vi "01 Wilt SM.vi"() -> ()   [LabVIEW 2012]
uses:
  Dryer.ctl
  Dryer Details.ctl
  Agilent Channel Definition.ctl
  Dryer Com Port Info.ctl
  Dryer Status Ctrl.ctl
  Dryer Test State.ctl
  <vilib>/Platform/fileVersionInfo.llb/FileVersionInformation.ctl
  Update Wilt GUI Control.ctl
  GEA2 Driver/GEA2 Dryer Interface Ctrl.ctl
  Dryer Commands.ctl
  <vilib>/Utility/file.llb/Write To Spreadsheet File (DBL).vi
  <vilib>/Utility/file.llb/Read From Spreadsheet File (DBL).vi
  Globals Wilt.vi
panel:
  out "Number of Units":i32
  in  "Emergency Timer":i32[](array[numeric])
  in  "Agilent Data":dbl[](array[numeric])
  in  "All Test Stations Control":T1[](array[typedef]) {"Night Cycle Count" format="%04d"; "Dryer Details"."Stop Dryer" items=["NO", "YES"]; "Dryer Details"."24 Hour Water Injection" items=["NO", "YES"]; "Dryer Details"."Run w/o Newfi" items=["NO", "YES"]; "Day Cycle Count" format="%04d"}
  in  "Pause Timer":i32[](array[numeric])
  in  "Agilent Channels Water Valves.":T3[](array[typedef])
  in  "Start Buttons.":T3[](array[typedef])
  out "Elapsed Time.":dbl format="%<%H:%M:%S>t"
  in  "Back Button":bool
  in  "Settings":bool
  in  "Tab Control 2":enum32{"Configuration", "Main"}(tab)
  in  "Tab Control":T4(tab)=enum."Directories"
  in  "DAQ Delay":u32=1000
  out "All Confgured Com Array":u8[](array[numeric])=[100, 2, 3, 4, 5, 6, 7, 8, 9, 10, 11, 12, 13, 14, 15, 16, 17, 18, 19, 20, 21, 22, 23, 24, 25, 26, 27, 28, 29, 30, 31, 32, 33, 34, 35, 36, 37, 38, 39, 40, 41, 42, 43, 44, 45, 46, 47, 48, 49, 50, 51, 52, 53, 54, 55, 56]
  out "Test Complete":bool
  in  "USB6008":tag="Dev2/port0"
  in  "Resend Start Limit":dbl=60.0
  in  "Wait Com Timer":dbl=15.0
  in  "Cooldown time":dbl=30.0
  out "Remote Station":bool
  out "Startup Coms":refnum<visa-resource-name>[](array[refnum])
  in  "Station Com List":u8[](array[numeric])
  out "All Test Stations":T1[](array[typedef]) {"Night Cycle Count" format="%04d"; "Dryer Details"."Stop Dryer" items=["NO", "YES"]; "Dryer Details"."24 Hour Water Injection" items=["NO", "YES"]; "Dryer Details"."Run w/o Newfi" items=["NO", "YES"]; "Day Cycle Count" format="%04d"}
  out "Dryer Com Info":T5[](array[typedef])=[{"Color"=0, "Last Read Status"=enum."Cycle Not Started", "Command:Data"="", "Com Port"=0, "Time(S)"=0.0, "Err Count"=0}, {"Color"=0, "Last Read Status"=enum."Cycle Not Started", "Command:Data"="", "Com Port"=0, "Time(S)"=0.0, "Err Count"=0}, {"Color"=0, "Last Read Status"=enum."Cycle Not Started", "Command:Data"="", "Com Port"=0, "Time(S)"=0.0, "Err Count"=0}, {"Color"=0, "Last Read Status"=enum."Cycle Not Started", "Command:Data"="", "Com Port"=0, "Time(S)"=0.0, "Err Count"=0}, {"Color"=0, "Last Read Status"=enum."Cycle Not Started", "Command:Data"="", "Com Port"=0, "Time(S)"=0.0, "Err Count"=0}, {"Color"=0, "Last Read Status"=enum."Cycle Not Started", "Command:Data"="", "Com Port"=0, "Time(S)"=0.0, "Err Count"=0}, {"Color"=0, "Last Read Status"=enum."Cycle Not Started", "Command:Data"="", "Com Port"=0, "Time(S)"=0.0, "Err Count"=0}, {"Color"=0, "Last Read Status"=enum."Cycle Not Started", "Command:Data"="", "Com Port"=0, "Time(S)"=0.0, "Err Count"=0}, {"Color"=0, "Last Read Status"=enum."Cycle Not Started", "Command:Data"="", "Com Port"=0, "Time(S)"=0.0, "Err Count"=0}, {"Color"=0, "Last Read Status"=enum."Cycle Not Started", "Command:Data"="", "Com Port"=0, "Time(S)"=0.0, "Err Count"=0}, {"Color"=0, "Last Read Status"=enum."Cycle Not Started", "Command:Data"="", "Com Port"=0, "Time(S)"=0.0, "Err Count"=0}, {"Color"=0, "Last Read Status"=enum."Cycle Not Started", "Command:Data"="", "Com Port"=0, "Time(S)"=0.0, "Err Count"=0}, {"Color"=0, "Last Read Status"=enum."Cycle Not Started", "Command:Data"="", "Com Port"=0, "Time(S)"=0.0, "Err Count"=0}, {"Color"=0, "Last Read Status"=enum."Cycle Not Started", "Command:Data"="", "Com Port"=0, "Time(S)"=0.0, "Err Count"=0}, {"Color"=0, "Last Read Status"=enum."Cycle Not Started", "Command:Data"="", "Com Port"=0, "Time(S)"=0.0, "Err Count"=0}, {"Color"=0, "Last Read Status"=enum."Cycle Not Started", "Command:Data"="", "Com Port"=0, "Time(S)"=0.0, "Err Count"=0}, {"Color"=0, "Last Read Status"=enum."Cycle Not Started", "Command:Data"="", "Com Port"=0, "Time(S)"=0.0, "Err Count"=0}, {"Color"=0, "Last Read Status"=enum."Cycle Not Started", "Command:Data"="", "Com Port"=0, "Time(S)"=0.0, "Err Count"=0}, {"Color"=0, "Last Read Status"=enum."Cycle Not Started", "Command:Data"="", "Com Port"=0, "Time(S)"=0.0, "Err Count"=0}, {"Color"=0, "Last Read Status"=enum."Cycle Not Started", "Command:Data"="", "Com Port"=0, "Time(S)"=0.0, "Err Count"=0}, {"Color"=0, "Last Read Status"=enum."Cycle Not Started", "Command:Data"="", "Com Port"=0, "Time(S)"=0.0, "Err Count"=0}, {"Color"=0, "Last Read Status"=enum."Cycle Not Started", "Command:Data"="", "Com Port"=0, "Time(S)"=0.0, "Err Count"=0}, {"Color"=0, "Last Read Status"=enum."Cycle Not Started", "Command:Data"="", "Com Port"=0, "Time(S)"=0.0, "Err Count"=0}, {"Color"=0, "Last Read Status"=enum."Cycle Not Started", "Command:Data"="", "Com Port"=0, "Time(S)"=0.0, "Err Count"=0}, {"Color"=0, "Last Read Status"=enum."Cycle Not Started", "Command:Data"="", "Com Port"=0, "Time(S)"=0.0, "Err Count"=0}, {"Color"=0, "Last Read Status"=enum."Cycle Not Started", "Command:Data"="", "Com Port"=0, "Time(S)"=0.0, "Err Count"=0}, {"Color"=0, "Last Read Status"=enum."Cycle Not Started", "Command:Data"="", "Com Port"=0, "Time(S)"=0.0, "Err Count"=0}, {"Color"=0, "Last Read Status"=enum."Cycle Not Started", "Command:Data"="", "Com Port"=0, "Time(S)"=0.0, "Err Count"=0}, {"Color"=0, "Last Read Status"=enum."Cycle Not Started", "Command:Data"="", "Com Port"=0, "Time(S)"=0.0, "Err Count"=0}, {"Color"=0, "Last Read Status"=enum."Cycle Not Started", "Command:Data"="", "Com Port"=0, "Time(S)"=0.0, "Err Count"=0}, {"Color"=0, "Last Read Status"=enum."Cycle Not Started", "Command:Data"="", "Com Port"=0, "Time(S)"=0.0, "Err Count"=0}, {"Color"=0, "Last Read Status"=enum."Cycle Not Started", "Command:Data"="", "Com Port"=0, "Time(S)"=0.0, "Err Count"=0}, {"Color"=0, "Last Read Status"=enum."Cycle Not Started", "Command:Data"="", "Com Port"=0, "Time(S)"=0.0, "Err Count"=0}, {"Color"=0, "Last Read Status"=enum."Cycle Not Started", "Command:Data"="", "Com Port"=0, "Time(S)"=0.0, "Err Count"=0}, {"Color"=0, "Last Read Status"=enum."Cycle Not Started", "Command:Data"="", "Com Port"=0, "Time(S)"=0.0, "Err Count"=0}, {"Color"=0, "Last Read Status"=enum."Cycle Not Started", "Command:Data"="", "Com Port"=0, "Time(S)"=0.0, "Err Count"=0}, {"Color"=0, "Last Read Status"=enum."Cycle Not Started", "Command:Data"="", "Com Port"=0, "Time(S)"=0.0, "Err Count"=0}, {"Color"=0, "Last Read Status"=enum."Cycle Not Started", "Command:Data"="", "Com Port"=0, "Time(S)"=0.0, "Err Count"=0}, {"Color"=0, "Last Read Status"=enum."Cycle Not Started", "Command:Data"="", "Com Port"=0, "Time(S)"=0.0, "Err Count"=0}, {"Color"=0, "Last Read Status"=enum."Cycle Not Started", "Command:Data"="", "Com Port"=0, "Time(S)"=0.0, "Err Count"=0}, {"Color"=0, "Last Read Status"=enum."Cycle Not Started", "Command:Data"="", "Com Port"=0, "Time(S)"=0.0, "Err Count"=0}, {"Color"=0, "Last Read Status"=enum."Cycle Not Started", "Command:Data"="", "Com Port"=0, "Time(S)"=0.0, "Err Count"=0}, {"Color"=0, "Last Read Status"=enum."Cycle Not Started", "Command:Data"="", "Com Port"=0, "Time(S)"=0.0, "Err Count"=0}, {"Color"=0, "Last Read Status"=enum."Cycle Not Started", "Command:Data"="", "Com Port"=0, "Time(S)"=0.0, "Err Count"=0}, {"Color"=0, "Last Read Status"=enum."Cycle Not Started", "Command:Data"="", "Com Port"=0, "Time(S)"=0.0, "Err Count"=0}, {"Color"=0, "Last Read Status"=enum."Cycle Not Started", "Command:Data"="", "Com Port"=0, "Time(S)"=0.0, "Err Count"=0}, {"Color"=0, "Last Read Status"=enum."Cycle Not Started", "Command:Data"="", "Com Port"=0, "Time(S)"=0.0, "Err Count"=0}, {"Color"=0, "Last Read Status"=enum."Cycle Not Started", "Command:Data"="", "Com Port"=0, "Time(S)"=0.0, "Err Count"=0}, {"Color"=0, "Last Read Status"=enum."Cycle Not Started", "Command:Data"="", "Com Port"=0, "Time(S)"=0.0, "Err Count"=0}, {"Color"=0, "Last Read Status"=enum."Cycle Not Started", "Command:Data"="", "Com Port"=0, "Time(S)"=0.0, "Err Count"=0}, {"Color"=0, "Last Read Status"=enum."Cycle Not Started", "Command:Data"="", "Com Port"=0, "Time(S)"=0.0, "Err Count"=0}, {"Color"=0, "Last Read Status"=enum."Cycle Not Started", "Command:Data"="", "Com Port"=0, "Time(S)"=0.0, "Err Count"=0}, {"Color"=0, "Last Read Status"=enum."Cycle Not Started", "Command:Data"="", "Com Port"=0, "Time(S)"=0.0, "Err Count"=0}, {"Color"=0, "Last Read Status"=enum."Cycle Not Started", "Command:Data"="", "Com Port"=0, "Time(S)"=0.0, "Err Count"=0}, {"Color"=0, "Last Read Status"=enum."Cycle Not Started", "Command:Data"="", "Com Port"=0, "Time(S)"=0.0, "Err Count"=0}, {"Color"=0, "Last Read Status"=enum."Cycle Not Started", "Command:Data"="", "Com Port"=0, "Time(S)"=0.0, "Err Count"=0}, {"Color"=0, "Last Read Status"=enum."Cycle Not Started", "Command:Data"="", "Com Port"=0, "Time(S)"=0.0, "Err Count"=0}, {"Color"=0, "Last Read Status"=enum."Cycle Not Started", "Command:Data"="", "Com Port"=0, "Time(S)"=0.0, "Err Count"=0}, {"Color"=0, "Last Read Status"=enum."Cycle Not Started", "Command:Data"="", "Com Port"=0, "Time(S)"=0.0, "Err Count"=0}, {"Color"=0, "Last Read Status"=enum."Cycle Not Started", "Command:Data"="", "Com Port"=0, "Time(S)"=0.0, "Err Count"=0}, {"Color"=0, "Last Read Status"=enum."Cycle Not Started", "Command:Data"="", "Com Port"=0, "Time(S)"=0.0, "Err Count"=0}, {"Color"=0, "Last Read Status"=enum."Cycle Not Started", "Command:Data"="", "Com Port"=0, "Time(S)"=0.0, "Err Count"=0}, {"Color"=0, "Last Read Status"=enum."Cycle Not Started", "Command:Data"="", "Com Port"=0, "Time(S)"=0.0, "Err Count"=0}, {"Color"=0, "Last Read Status"=enum."Cycle Not Started", "Command:Data"="", "Com Port"=0, "Time(S)"=0.0, "Err Count"=0}, {"Color"=0, "Last Read Status"=enum."Cycle Not Started", "Command:Data"="", "Com Port"=0, "Time(S)"=0.0, "Err Count"=0}, {"Color"=0, "Last Read Status"=enum."Cycle Not Started", "Command:Data"="", "Com Port"=0, "Time(S)"=0.0, "Err Count"=0}, {"Color"=0, "Last Read Status"=enum."Cycle Not Started", "Command:Data"="", "Com Port"=0, "Time(S)"=0.0, "Err Count"=0}, {"Color"=0, "Last Read Status"=enum."Cycle Not Started", "Command:Data"="", "Com Port"=0, "Time(S)"=0.0, "Err Count"=0}, {"Color"=0, "Last Read Status"=enum."Cycle Not Started", "Command:Data"="", "Com Port"=0, "Time(S)"=0.0, "Err Count"=0}, {"Color"=0, "Last Read Status"=enum."Cycle Not Started", "Command:Data"="", "Com Port"=0, "Time(S)"=0.0, "Err Count"=0}, {"Color"=0, "Last Read Status"=enum."Cycle Not Started", "Command:Data"="", "Com Port"=0, "Time(S)"=0.0, "Err Count"=0}, {"Color"=0, "Last Read Status"=enum."Cycle Not Started", "Command:Data"="", "Com Port"=0, "Time(S)"=0.0, "Err Count"=0}, {"Color"=0, "Last Read Status"=enum."Cycle Not Started", "Command:Data"="", "Com Port"=0, "Time(S)"=0.0, "Err Count"=0}, {"Color"=0, "Last Read Status"=enum."Cycle Not Started", "Command:Data"="", "Com Port"=0, "Time(S)"=0.0, "Err Count"=0}, {"Color"=0, "Last Read Status"=enum."Cycle Not Started", "Command:Data"="", "Com Port"=0, "Time(S)"=0.0, "Err Count"=0}, {"Color"=0, "Last Read Status"=enum."Cycle Not Started", "Command:Data"="", "Com Port"=0, "Time(S)"=0.0, "Err Count"=0}, {"Color"=0, "Last Read Status"=enum."Cycle Not Started", "Command:Data"="", "Com Port"=0, "Time(S)"=0.0, "Err Count"=0}, {"Color"=0, "Last Read Status"=enum."Cycle Not Started", "Command:Data"="", "Com Port"=0, "Time(S)"=0.0, "Err Count"=0}, {"Color"=0, "Last Read Status"=enum."Cycle Not Started", "Command:Data"="", "Com Port"=0, "Time(S)"=0.0, "Err Count"=0}, {"Color"=0, "Last Read Status"=enum."Cycle Not Started", "Command:Data"="", "Com Port"=0, "Time(S)"=0.0, "Err Count"=0}, {"Color"=0, "Last Read Status"=enum."Cycle Not Started", "Command:Data"="", "Com Port"=0, "Time(S)"=0.0, "Err Count"=0}, {"Color"=0, "Last Read Status"=enum."Cycle Not Started", "Command:Data"="", "Com Port"=0, "Time(S)"=0.0, "Err Count"=0}, {"Color"=0, "Last Read Status"=enum."Cycle Not Started", "Command:Data"="", "Com Port"=0, "Time(S)"=0.0, "Err Count"=0}, {"Color"=0, "Last Read Status"=enum."Cycle Not Started", "Command:Data"="", "Com Port"=0, "Time(S)"=0.0, "Err Count"=0}, {"Color"=0, "Last Read Status"=enum."Cycle Not Started", "Command:Data"="", "Com Port"=0, "Time(S)"=0.0, "Err Count"=0}, {"Color"=0, "Last Read Status"=enum."Cycle Not Started", "Command:Data"="", "Com Port"=0, "Time(S)"=0.0, "Err Count"=0}, {"Color"=0, "Last Read Status"=enum."Cycle Not Started", "Command:Data"="", "Com Port"=0, "Time(S)"=0.0, "Err Count"=0}, {"Color"=0, "Last Read Status"=enum."Cycle Not Started", "Command:Data"="", "Com Port"=0, "Time(S)"=0.0, "Err Count"=0}, {"Color"=0, "Last Read Status"=enum."Cycle Not Started", "Command:Data"="", "Com Port"=0, "Time(S)"=0.0, "Err Count"=0}, {"Color"=0, "Last Read Status"=enum."Cycle Not Started", "Command:Data"="", "Com Port"=0, "Time(S)"=0.0, "Err Count"=0}, {"Color"=0, "Last Read Status"=enum."Cycle Not Started", "Command:Data"="", "Com Port"=0, "Time(S)"=0.0, "Err Count"=0}, {"Color"=0, "Last Read Status"=enum."Cycle Not Started", "Command:Data"="", "Com Port"=0, "Time(S)"=0.0, "Err Count"=0}, {"Color"=0, "Last Read Status"=enum."Cycle Not Started", "Command:Data"="", "Com Port"=0, "Time(S)"=0.0, "Err Count"=0}, {"Color"=0, "Last Read Status"=enum."Cycle Not Started", "Command:Data"="", "Com Port"=0, "Time(S)"=0.0, "Err Count"=0}, {"Color"=0, "Last Read Status"=enum."Cycle Not Started", "Command:Data"="", "Com Port"=0, "Time(S)"=0.0, "Err Count"=0}, {"Color"=0, "Last Read Status"=enum."Cycle Not Started", "Command:Data"="", "Com Port"=0, "Time(S)"=0.0, "Err Count"=0}, {"Color"=0, "Last Read Status"=enum."Cycle Not Started", "Command:Data"="", "Com Port"=0, "Time(S)"=0.0, "Err Count"=0}, {"Color"=0, "Last Read Status"=enum."Cycle Not Started", "Command:Data"="", "Com Port"=0, "Time(S)"=0.0, "Err Count"=0}, {"Color"=0, "Last Read Status"=enum."Cycle Not Started", "Command:Data"="", "Com Port"=0, "Time(S)"=0.0, "Err Count"=0}, {"Color"=0, "Last Read Status"=enum."Cycle Not Started", "Command:Data"="", "Com Port"=0, "Time(S)"=0.0, "Err Count"=0}, {"Color"=0, "Last Read Status"=enum."Cycle Not Started", "Command:Data"="", "Com Port"=0, "Time(S)"=0.0, "Err Count"=0}, {"Color"=0, "Last Read Status"=enum."Cycle Not Started", "Command:Data"="", "Com Port"=0, "Time(S)"=0.0, "Err Count"=0}, {"Color"=0, "Last Read Status"=enum."Cycle Not Started", "Command:Data"="", "Com Port"=0, "Time(S)"=0.0, "Err Count"=0}, {"Color"=0, "Last Read Status"=enum."Cycle Not Started", "Command:Data"="", "Com Port"=0, "Time(S)"=0.0, "Err Count"=0}, {"Color"=0, "Last Read Status"=enum."Cycle Not Started", "Command:Data"="", "Com Port"=0, "Time(S)"=0.0, "Err Count"=0}, {"Color"=0, "Last Read Status"=enum."Cycle Not Started", "Command:Data"="", "Com Port"=0, "Time(S)"=0.0, "Err Count"=0}, {"Color"=0, "Last Read Status"=enum."Cycle Not Started", "Command:Data"="", "Com Port"=0, "Time(S)"=0.0, "Err Count"=0}, {"Color"=0, "Last Read Status"=enum."Cycle Not Started", "Command:Data"="", "Com Port"=0, "Time(S)"=0.0, "Err Count"=0}, {"Color"=0, "Last Read Status"=enum."Cycle Not Started", "Command:Data"="", "Com Port"=0, "Time(S)"=0.0, "Err Count"=0}, {"Color"=0, "Last Read Status"=enum."Cycle Not Started", "Command:Data"="", "Com Port"=0, "Time(S)"=0.0, "Err Count"=0}, {"Color"=0, "Last Read Status"=enum."Cycle Not Started", "Command:Data"="", "Com Port"=0, "Time(S)"=0.0, "Err Count"=0}, {"Color"=0, "Last Read Status"=enum."Cycle Not Started", "Command:Data"="", "Com Port"=0, "Time(S)"=0.0, "Err Count"=0}, {"Color"=0, "Last Read Status"=enum."Cycle Not Started", "Command:Data"="", "Com Port"=0, "Time(S)"=0.0, "Err Count"=0}, {"Color"=0, "Last Read Status"=enum."Cycle Not Started", "Command:Data"="", "Com Port"=0, "Time(S)"=0.0, "Err Count"=0}, {"Color"=0, "Last Read Status"=enum."Cycle Not Started", "Command:Data"="", "Com Port"=0, "Time(S)"=0.0, "Err Count"=0}, {"Color"=0, "Last Read Status"=enum."Cycle Not Started", "Command:Data"="", "Com Port"=0, "Time(S)"=0.0, "Err Count"=0}, {"Color"=0, "Last Read Status"=enum."Cycle Not Started", "Command:Data"="", "Com Port"=0, "Time(S)"=0.0, "Err Count"=0}, {"Color"=0, "Last Read Status"=enum."Cycle Not Started", "Command:Data"="", "Com Port"=0, "Time(S)"=0.0, "Err Count"=0}, {"Color"=0, "Last Read Status"=enum."Cycle Not Started", "Command:Data"="", "Com Port"=0, "Time(S)"=0.0, "Err Count"=0}, {"Color"=0, "Last Read Status"=enum."Cycle Not Started", "Command:Data"="", "Com Port"=0, "Time(S)"=0.0, "Err Count"=0}, {"Color"=0, "Last Read Status"=enum."Cycle Not Started", "Command:Data"="", "Com Port"=0, "Time(S)"=0.0, "Err Count"=0}, {"Color"=0, "Last Read Status"=enum."Cycle Not Started", "Command:Data"="", "Com Port"=0, "Time(S)"=0.0, "Err Count"=0}, {"Color"=0, "Last Read Status"=enum."Cycle Not Started", "Command:Data"="", "Com Port"=0, "Time(S)"=0.0, "Err Count"=0}, {"Color"=0, "Last Read Status"=enum."Cycle Not Started", "Command:Data"="", "Com Port"=0, "Time(S)"=0.0, "Err Count"=0}, {"Color"=0, "Last Read Status"=enum."Cycle Not Started", "Command:Data"="", "Com Port"=0, "Time(S)"=0.0, "Err Count"=0}, {"Color"=0, "Last Read Status"=enum."Cycle Not Started", "Command:Data"="", "Com Port"=0, "Time(S)"=0.0, "Err Count"=0}, {"Color"=0, "Last Read Status"=enum."Cycle Not Started", "Command:Data"="", "Com Port"=0, "Time(S)"=0.0, "Err Count"=0}, {"Color"=0, "Last Read Status"=enum."Cycle Not Started", "Command:Data"="", "Com Port"=0, "Time(S)"=0.0, "Err Count"=0}, {"Color"=0, "Last Read Status"=enum."Cycle Not Started", "Command:Data"="", "Com Port"=0, "Time(S)"=0.0, "Err Count"=0}, {"Color"=0, "Last Read Status"=enum."Cycle Not Started", "Command:Data"="", "Com Port"=0, "Time(S)"=0.0, "Err Count"=0}, {"Color"=0, "Last Read Status"=enum."Cycle Not Started", "Command:Data"="", "Com Port"=0, "Time(S)"=0.0, "Err Count"=0}, {"Color"=0, "Last Read Status"=enum."Cycle Not Started", "Command:Data"="", "Com Port"=0, "Time(S)"=0.0, "Err Count"=0}, {"Color"=0, "Last Read Status"=enum."Cycle Not Started", "Command:Data"="", "Com Port"=0, "Time(S)"=0.0, "Err Count"=0}, {"Color"=0, "Last Read Status"=enum."Cycle Not Started", "Command:Data"="", "Com Port"=0, "Time(S)"=0.0, "Err Count"=0}, {"Color"=0, "Last Read Status"=enum."Cycle Not Started", "Command:Data"="", "Com Port"=0, "Time(S)"=0.0, "Err Count"=0}, {"Color"=0, "Last Read Status"=enum."Cycle Not Started", "Command:Data"="", "Com Port"=0, "Time(S)"=0.0, "Err Count"=0}, {"Color"=0, "Last Read Status"=enum."Cycle Not Started", "Command:Data"="", "Com Port"=0, "Time(S)"=0.0, "Err Count"=0}, {"Color"=0, "Last Read Status"=enum."Cycle Not Started", "Command:Data"="", "Com Port"=0, "Time(S)"=0.0, "Err Count"=0}, {"Color"=0, "Last Read Status"=enum."Cycle Not Started", "Command:Data"="", "Com Port"=0, "Time(S)"=0.0, "Err Count"=0}, {"Color"=0, "Last Read Status"=enum."Cycle Not Started", "Command:Data"="", "Com Port"=0, "Time(S)"=0.0, "Err Count"=0}, {"Color"=0, "Last Read Status"=enum."Cycle Not Started", "Command:Data"="", "Com Port"=0, "Time(S)"=0.0, "Err Count"=0}, {"Color"=0, "Last Read Status"=enum."Cycle Not Started", "Command:Data"="", "Com Port"=0, "Time(S)"=0.0, "Err Count"=0}, {"Color"=0, "Last Read Status"=enum."Cycle Not Started", "Command:Data"="", "Com Port"=0, "Time(S)"=0.0, "Err Count"=0}, {"Color"=0, "Last Read Status"=enum."Cycle Not Started", "Command:Data"="", "Com Port"=0, "Time(S)"=0.0, "Err Count"=0}, {"Color"=0, "Last Read Status"=enum."Cycle Not Started", "Command:Data"="", "Com Port"=0, "Time(S)"=0.0, "Err Count"=0}, {"Color"=0, "Last Read Status"=enum."Cycle Not Started", "Command:Data"="", "Com Port"=0, "Time(S)"=0.0, "Err Count"=0}, {"Color"=0, "Last Read Status"=enum."Cycle Not Started", "Command:Data"="", "Com Port"=0, "Time(S)"=0.0, "Err Count"=0}, {"Color"=0, "Last Read Status"=enum."Cycle Not Started", "Command:Data"="", "Com Port"=0, "Time(S)"=0.0, "Err Count"=0}, {"Color"=0, "Last Read Status"=enum."Cycle Not Started", "Command:Data"="", "Com Port"=0, "Time(S)"=0.0, "Err Count"=0}, {"Color"=0, "Last Read Status"=enum."Cycle Not Started", "Command:Data"="", "Com Port"=0, "Time(S)"=0.0, "Err Count"=0}, {"Color"=0, "Last Read Status"=enum."Cycle Not Started", "Command:Data"="", "Com Port"=0, "Time(S)"=0.0, "Err Count"=0}, {"Color"=0, "Last Read Status"=enum."Cycle Not Started", "Command:Data"="", "Com Port"=0, "Time(S)"=0.0, "Err Count"=0}, {"Color"=0, "Last Read Status"=enum."Cycle Not Started", "Command:Data"="", "Com Port"=0, "Time(S)"=0.0, "Err Count"=0}, {"Color"=0, "Last Read Status"=enum."Cycle Not Started", "Command:Data"="", "Com Port"=0, "Time(S)"=0.0, "Err Count"=0}, {"Color"=0, "Last Read Status"=enum."Cycle Not Started", "Command:Data"="", "Com Port"=0, "Time(S)"=0.0, "Err Count"=0}, {"Color"=0, "Last Read Status"=enum."Cycle Not Started", "Command:Data"="", "Com Port"=0, "Time(S)"=0.0, "Err Count"=0}, {"Color"=0, "Last Read Status"=enum."Cycle Not Started", "Command:Data"="", "Com Port"=0, "Time(S)"=0.0, "Err Count"=0}, {"Color"=0, "Last Read Status"=enum."Cycle Not Started", "Command:Data"="", "Com Port"=0, "Time(S)"=0.0, "Err Count"=0}, {"Color"=0, "Last Read Status"=enum."Cycle Not Started", "Command:Data"="", "Com Port"=0, "Time(S)"=0.0, "Err Count"=0}, {"Color"=0, "Last Read Status"=enum."Cycle Not Started", "Command:Data"="", "Com Port"=0, "Time(S)"=0.0, "Err Count"=0}, {"Color"=0, "Last Read Status"=enum."Cycle Not Started", "Command:Data"="", "Com Port"=0, "Time(S)"=0.0, "Err Count"=0}, {"Color"=0, "Last Read Status"=enum."Cycle Not Started", "Command:Data"="", "Com Port"=0, "Time(S)"=0.0, "Err Count"=0}, {"Color"=0, "Last Read Status"=enum."Cycle Not Started", "Command:Data"="", "Com Port"=0, "Time(S)"=0.0, "Err Count"=0}, {"Color"=0, "Last Read Status"=enum."Cycle Not Started", "Command:Data"="", "Com Port"=0, "Time(S)"=0.0, "Err Count"=0}, {"Color"=0, "Last Read Status"=enum."Cycle Not Started", "Command:Data"="", "Com Port"=0, "Time(S)"=0.0, "Err Count"=0}, {"Color"=0, "Last Read Status"=enum."Cycle Not Started", "Command:Data"="", "Com Port"=0, "Time(S)"=0.0, "Err Count"=0}, {"Color"=0, "Last Read Status"=enum."Cycle Not Started", "Command:Data"="", "Com Port"=0, "Time(S)"=0.0, "Err Count"=0}, {"Color"=0, "Last Read Status"=enum."Cycle Not Started", "Command:Data"="", "Com Port"=0, "Time(S)"=0.0, "Err Count"=0}, {"Color"=0, "Last Read Status"=enum."Cycle Not Started", "Command:Data"="", "Com Port"=0, "Time(S)"=0.0, "Err Count"=0}, {"Color"=0, "Last Read Status"=enum."Cycle Not Started", "Command:Data"="", "Com Port"=0, "Time(S)"=0.0, "Err Count"=0}, {"Color"=0, "Last Read Status"=enum."Cycle Not Started", "Command:Data"="", "Com Port"=0, "Time(S)"=0.0, "Err Count"=0}, {"Color"=0, "Last Read Status"=enum."Cycle Not Started", "Command:Data"="", "Com Port"=0, "Time(S)"=0.0, "Err Count"=0}, {"Color"=0, "Last Read Status"=enum."Cycle Not Started", "Command:Data"="", "Com Port"=0, "Time(S)"=0.0, "Err Count"=0}, {"Color"=0, "Last Read Status"=enum."Cycle Not Started", "Command:Data"="", "Com Port"=0, "Time(S)"=0.0, "Err Count"=0}, {"Color"=0, "Last Read Status"=enum."Cycle Not Started", "Command:Data"="", "Com Port"=0, "Time(S)"=0.0, "Err Count"=0}, {"Color"=0, "Last Read Status"=enum."Cycle Not Started", "Command:Data"="", "Com Port"=0, "Time(S)"=0.0, "Err Count"=0}, {"Color"=0, "Last Read Status"=enum."Cycle Not Started", "Command:Data"="", "Com Port"=0, "Time(S)"=0.0, "Err Count"=0}, {"Color"=0, "Last Read Status"=enum."Cycle Not Started", "Command:Data"="", "Com Port"=0, "Time(S)"=0.0, "Err Count"=0}, {"Color"=0, "Last Read Status"=enum."Cycle Not Started", "Command:Data"="", "Com Port"=0, "Time(S)"=0.0, "Err Count"=0}, {"Color"=0, "Last Read Status"=enum."Cycle Not Started", "Command:Data"="", "Com Port"=0, "Time(S)"=0.0, "Err Count"=0}, {"Color"=0, "Last Read Status"=enum."Cycle Not Started", "Command:Data"="", "Com Port"=0, "Time(S)"=0.0, "Err Count"=0}, {"Color"=0, "Last Read Status"=enum."Cycle Not Started", "Command:Data"="", "Com Port"=0, "Time(S)"=0.0, "Err Count"=0}, {"Color"=0, "Last Read Status"=enum."Cycle Not Started", "Command:Data"="", "Com Port"=0, "Time(S)"=0.0, "Err Count"=0}, {"Color"=0, "Last Read Status"=enum."Cycle Not Started", "Command:Data"="", "Com Port"=0, "Time(S)"=0.0, "Err Count"=0}, {"Color"=0, "Last Read Status"=enum."Cycle Not Started", "Command:Data"="", "Com Port"=0, "Time(S)"=0.0, "Err Count"=0}, {"Color"=0, "Last Read Status"=enum."Cycle Not Started", "Command:Data"="", "Com Port"=0, "Time(S)"=0.0, "Err Count"=0}, {"Color"=0, "Last Read Status"=enum."Cycle Not Started", "Command:Data"="", "Com Port"=0, "Time(S)"=0.0, "Err Count"=0}, {"Color"=0, "Last Read Status"=enum."Cycle Not Started", "Command:Data"="", "Com Port"=0, "Time(S)"=0.0, "Err Count"=0}, {"Color"=0, "Last Read Status"=enum."Cycle Not Started", "Command:Data"="", "Com Port"=0, "Time(S)"=0.0, "Err Count"=0}, {"Color"=0, "Last Read Status"=enum."Cycle Not Started", "Command:Data"="", "Com Port"=0, "Time(S)"=0.0, "Err Count"=0}, {"Color"=0, "Last Read Status"=enum."Cycle Not Started", "Command:Data"="", "Com Port"=0, "Time(S)"=0.0, "Err Count"=0}, {"Color"=0, "Last Read Status"=enum."Cycle Not Started", "Command:Data"="", "Com Port"=0, "Time(S)"=0.0, "Err Count"=0}, {"Color"=0, "Last Read Status"=enum."Cycle Not Started", "Command:Data"="", "Com Port"=0, "Time(S)"=0.0, "Err Count"=0}, {"Color"=0, "Last Read Status"=enum."Cycle Not Started", "Command:Data"="", "Com Port"=0, "Time(S)"=0.0, "Err Count"=0}, {"Color"=0, "Last Read Status"=enum."Cycle Not Started", "Command:Data"="", "Com Port"=0, "Time(S)"=0.0, "Err Count"=0}, {"Color"=0, "Last Read Status"=enum."Cycle Not Started", "Command:Data"="", "Com Port"=0, "Time(S)"=0.0, "Err Count"=0}, {"Color"=0, "Last Read Status"=enum."Cycle Not Started", "Command:Data"="", "Com Port"=0, "Time(S)"=0.0, "Err Count"=0}, {"Color"=0, "Last Read Status"=enum."Cycle Not Started", "Command:Data"="", "Com Port"=0, "Time(S)"=0.0, "Err Count"=0}, {"Color"=0, "Last Read Status"=enum."Cycle Not Started", "Command:Data"="", "Com Port"=0, "Time(S)"=0.0, "Err Count"=0}, {"Color"=0, "Last Read Status"=enum."Cycle Not Started", "Command:Data"="", "Com Port"=0, "Time(S)"=0.0, "Err Count"=0}, {"Color"=0, "Last Read Status"=enum."Cycle Not Started", "Command:Data"="", "Com Port"=0, "Time(S)"=0.0, "Err Count"=0}, {"Color"=0, "Last Read Status"=enum."Cycle Not Started", "Command:Data"="", "Com Port"=0, "Time(S)"=0.0, "Err Count"=0}, {"Color"=0, "Last Read Status"=enum."Cycle Not Started", "Command:Data"="", "Com Port"=0, "Time(S)"=0.0, "Err Count"=0}, {"Color"=0, "Last Read Status"=enum."Cycle Not Started", "Command:Data"="", "Com Port"=0, "Time(S)"=0.0, "Err Count"=0}, {"Color"=0, "Last Read Status"=enum."Cycle Not Started", "Command:Data"="", "Com Port"=0, "Time(S)"=0.0, "Err Count"=0}, {"Color"=0, "Last Read Status"=enum."Cycle Not Started", "Command:Data"="", "Com Port"=0, "Time(S)"=0.0, "Err Count"=0}, {"Color"=0, "Last Read Status"=enum."Cycle Not Started", "Command:Data"="", "Com Port"=0, "Time(S)"=0.0, "Err Count"=0}, {"Color"=0, "Last Read Status"=enum."Cycle Not Started", "Command:Data"="", "Com Port"=0, "Time(S)"=0.0, "Err Count"=0}, {"Color"=0, "Last Read Status"=enum."Cycle Not Started", "Command:Data"="", "Com Port"=0, "Time(S)"=0.0, "Err Count"=0}, {"Color"=0, "Last Read Status"=enum."Cycle Not Started", "Command:Data"="", "Com Port"=0, "Time(S)"=0.0, "Err Count"=0}, {"Color"=0, "Last Read Status"=enum."Cycle Not Started", "Command:Data"="", "Com Port"=0, "Time(S)"=0.0, "Err Count"=0}, {"Color"=0, "Last Read Status"=enum."Cycle Not Started", "Command:Data"="", "Com Port"=0, "Time(S)"=0.0, "Err Count"=0}, {"Color"=0, "Last Read Status"=enum."Cycle Not Started", "Command:Data"="", "Com Port"=0, "Time(S)"=0.0, "Err Count"=0}, {"Color"=0, "Last Read Status"=enum."Cycle Not Started", "Command:Data"="", "Com Port"=0, "Time(S)"=0.0, "Err Count"=0}, {"Color"=0, "Last Read Status"=enum."Cycle Not Started", "Command:Data"="", "Com Port"=0, "Time(S)"=0.0, "Err Count"=0}, {"Color"=0, "Last Read Status"=enum."Cycle Not Started", "Command:Data"="", "Com Port"=0, "Time(S)"=0.0, "Err Count"=0}, {"Color"=0, "Last Read Status"=enum."Cycle Not Started", "Command:Data"="", "Com Port"=0, "Time(S)"=0.0, "Err Count"=0}, {"Color"=0, "Last Read Status"=enum."Cycle Not Started", "Command:Data"="", "Com Port"=0, "Time(S)"=0.0, "Err Count"=0}, {"Color"=0, "Last Read Status"=enum."Cycle Not Started", "Command:Data"="", "Com Port"=0, "Time(S)"=0.0, "Err Count"=0}, {"Color"=0, "Last Read Status"=enum."Cycle Not Started", "Command:Data"="", "Com Port"=0, "Time(S)"=0.0, "Err Count"=0}, {"Color"=0, "Last Read Status"=enum."Cycle Not Started", "Command:Data"="", "Com Port"=0, "Time(S)"=0.0, "Err Count"=0}, {"Color"=0, "Last Read Status"=enum."Cycle Not Started", "Command:Data"="", "Com Port"=0, "Time(S)"=0.0, "Err Count"=0}, {"Color"=0, "Last Read Status"=enum."Cycle Not Started", "Command:Data"="", "Com Port"=0, "Time(S)"=0.0, "Err Count"=0}, {"Color"=0, "Last Read Status"=enum."Cycle Not Started", "Command:Data"="", "Com Port"=0, "Time(S)"=0.0, "Err Count"=0}, {"Color"=0, "Last Read Status"=enum."Cycle Not Started", "Command:Data"="", "Com Port"=0, "Time(S)"=0.0, "Err Count"=0}, {"Color"=0, "Last Read Status"=enum."Cycle Not Started", "Command:Data"="", "Com Port"=0, "Time(S)"=0.0, "Err Count"=0}, {"Color"=0, "Last Read Status"=enum."Cycle Not Started", "Command:Data"="", "Com Port"=0, "Time(S)"=0.0, "Err Count"=0}, {"Color"=0, "Last Read Status"=enum."Cycle Not Started", "Command:Data"="", "Com Port"=0, "Time(S)"=0.0, "Err Count"=0}, {"Color"=0, "Last Read Status"=enum."Cycle Not Started", "Command:Data"="", "Com Port"=0, "Time(S)"=0.0, "Err Count"=0}, {"Color"=0, "Last Read Status"=enum."Cycle Not Started", "Command:Data"="", "Com Port"=0, "Time(S)"=0.0, "Err Count"=0}, {"Color"=0, "Last Read Status"=enum."Cycle Not Started", "Command:Data"="", "Com Port"=0, "Time(S)"=0.0, "Err Count"=0}, {"Color"=0, "Last Read Status"=enum."Cycle Not Started", "Command:Data"="", "Com Port"=0, "Time(S)"=0.0, "Err Count"=0}, {"Color"=0, "Last Read Status"=enum."Cycle Not Started", "Command:Data"="", "Com Port"=0, "Time(S)"=0.0, "Err Count"=0}, {"Color"=0, "Last Read Status"=enum."Cycle Not Started", "Command:Data"="", "Com Port"=0, "Time(S)"=0.0, "Err Count"=0}, {"Color"=0, "Last Read Status"=enum."Cycle Not Started", "Command:Data"="", "Com Port"=0, "Time(S)"=0.0, "Err Count"=0}, {"Color"=0, "Last Read Status"=enum."Cycle Not Started", "Command:Data"="", "Com Port"=0, "Time(S)"=0.0, "Err Count"=0}, {"Color"=0, "Last Read Status"=enum."Cycle Not Started", "Command:Data"="", "Com Port"=0, "Time(S)"=0.0, "Err Count"=0}, {"Color"=0, "Last Read Status"=enum."Cycle Not Started", "Command:Data"="", "Com Port"=0, "Time(S)"=0.0, "Err Count"=0}, {"Color"=0, "Last Read Status"=enum."Cycle Not Started", "Command:Data"="", "Com Port"=0, "Time(S)"=0.0, "Err Count"=0}, {"Color"=0, "Last Read Status"=enum."Cycle Not Started", "Command:Data"="", "Com Port"=0, "Time(S)"=0.0, "Err Count"=0}, {"Color"=0, "Last Read Status"=enum."Cycle Not Started", "Command:Data"="", "Com Port"=0, "Time(S)"=0.0, "Err Count"=0}, {"Color"=0, "Last Read Status"=enum."Cycle Not Started", "Command:Data"="", "Com Port"=0, "Time(S)"=0.0, "Err Count"=0}, {"Color"=0, "Last Read Status"=enum."Cycle Not Started", "Command:Data"="", "Com Port"=0, "Time(S)"=0.0, "Err Count"=0}, {"Color"=0, "Last Read Status"=enum."Cycle Not Started", "Command:Data"="", "Com Port"=0, "Time(S)"=0.0, "Err Count"=0}, {"Color"=0, "Last Read Status"=enum."Cycle Not Started", "Command:Data"="", "Com Port"=0, "Time(S)"=0.0, "Err Count"=0}, {"Color"=0, "Last Read Status"=enum."Cycle Not Started", "Command:Data"="", "Com Port"=0, "Time(S)"=0.0, "Err Count"=0}, {"Color"=0, "Last Read Status"=enum."Cycle Not Started", "Command:Data"="", "Com Port"=0, "Time(S)"=0.0, "Err Count"=0}, {"Color"=0, "Last Read Status"=enum."Cycle Not Started", "Command:Data"="", "Com Port"=0, "Time(S)"=0.0, "Err Count"=0}, {"Color"=0, "Last Read Status"=enum."Cycle Not Started", "Command:Data"="", "Com Port"=0, "Time(S)"=0.0, "Err Count"=0}, {"Color"=0, "Last Read Status"=enum."Cycle Not Started", "Command:Data"="", "Com Port"=0, "Time(S)"=0.0, "Err Count"=0}, {"Color"=0, "Last Read Status"=enum."Cycle Not Started", "Command:Data"="", "Com Port"=0, "Time(S)"=0.0, "Err Count"=0}, {"Color"=0, "Last Read Status"=enum."Cycle Not Started", "Command:Data"="", "Com Port"=0, "Time(S)"=0.0, "Err Count"=0}, {"Color"=0, "Last Read Status"=enum."Cycle Not Started", "Command:Data"="", "Com Port"=0, "Time(S)"=0.0, "Err Count"=0}, {"Color"=0, "Last Read Status"=enum."Cycle Not Started", "Command:Data"="", "Com Port"=0, "Time(S)"=0.0, "Err Count"=0}, {"Color"=0, "Last Read Status"=enum."Cycle Not Started", "Command:Data"="", "Com Port"=0, "Time(S)"=0.0, "Err Count"=0}, {"Color"=0, "Last Read Status"=enum."Cycle Not Started", "Command:Data"="", "Com Port"=0, "Time(S)"=0.0, "Err Count"=0}, {"Color"=0, "Last Read Status"=enum."Cycle Not Started", "Command:Data"="", "Com Port"=0, "Time(S)"=0.0, "Err Count"=0}]
  out "WriteOK":bool
  in  "Enter Button":bool
  out "Station Labels":string[](array[string])
  in  "Manual Station Pause":dbl=30.0
  in  "Emergency Valve Timer":dbl=300.0
  in  "Aisle 4 (45-56)":dbl[](array[numeric])=[64.6, 64.6, 64.6, 64.6, 64.6, 64.6, 64.6, 64.6, 64.6, 64.6, 64.6, 64.6]
  in  "Aisle 3 (33-44)":dbl[](array[numeric])=[64.6, 64.6, 64.6, 64.6, 64.6, 64.6, 64.6, 64.6, 64.6, 64.6, 64.6, 64.6]
  in  "Aisle 2 (21-32)":dbl[](array[numeric])=[64.6, 64.6, 64.6, 64.6, 64.6, 64.6, 64.6, 64.6, 64.6, 64.6, 64.6, 64.6]
  in  "Aisle 1 (1-20)":dbl[](array[numeric])=[64.6, 64.6, 64.6, 64.6, 64.6, 64.6, 64.6, 64.6, 64.6, 64.6, 64.6, 64.6, 64.6, 64.6, 64.6, 64.6, 64.6, 64.6, 64.6, 64.6]
  in  "Dryer To Save":T1 {"Night Cycle Count" format="%04d"; "Dryer Details"."Stop Dryer" items=["NO", "YES"]; "Dryer Details"."24 Hour Water Injection" items=["NO", "YES"]; "Dryer Details"."Run w/o Newfi" items=["NO", "YES"]; "Day Cycle Count" format="%04d"}
  out "Log Coms Array":string[](array[string])
  out "Data Sample Directory":path=path "D:/data/Wilt Sample Data"
  out "Dryer Bank Filename":path=path "D:/data/Wilt Backup"
  out "Data Sample Filename":path=path "D:/data/Wilt Sample Data"
  in  "Agilent Channel Assignment":path=path "C:/data/Agilent Channel Assignment - Wilt.ini"
  out "FileVersionInfo Out":T7
  in  "Com Config File":path=path "c:/work/ComArray.ini"
  in  "Water Times Filepath":path=path "c:/Work/watertimes.csv"
  in  "Robocopy Location":string="C:\\Program Files\\GE\\WILT\\Robocopy_Update.bat"
  in  "Daily Summary":string="C:\\Program Files\\GE\\WILT\\WILT_Daily_Summary - No Excel_LocalMachine.bat"
  out "Current Agilent Data":dbl[](array[numeric])
  out "Agilent Station Data Index Array":i32[][](array[numeric])
  out "Agilent Read Channels Array":T3[](array[typedef])
  out "Agilent Station Data Headers":string[][](array[string])
  out "All Agilent Refs":refnum<visa-resource-name>[](array[refnum])=["AGILENT1", "AGILENT2", "AGILENT3", "AGILENT4", "AGILENT5"]
  out "Agilent Read Refs":refnum<visa-resource-name>[](array[refnum])=["AGILENT1", "AGILENT2", "AGILENT3", "AGILENT4", "AGILENT5"]
  out "Agilent Channels Water Valves":T3[](array[typedef])
  out "Start Buttons":T3[](array[typedef])
  out "Temperature Channels":T3[](array[typedef])
  out "Test State array":string[](array[string])
  in  "Debug":bool
  out "Test State 7":T8=enum."Paused"
  out "Test State 6":T8=enum."Cooldown"
  out "Test State 5":T8=enum."Drying"
  out "Test State 4":T8=enum."Watering"
  out "Test State 3":T8=enum."Wait to Start"
  out "Test State 2":T8=enum."Wait Com"
  out "Test State":T8
  out "Init Complete":bool=TRUE
  out "Gathering Data Latch":bool=TRUE
  out "GUI Update":bool=TRUE
  out "Read Data Count":dbl
  out "exe?":bool
  out "InCorrect Cycle":bool
  out "Current State":string
  out "GUI":string
  out "Daq":string
  out "Main Loop Count":dbl
  out "UI Events":i32
  out "Samples":dbl
  out "DAQ Error List":string
  out "Control Error List":string
  out "UI Error List":string
  out "Agilent\nRead Errors":errorcluster
  out "UI error out":errorcluster
  out "DAQ error out":errorcluster
  out "Serial Error Array":errorcluster[](array[cluster])
  out "valve error out":errorcluster
  out "Error Stop All":errorcluster
  out "Agilent":T9
  in  "Station Timer":dbl[](array[numeric])
  in  "Saved Test State":T8[](array[typedef])
  in  "Station Test State":T8[](array[typedef])
  out "Emergency Timer.":i32[](array[numeric])
  out "Valve States":string[](array[string])
  in  "Save Setup":bool
  in  "Reset E-Timer":bool
  out "Temperature Fault":u32(colorbox)=15698688
  out "No Com":u32(colorbox)
  out "Running":u32(colorbox)=6618880
  out "Stopped":u32(colorbox)=16776960
  out "Fault":u32(colorbox)=16711680
  in  "Stop Test":bool
  in  "GUI Aisle 4":T1[](array[typedef]) {"Night Cycle Count" format="%04d"; "Dryer Details"."Stop Dryer" items=["NO", "YES"]; "Dryer Details"."24 Hour Water Injection" items=["NO", "YES"]; "Dryer Details"."Run w/o Newfi" items=["NO", "YES"]; "Day Cycle Count" format="%04d"}
  in  "GUI Aisle 3":T1[](array[typedef]) {"Night Cycle Count" format="%04d"; "Dryer Details"."Stop Dryer" items=["NO", "YES"]; "Dryer Details"."24 Hour Water Injection" items=["NO", "YES"]; "Dryer Details"."Run w/o Newfi" items=["NO", "YES"]; "Day Cycle Count" format="%04d"}
  in  "GUI Aisle 2":T1[](array[typedef]) {"Night Cycle Count" format="%04d"; "Dryer Details"."Stop Dryer" items=["NO", "YES"]; "Dryer Details"."24 Hour Water Injection" items=["NO", "YES"]; "Dryer Details"."Run w/o Newfi" items=["NO", "YES"]; "Day Cycle Count" format="%04d"}
  in  "GUI Aisle 1":T1[](array[typedef]) {"Night Cycle Count" format="%04d"; "Dryer Details"."Stop Dryer" items=["NO", "YES"]; "Dryer Details"."24 Hour Water Injection" items=["NO", "YES"]; "Dryer Details"."Run w/o Newfi" items=["NO", "YES"]; "Day Cycle Count" format="%04d"}
  in  "GUI Aisle 1A":T1[](array[typedef]) {"Night Cycle Count" format="%04d"; "Dryer Details"."Stop Dryer" items=["NO", "YES"]; "Dryer Details"."24 Hour Water Injection" items=["NO", "YES"]; "Dryer Details"."Run w/o Newfi" items=["NO", "YES"]; "Day Cycle Count" format="%04d"}
  in  "Robocopy":bool
  out "File Version Info":string
  out "User Notice":string
  in  "Reset Faults":bool
  out "Paused":u32(colorbox)=16860
  out "Unused":u32(colorbox)=7171459
  in  "Transition":bool
  in  "Resend Start":bool
  out "Day":bool
  out "Night":bool
  in  "Stop All":bool
  out "4":T9
  out "3":T9
  out "2":T9
  out "1A":T9
  out "1":T9
  # "WILT"
  # "D"
  # "N"
  # "D"
  # "N"
  # "Valve on Times"
  # "D"
  # "N"
  # "Action: Waits for user to enter serial number for dryer.\nTransition: SN and Model Num <> \"\""
  # "Action: Send Wilt Startup Commands every Wait Com Timer period. \nTransition: Must receive 0x74 command, and have a status of 0x00 thru 0x04."
  # "Transition: If Status = running 0x74,01, then Watering, else if\n elapsed time > Resend start limit, Waitcom."
  # "Action: Turn on Valve, wait for On Valve Times, Turn off Valve\nTrans: Go to Drying"
  # "Transitions: \nStatus = New dryer or Err, Waitcom\nStatus = Cycle Completed, Cooldown"
  # "Action: \nElapsed time = cool down time, Send Continue command\nTransition: Goto wait to start."
  # "Action: \nIf the status ever = Paused, go to this state.  The current station timer is set to \nthe current time.  \nTransition: When the status changes to something else, the test state is restored."
  # "D"
  # "N"
  # "D"
  # "N"
  # "D"
  # "N"
  # "D"
  # "N"
  # "D"
  # "N"
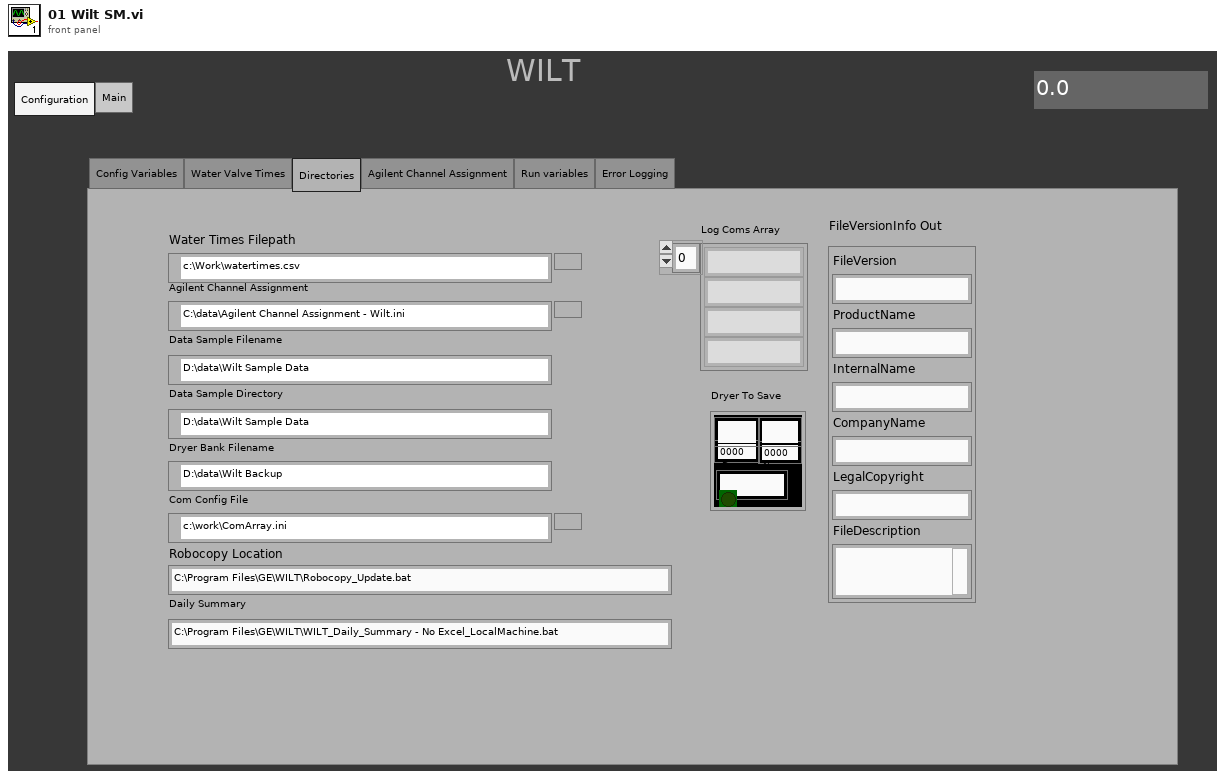
[diagram p1: front panel]
types:
  T1 = typedef "Dryer.ctl" = cluster{"Lab ID":string, "Day Cycle Count":i32, "Station Label":string, "Dryer Details":T2, "Sample Record ":string[], "Hist Record ":string[][], "Status Color":u32, "Boolean":bool, "Com Port":u8, "Bad Com Count":i32, "Current Run Start Time":dbl, "Night Cycle Count":i32, "Station Index":i32, "Cycle Index":string, "Audit Alert":bool}
  T2 = typedef "Dryer Details.ctl" = cluster{"Station":string, "Cycle Count Day":string, "Status":string, "Debug ASCII":string, "Notes":string, "Lab ID":string, "Total Time On":string, "TR Number":string, "Cycle Count Night":string, "Time On Day":string, "Time On Night":string, "Run w/o Newfi":i32, "24 Hour Water Injection":i32, "Stop Dryer":i32}
  T3 = typedef "Agilent Channel Definition.ctl" = cluster{"Channel":string, "Station":string, "Label":string, "Agilent Station":string}
  T4 = enum32{"Config Variables", "Water Valve Times", "Directories", "Agilent Channel Assignment", "Run variables", "Error Logging"}
  T5 = typedef "Dryer Com Port Info.ctl" = cluster{"Color":u32, "Last Read Status":T6, "Command:Data":string, "Com Port":u8, "Time(S)":dbl, "Err Count":u32}
  T6 = typedef "Dryer Status Ctrl.ctl" = enum16{"Cycle Not Started", "Cycle Running", "Paused", "Cycle Completed", "Eval Mode Entered", "Err", "Pause (No GEA2)"}
  T7 = typedef "FileVersionInformation.ctl" = cluster{"FileVersion":string, "ProductName":string, "InternalName":string, "CompanyName":string, "LegalCopyright":string, "FileDescription":string}
  T8 = typedef "Dryer Test State.ctl" = enum16{"No SN", "Wait Com", "Wait to Start", "Watering", "Drying", "Cooldown", "Paused", "Temp Fault", "Com Fault", "Pause Manual Station"}
  T9 = typedef "Semaphore RefNum" = refnum<k1>
  T10 = enum32{"invalid app kind", "Development System", "Run Time System", "Student Edition", "Embedded LabVIEW", "Evaluation", "Custom"}
  T11 = enum16{"Write History", "Write Sample Data", "Write Dryer Bank", "Read Dryer Bank", "Read Sample History"}
  T12 = cluster{"Data Sample Filename":path, "Data Sample Directory":path, "Agilent Read Refs":refnum<visa-resource-name>[], "All Confgured Com Array":u8[], "Elapsed Time (sec)":dbl, "GUI Aisle 1":T1[], "GUI Aisle 1A":T1[], "GUI Aisle 2":T1[], "GUI Aisle 3":T1[], "GUI Aisle 4":T1[], "Last Save Hour":string, "Save Bool":bool, "Agilent Data":dbl[], "Remote Station":bool, "Dryer Com Info":T5[]}
  T13 = cluster{"Current VI Reference":refnum<vi>, "Close Panel on Exit?":bool}
  T14 = typedef "GEA2 Dryer Interface Ctrl.ctl" = enum16{"Init Com Port", "SendCMD", "ReadPort", "Close Port", "Simulate Diag Data", "Simulate Dryer", "Send WILT Startup CMDs", "Send Continue CMD", "Read Continuous"}
  T15 = enum32{"Invalid", "Standard", "Closed", "Hidden", "Minimized", "Maximized"}
  T16 = cluster{"Water Times Filepath":path, "Core":cluster{"Current VI Reference":refnum<vi>, "Close Panel on Exit?":bool}, "Agilent Refs":refnum<visa-resource-name>[], "GUI Aisle 4":T1[], "GUI Aisle 3":T1[], "GUI Aisle 2":T1[], "GUI Aisle 1A":T1[], "GUI Aisle 1":T1[], "Station Timer":dbl[], "Station Test State":T8[], "Saved Test State":T8[], "Dryer Bank Filename":path, "Station Com List":u8[], "Start Buttons.":T3[], "Agilent Channels Water Valves.":T3[], "Pause Timer":i32[], "Remote Station":bool, "All Confgured Com Array":u8[], "All Test Stations Control":T1[], "USB6008":tag, "Emergency Timer":i32[]}
  T17 = typedef "Update Wilt GUI Control.ctl" = enum16{"Init Station Number", "Update Detail Data", "Update Status", "Init Com Port Num", "Update Sample Info", "Reset All Cycles"}
  T18 = enum16{"Left Button", "Center Button", "Right Button", "Window Close"}
  T19 = typedef "Dryer Commands.ctl" = u8
  T20 = cluster{"GUI Aisle 1":T1[], "GUI Aisle 1A":T1[], "GUI Aisle 2":T1[], "GUI Aisle 3":T1[], "GUI Aisle 4":T1[], "Dryer To Save":T1}
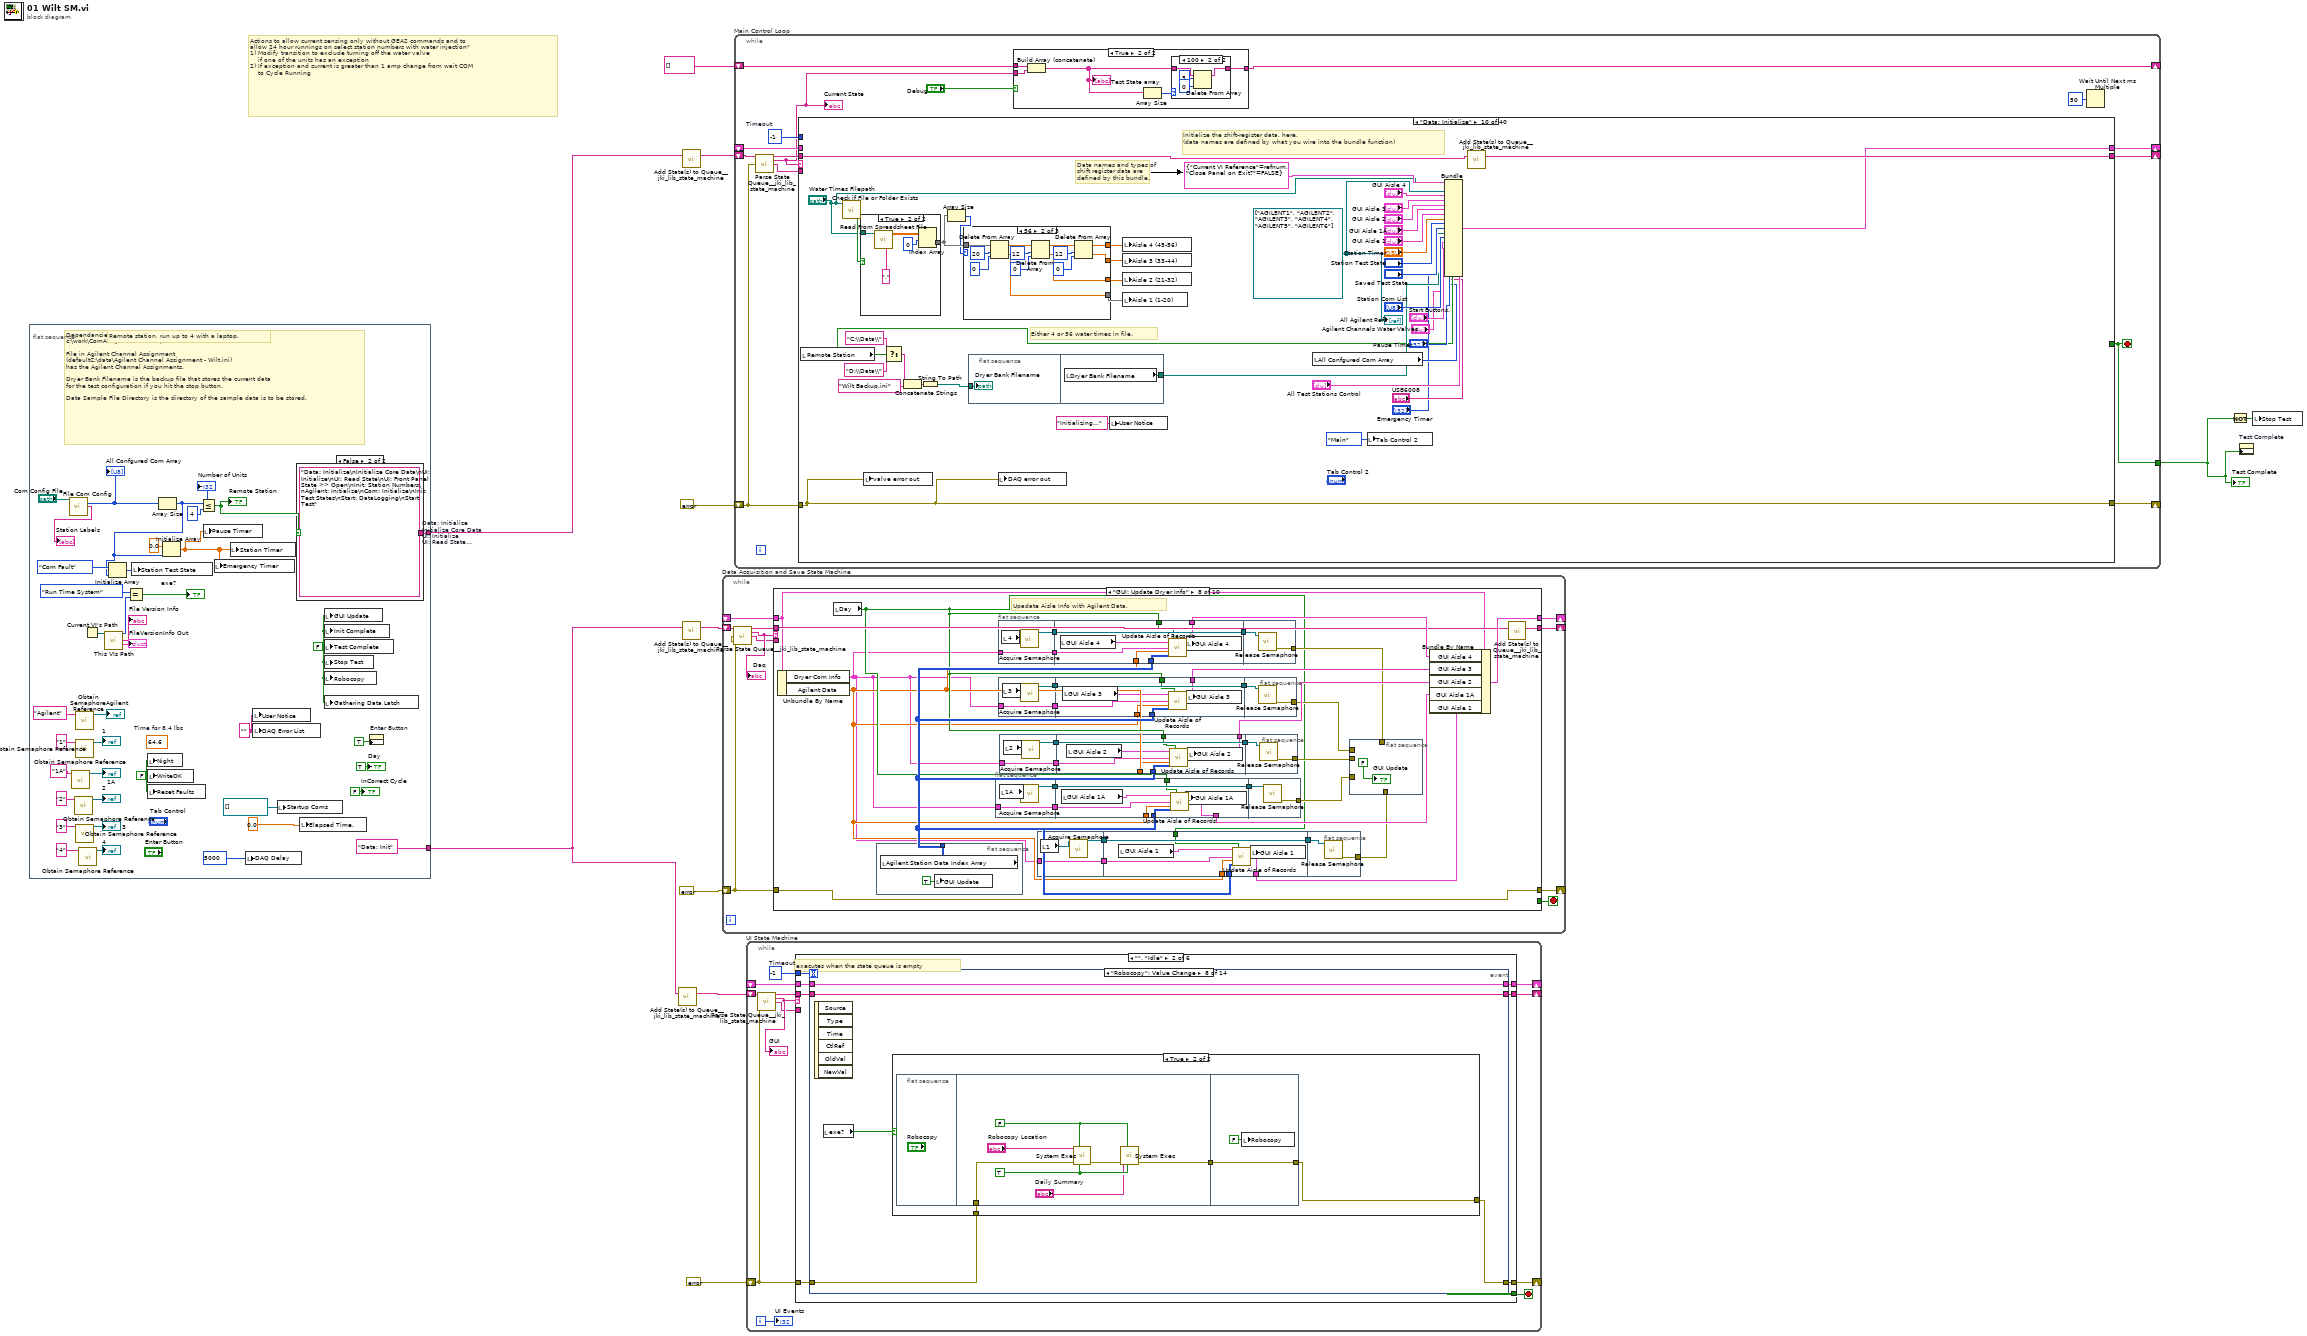
[diagram p0: block diagram]
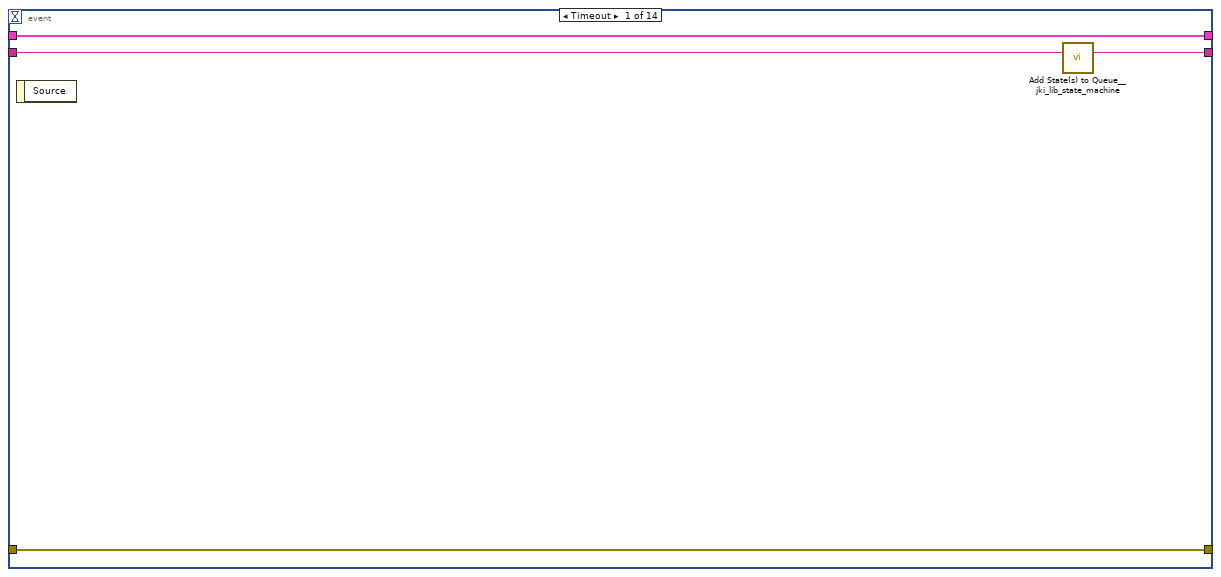
[diagram p3: hidden frame]
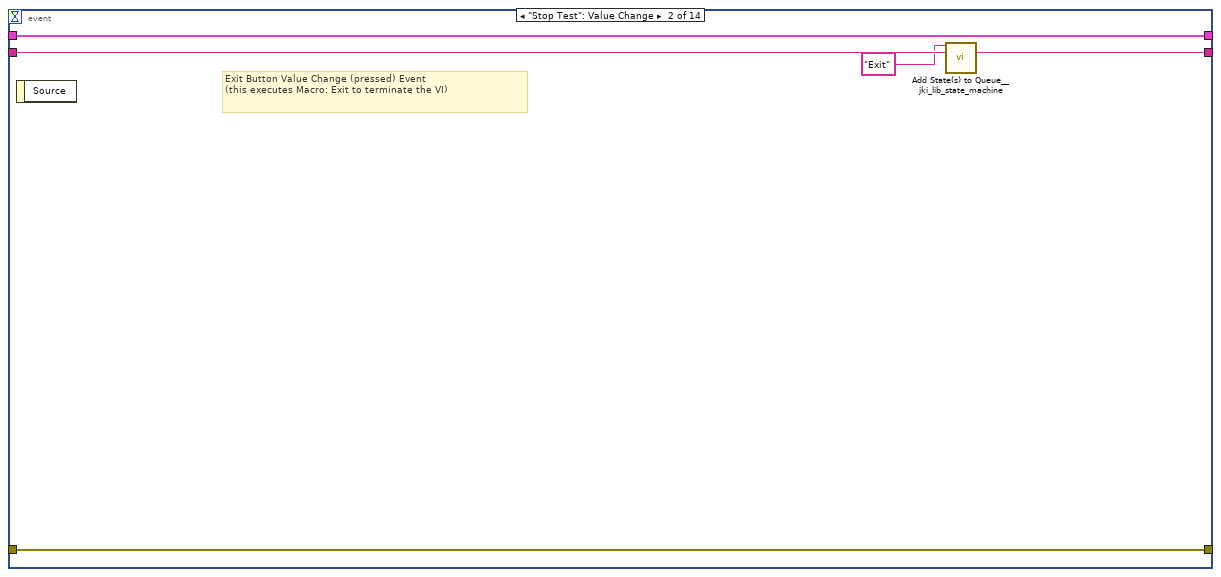
[diagram p4: hidden frame]
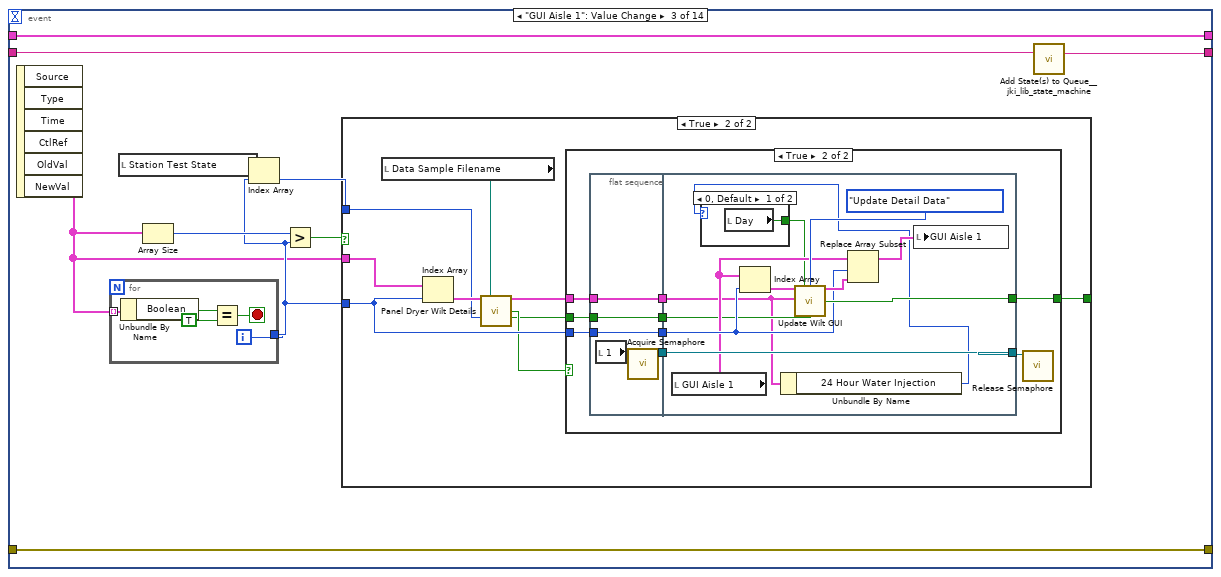
[diagram p5: hidden frame]
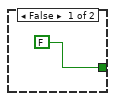
[diagram p6: hidden frame]
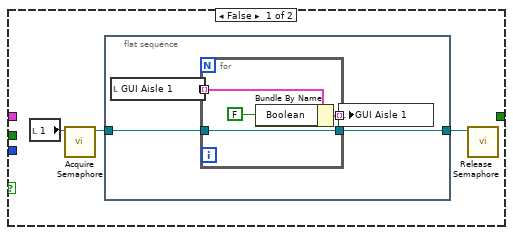
[diagram p7: hidden frame]
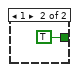
[diagram p8: hidden frame]
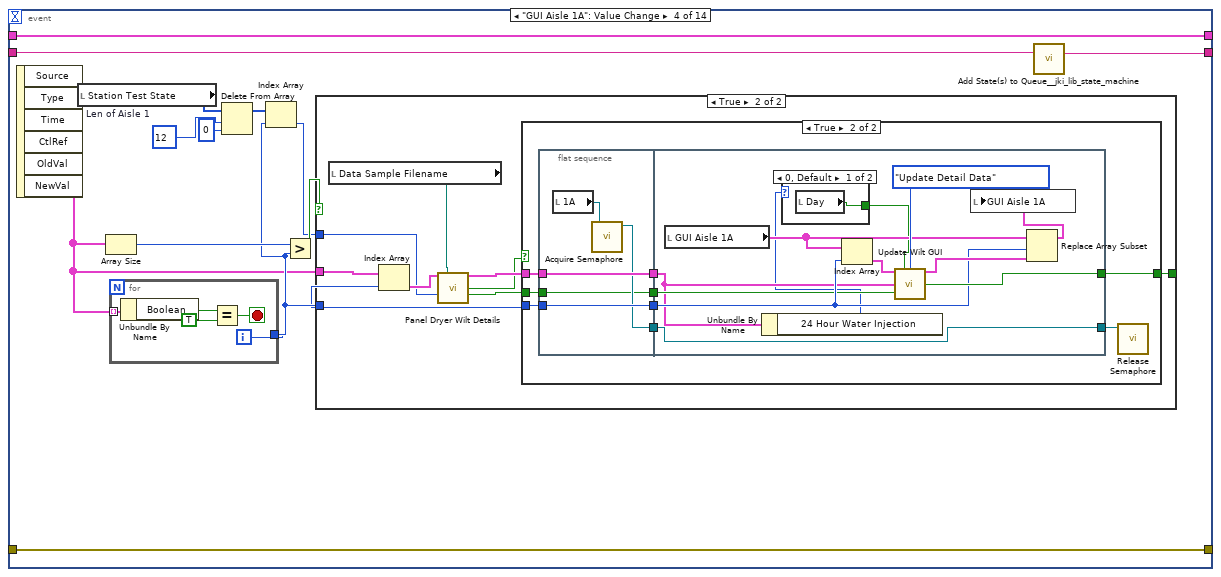
[diagram p9: hidden frame]
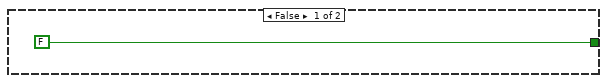
[diagram p10: hidden frame]
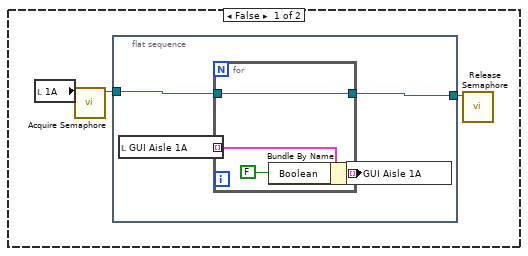
[diagram p11: hidden frame]
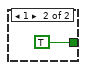
[diagram p12: hidden frame]
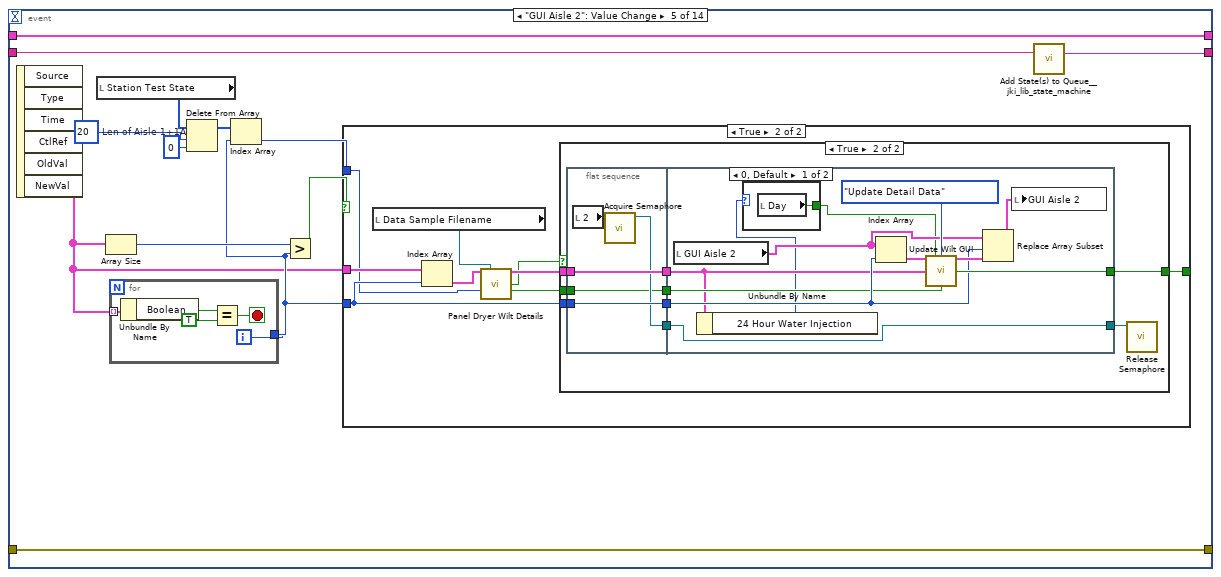
[diagram p13: hidden frame]
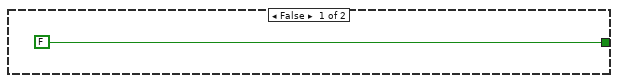
[diagram p14: hidden frame]
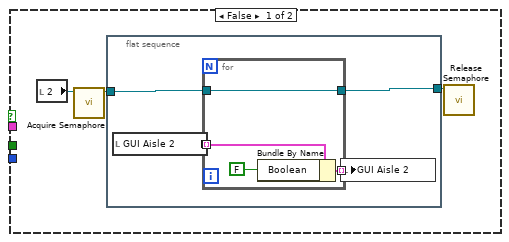
[diagram p15: hidden frame]
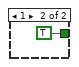
[diagram p16: hidden frame]
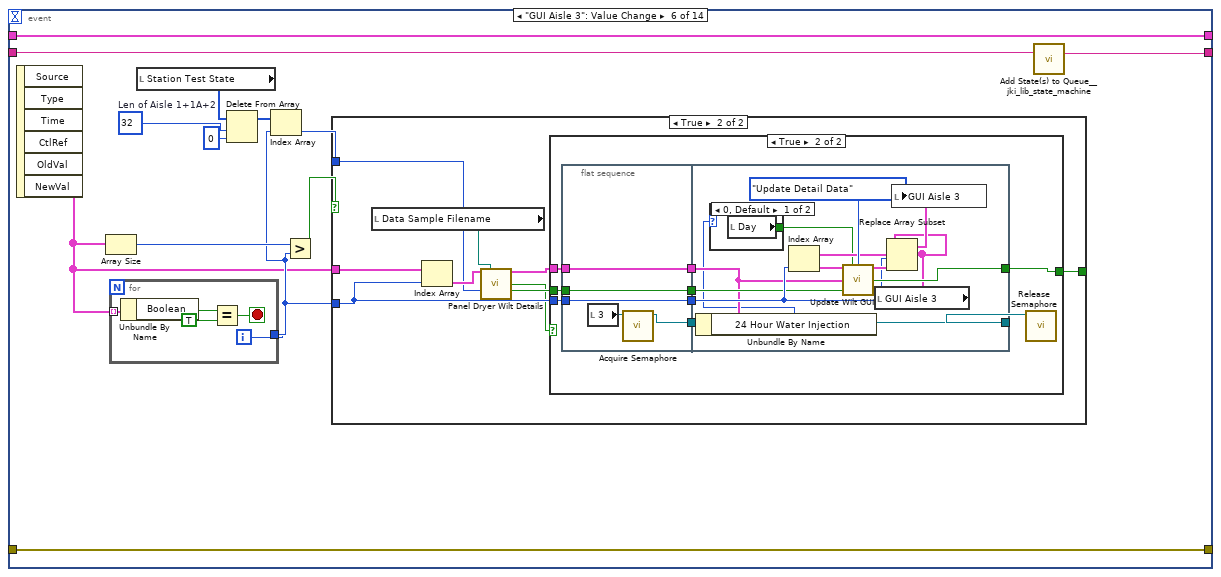
[diagram p17: hidden frame]
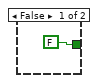
[diagram p18: hidden frame]
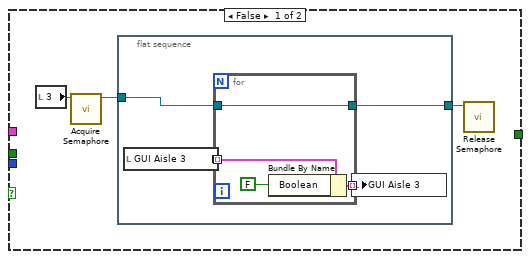
[diagram p19: hidden frame]
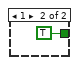
[diagram p20: hidden frame]
diagram:
  # "Actions to allow current sensing only without GEA2 commands and to\nallow 24 hour runnings on select station numbers with water injection\"\n1) Modify transition to exclude turning off the water valve\n    if one of the units has an exception\n2) If exception and current is greater than 1 amp change from wait COM\n    to Cycle Running"
  n1 = flat-sequence {
    tunnel: [w48] -> w10
    tunnel: ["Data: Init"] -> w5
    frame #0 {
      (unwired) 64.6  # Time for 8.4 lbs
      w21 = FALSE ("Reset Faults")
      w28 = "" ("User Notice")
      w17 = FALSE ("Init Complete")
      # "Remote station, run up to 4 with a laptop."
      # "Dependancies:\nc:\\work\\ComArray.ini lists com ports to be used.\n\nFile in Agilent Channel Assignment \n(defaultC:\\data\\Agilent Channel Assignment - Wilt.ini)\nhas the Agilent Channel Assignments.\n\nDryer Bank Filename is the backup file that stores the current data \nfor the test configuration if you hit the stop button. \n\nData Sample File Directory is the directory of the sample data is to be stored."
      n2 = call "File Com Config.vi"("file path (dialog if empty)"="Com Config File") -> ("Com Array Out"=w27:u8[], "Station Labels"=→"Station Labels":string[])  [unwired: 13 in]
      "All Confgured Com Array" <- w27
      n3 = call <vilib>:"Obtain Semaphore Reference.vi"("name (unnamed)"="1A") -> ("semaphore"=→"1A":T9)  [unwired: 4 in, 2 out]
      n4 = call <vilib>:"Obtain Semaphore Reference.vi"("name (unnamed)"="2") -> ("semaphore"=→"2":T9)  [unwired: 4 in, 2 out]
      n5 = call <vilib>:"Obtain Semaphore Reference.vi"("name (unnamed)"="Agilent") -> ("semaphore"=→"Agilent":T9)  [unwired: 4 in, 2 out]
      n6 = call <vilib>:"Obtain Semaphore Reference.vi"("name (unnamed)"="1") -> ("semaphore"=→"1":T9)  [unwired: 4 in, 2 out]
      n7 = call <vilib>:"Obtain Semaphore Reference.vi"("name (unnamed)"="3") -> ("semaphore"=→"3":T9)  [unwired: 4 in, 2 out]
      n8 = call <vilib>:"Obtain Semaphore Reference.vi"("name (unnamed)"="4") -> ("semaphore"=→"4":T9)  [unwired: 4 in, 2 out]
      n9 = Current VI's Path() -> (path=w31:path)
      n10 = call "This VIs Path.vi"("path"=w31) -> ("Application:Kind"=w20:T10, "File Version Info"=→"File Version Info":string, "FileVersionInfo Out"=→"FileVersionInfo Out":T7)  [unwired: 10 in, 2 out]
      n11 = Equal?(x=T10."Run Time System" ("Application:Kind"), y=w20) -> (x = y?=→"exe?":bool)
      n12 = local write "Night"(w21) -> ()
      n13 = local write "WriteOK"(w21) -> ()
      n14 = local write "Reset Faults"(w21) -> ()
      n15 = Array Size(array=w27) -> (size(s)=w13:i32)
      "Number of Units" <- w13
      n16 = Initialize Array(Dryer_Test_State."Com Fault" ("Test State"), w13) -> (w34:T8[])
      n17 = local write "Station Test State"(w34) -> ()
      n18 = Initialize Array(0.0 ("element"), w13) -> (w12:dbl[])
      n19 = Less Or Equal?(x=w13, y=4) -> (x <= y?=w25:bool)
      "Remote Station" <- w25
      n20 = local write "Pause Timer"(w12) -> ()
      n21 = local write "Emergency Timer"(w12) -> ()
      n22 = local write "Station Timer"(w12) -> ()
      n23 = local write "DAQ Delay"(u32 5000 ("DAQ Delay")) -> ()
      n24 = local write "User Notice"(w28) -> ()
      n25 = local write "DAQ Error List"(w28) -> ()
      n26 = local write "Startup Coms"(refnum<visa-resource-name>[] [] ("Startup Coms")) -> ()
      n27 = case shown="False" w25 {
        tunnel: [w51 w52] -> w48
        frame True {
          w51 = "Data: Initialize\nInitialize Core Data\nUI: Initialize\nUI: Read State\nUI: Front Panel State >> Open\nInit: Station Numbers\nCom: Initialize\nInit: Test States\nStart: DataLogging\nStart Test"  # Data: Initialize Initialize Core Data UI: Initialize UI: Read State UI: Front Panel State >> Open Init: Station Numbers Com: Initialize Init: Test States Start: DataLogging Start Test
        }
        frame False {
          w52 = "Data: Initialize\nInitialize Core Data\nUI: Initialize\nUI: Read State\nUI: Front Panel State >> Open\nInit: Station Numbers\nAgilent: Initialize\nCom: Initialize\nInit: Test States\nStart: DataLogging\nStart Test"  # Data: Initialize Initialize Core Data UI: Initialize UI: Read State UI: Front Panel State >> Open Init: Station Numbers Agilent: Initialize Com: Initialize Init: Test States Start: DataLogging Start Test
        }
      }
      n28 = local write "Elapsed Time."(0.0 ("Elapsed Time (sec)")) -> ()
      n29 = local write "GUI Update"(w17) -> ()
      n30 = local write "Init Complete"(w17) -> ()
      n31 = local write "Test Complete"(w17) -> ()
      n32 = local write "Stop Test"(w17) -> ()
      n33 = local write "Robocopy"(w17) -> ()
      n34 = local write "Gathering Data Latch"(w17) -> ()
      n35 = property on="Enter Button" class="Bool (strict)"("Key Focus"=TRUE) -> ()  [unwired: 2 in, 2 out]
      "Day" <- TRUE ("Day")
      "InCorrect Cycle" <- FALSE ("InCorrect Cycle")
    }
  }
  n36 = call <vilib>:"Add State(s) to Queue__jki_lib_state_machine.vi"("State(s) in (\"\")"=w5) -> ("States Out"=w8:string)  [unwired: 14 in]
  n37 = call <vilib>:"Add State(s) to Queue__jki_lib_state_machine.vi"("State(s) in (\"\")"=w10) -> ("States Out"=w11:string)  [unwired: 14 in]
  n38 = call <vilib>:"Add State(s) to Queue__jki_lib_state_machine.vi"("State(s) in (\"\")"=w5) -> ("States Out"=w9:string)  [unwired: 14 in]
  n39 = while "Data Acquisition and Save State Machine" {
    shift-right: [w55] -> _
    shift-left: _ -> [w54]
    shift-right: [w58] -> _
    shift-left: errorcluster {"status"=FALSE, "code"=0, "source"=""} ("error out") -> [w53]
    shift-right: [w57] -> _
    shift-left: w9 -> [w59]
    stop <- w56 stop-if-true
    n40 = call <vilib>:"Parse State Queue__jki_lib_state_machine.vi"("State Queue"=w59, "Error In (no error)"=w53) -> ("Remaining States"=w61:string, "Current State"=w62:string, "Arguments"=w60:string)  [unwired: 11 in]
    "Daq" <- w62
    n41 = case shown="\"GUI: Update Dryer Info\"" w62 {
      selector: w62 -> [_ w84 _ _ _ _ _ _ _ _]
      tunnel: w61 -> [w73 w88 w110 w116 w120 w160 w228 w250 w362 w367]
      tunnel: w60 -> [_ _ _ _ _ _ _ _ _ _]
      tunnel: w54 -> [w68 w86 w107 w114 w117 _ w224 w248 w351 w365]
      tunnel: [w71 w90 errorcluster {"status"=FALSE, "code"=0, "source"=""} ("error out") w113 w118 w158 w214 w251 w352 w363] -> w58
      tunnel: w53 -> [w70 w89 w104 w113 w118 w158 w225 w251 w353 w363]
      tunnel: [w72 w87 w109 w115 w119 w159 w227 w253 w361 w366] -> w57
      tunnel: [_ _ _ TRUE _ _ _ _ _ _] -> w56
      tunnel: [w69 w86 w107 w114 w117 w157 w223 w252 w350 w365] -> w55
      frame "", "Idle" {
        n42 = local read "DAQ Delay"() -> (w65:u32)
        n43 = Unbundle By Name(w68) -> ("Elapsed Time (sec)"=w67:dbl)
        n44 = To Long Integer(number=w65) -> (32bit integer=w63:i32)
        n45 = call "E-Time.vi"() -> ("Elapsed Time (sec)"=w66:dbl)  [unwired: 9 in, 2 out]
        n46 = call "Timeout Calc.vi"("Complete time"=w66, "Gather Data Period"=w63, "Start Time"=w67) -> ("Delay Time"=w64:i32)  [unwired: 8 in]
        n47 = event shown="[0] Timeout" {
          selector: _ -> [_ _]
          dyn-events: _ -> [_ _]
          timeout: w64 -> [_ _]
          tunnel: w73 -> [w78 w83]
          tunnel: [w77 w82] -> w72
          tunnel: w68 -> [w75 w80]
          tunnel: [w76 w81] -> w71
          tunnel: w70 -> [w76 w81]
          tunnel: [w75 w80] -> w69
          event Timeout {
            n48 = event-data() -> ()  [unwired: 1 in, 1 out]
            n49 = call <vilib>:"Add State(s) to Queue__jki_lib_state_machine.vi"("State(s) in (\"\")"=w78, "State(s) at Back (\"\")"="Read Data\nGUI: Update Dryer Info\nSave Data Sample\nSave Data History") -> ("States Out"=w77:string)  [unwired: 13 in]
          }
          event "Stop Test": Value Change {
            # "Exit Button Value Change (pressed) Event\n(this executes Macro: Exit to terminate the VI)"
            n50 = event-data() -> ()  [unwired: 1 in, 6 out]
            n51 = call <vilib>:"Add State(s) to Queue__jki_lib_state_machine.vi"("State(s) in Front (\"\")"="Exit", "State(s) in (\"\")"=w83) -> ("States Out"=w82:string)  [unwired: 13 in]
          }
        }
      }
      frame Default {
        w93 = 42 items=["No error", "Argument error", "Memory is full", "Out of zone", "End of file", "File already open", "Generic file I/O error", "File not found", "File permission error", "Disk is full", "Duplicate path", "Too many files open", "System feature not enabled", "Resource file not found", "Cannot add resource", "Resource not found", "Image not found", "Image memory error", "Pen does not exist", "Config type invalid", "Config token not found", "Config parse error", "Config memory error", "Bad external code format", "Bad external code offset", "External code not present", "Null window", "Destroy window error", "Null menu", "Print aborted", "Bad print record", "Print driver error", "Windows error during printing", "Memory error during printing", "Print dialog error", "Generic print error", "Invalid device refnum", "Device not found", "Device parameter error", "Device unit error", "Cannot open device", "Device call aborted", "Generic error", "Cancelled by user", "Object ID too low", "Object ID too high", "Object not in heap", "Unknown heap", "Unknown object (invalid DefProc)", "Unknown object (DefProc not in table)", "Message out of range", "Invalid (null) method", "Unknown message", "Manager call not supported", "Bad address", "Network operation in progress", "Network operation timed out", "Connection is busy", "Network attribute not supported", "Network error", "Address in use", "System out of memory", "Connection aborted", "Connection refused", "Not connected", "Already connected", "Connection closed", "Initialization error (interapplication manager)", "Bad occurrence", "Wait on unbound occurrence handler", "Occurrence queue overflow", "Datalog type conflict", "Unused", "Unrecognized type (interapplication manager)", "Memory corrupt", "Failed to make temporary DLL", "Old CIN version", "Drag socket not found", "Failed to load drop-object", "Failed to register OLE object", "Failed to release OLE object", "Format specifier type mismatch", "Unknown format specifier", "Too few format specifiers", "Too many format specifiers", "Scan failed", "Newer CIN version", "Error converting to variant", "Runtime menu error", "Password tampered", "Variant attribute not found", "Incompatible variant data type", "Event data is not available", "Event Store is not present", "Occurrence is not found", "Event Queue is not created", "Event info is not available", "Refnum passed is NULL", "Error retrieving Class GUID", "Error retrieving CoClass GUID", "Error retrieving TypeLib GUID.", "Bad built application magic bytes.", "Specific driver is different from the specific driver associated with the Logical Name.", "There is no session opened to the class driver.", "Max Error", "MAX - Error with config objects", "MAX - Error loading configuration", "MAX - Group not supported"]
        # "Current State"
        # "Do not delete, rename, or modify this frame.\n(this is used to capture unhandled states and typos)"
        # "Handle mistyped state name (developer tool)"
        n52 = Format Into String(format string="Software Exception: Unhandled State \"%s\"." ("message"), error in=w89, w84) -> (resulting string=w92:string, error out=w91:errorcluster)  [unwired: 1 in]
        n53 = call <vilib>:"Error Cluster From Error Code.vi"("show call chain? (False)"=TRUE, "error in (no error)"=w91, "error message (\"\")"=w92, "error code (0)"=w93) -> ("error out"=w90:errorcluster)  [unwired: 5 in]
        n54 = call <vilib>:"Add State(s) to Queue__jki_lib_state_machine.vi"("State(s) in (\"\")"=w88) -> ("States Out"=w87:string)  [unwired: 14 in]
      }
      frame "Error Handler" {
        # "Handle any errors here.\nYou can also output any states to clean-up after errors occur"
        # "Clear error"
        n55 = local read "Debug"() -> (w98:bool)
        n56 = case shown="False" w98 {
          tunnel: w104 -> [_ w111]
          frame False {
          }
          frame True {
            # "Unhandled Error -- Display it"
            n57 = call <vilib>:"General Error Handler.vi"("error in (no error)"=w111) -> ()  [unwired: 10 in, 5 out]
          }
        }
        n58 = Unbundle By Name(w104) -> ("source"=w101:string)
        n59 = call "Counter.vi"() -> ("Count"=w97:dbl)  [unwired: 11 in]
        n60 = To Long Integer(number=w97) -> (32bit integer=w96:i32)
        n61 = local read "DAQ Error List"() -> (w99:string)
        n62 = Number To Decimal String(number=w96) -> (decimal integer string=w95:string)  [unwired: 1 in]
        n63 = Concatenate Strings(w95, " Error DAQ: " ("string"), w101) -> (w103:string)
        n64 = local write "User Notice"(w103) -> ()
        n65 = Concatenate Strings(w101, "\n", w99) -> (→"DAQ Error List":string)
        n66 = call <vilib>:"Add State(s) to Queue__jki_lib_state_machine.vi"("State(s) in Front (\"\")"="/* Post Error States", "State(s) in (\"\")"=w110) -> ("States Out"=w109:string)  [unwired: 13 in]
        "DAQ error out" <- w104
      }
      frame "Exit" {
        # "Do not put any code in this frame.\n(No errors that occur here will be handled.)"
        n67 = call <vilib>:"Add State(s) to Queue__jki_lib_state_machine.vi"("State(s) in (\"\")"=w116) -> ("States Out"=w115:string)  [unwired: 14 in]
      }
      frame "----------Data Acqisition ----------" {
        # "Template Separator\n(You can make a copy of, or modify, this frame)"
        n68 = call <vilib>:"Add State(s) to Queue__jki_lib_state_machine.vi"("State(s) in (\"\")"=w120) -> ("States Out"=w119:string)  [unwired: 14 in]
      }
      frame "Data: Init" {
        # "Data Log Time"
        # "Template Separator\n(You can make a copy of, or modify, this frame)"
        n69 = flat-sequence {
          tunnel: [w166] -> w152
          tunnel: [w163] -> w141
          tunnel: [w162] -> w125
          tunnel: w152 -> [w186]
          tunnel: w141 -> [w175]
          tunnel: [w185] -> w140
          tunnel: [w188] -> w139
          tunnel: [w187] -> w138
          tunnel: [w186] -> w137
          tunnel: [w183] -> w136
          tunnel: [w182] -> w135
          tunnel: [w181] -> w134
          tunnel: [w180] -> w133
          tunnel: [w179] -> w132
          tunnel: [w174] -> w131
          tunnel: [w184] -> w130
          tunnel: [w174] -> w129
          tunnel: [w178] -> w128
          tunnel: ["Agilent Data"] -> w127
          tunnel: w125 -> [w172]
          tunnel: [w172] -> w124
          tunnel: [w171] -> w122
          tunnel: [w194] -> w142
          tunnel: [w193] -> w143
          tunnel: [w195] -> w144
          tunnel: [w192] -> w145
          tunnel: [w196] -> w146
          tunnel: [w197] -> w147
          tunnel: [w198] -> w148
          tunnel: [w199] -> w149
          tunnel: [w200] -> w150
          tunnel: [w201] -> w153
          tunnel: [w202] -> w154
          tunnel: [w203] -> w155
          tunnel: [w204] -> w156
          tunnel: w140 -> [w204]
          tunnel: w139 -> [w203]
          tunnel: w138 -> [w202]
          tunnel: w137 -> [w201]
          tunnel: w136 -> [w200]
          tunnel: w135 -> [w199]
          tunnel: w134 -> [w198]
          tunnel: w133 -> [w197]
          tunnel: w132 -> [w196]
          tunnel: w131 -> [_]
          tunnel: w130 -> [w195]
          tunnel: w129 -> [_]
          tunnel: w128 -> [w194]
          tunnel: [w191] -> w126
          tunnel: w127 -> [w191]
          tunnel: w124 -> [w190]
          tunnel: [w190] -> w123
          tunnel: w122 -> [w189]
          tunnel: [w189] -> w121
          frame #0 {
            n70 = while {
              tunnel: [w167] -> w166
              stop <- w169 stop-if-true
              n71 = local read "DAQ Delay"() -> (w168:u32)
              n72 = local read "Test Complete"() -> (w167:bool)
              n73 = local read "Init Complete"() -> (w170:bool)
              n74 = Wait (ms)(milliseconds to wait=w168) -> ()  [unwired: 1 out]
              n75 = Or(x=w170, y=w167) -> (x .or. y?=w169:bool)
            }
            n76 = local read "Remote Station"() -> (w162:bool)
            n77 = Select(t="C:\\Data\\", s=w162, f="D:\\Data\\") -> (s? t:f=w163:string)
          }
          frame #1 {
            w178 = TRUE  # Save Bool
            w184 = "%H"  # Last Save Hour
            n78 = local read "Dryer Com Info"() -> (w171:T5[])
            n79 = local read "All Confgured Com Array"() -> (w188:u8[])
            n80 = Concatenate Strings(w175, "Wilt Sample Data") -> (w176:string)
            n81 = local read "Agilent Read Refs"() -> (w185:refnum<visa-resource-name>[])
            n82 = local read "GUI Aisle 2"() -> (w181:T1[])
            n83 = local read "GUI Aisle 3"() -> (w180:T1[])
            n84 = local read "GUI Aisle 1A"() -> (w182:T1[])
            n85 = local read "GUI Aisle 4"() -> (w179:T1[])
            n86 = local read "GUI Aisle 1"() -> (w183:T1[])
            n87 = String To Path(string=w176) -> (path=w174:path)
            "Data Sample Directory" <- w174
            "Data Sample Filename" <- w174
            n88 = call "E-Time.vi"() -> ("Elapsed Time (sec)"=w187:dbl)  [unwired: 9 in, 2 out]
          }
          frame #2 {
            n89 = local read "Data Sample Directory"() -> (w192:path)
            n90 = local read "Data Sample Filename"() -> (w193:path)
          }
        }
        n91 = case shown="False" w153 {
          tunnel: [_ "Exit" ("State(s) in Front (\"\")")] -> w151
          frame False {
          }
          frame True {
          }
        }
        n92 = Bundle("Data Sample Filename"=w143, "Data Sample Directory"=w145, "Agilent Read Refs"=w156, "All Confgured Com Array"=w155, "Elapsed Time (sec)"=w154, "GUI Aisle 1"=w150, "GUI Aisle 1A"=w149, "GUI Aisle 2"=w148, "GUI Aisle 3"=w147, "GUI Aisle 4"=w146, "Last Save Hour"=w144, "Save Bool"=w142, "Agilent Data"=w126, "Remote Station"=w123, "Dryer Com Info"=w121) -> (w157:T12)  [unwired: 1 in]
        n93 = call <vilib>:"Add State(s) to Queue__jki_lib_state_machine.vi"("State(s) in Front (\"\")"=w151, "State(s) in (\"\")"=w160) -> ("States Out"=w159:string)  [unwired: 13 in]
      }
      frame "Read Data" {
        # "Gathers all data:"
        n94 = Unbundle By Name(w224) -> ("Agilent Read Refs"=w226:refnum<visa-resource-name>[], "All Confgured Com Array"=w221:u8[], "Remote Station"=w208:bool, "Dryer Com Info"=w207:T5[])
        n95 = local read "Station Test State"() -> (w205:T8[])
        n96 = call "E-Time.vi"("error in (no error)"=w225) -> ("error out"=w222:errorcluster, "Elapsed Time (sec)"=w210:dbl)  [unwired: 8 in, 1 out]
        "Elapsed Time." <- w210
        n97 = Not Equal?(x=w205, y=Dryer_Test_State."Com Fault" ("Test State")) -> (x != y?=w215:bool[])
        n98 = local read "All Test Stations"() -> (w213:T1[])
        n99 = local read "Agilent Read Channels Array"() -> (w211:T3[])
        n100 = call "Counter.vi"() -> ("Count"=→"Read Data Count":dbl)  [unwired: 11 in]
        n101 = case shown="False" w208 {
          tunnel: w226 -> [w236 _]
          tunnel: w222 -> [w235 _]
          tunnel: [w230 errorcluster {"status"=FALSE, "code"=0, "source"=""} ("error out")] -> w212
          tunnel: [w229 dbl[] []] -> w209
          frame False {
            # "SW set >1e6 values to 1000."
            n102 = local read "Agilent"() -> (w233:T9)
            n103 = call "Agilent Read 5 Units.vi"("Agilent Refs"=w236, "error in (no error)"=w235, "Agilent"=w233) -> ("All Agilent Data"=w234:dbl[], "error out"=w230:errorcluster)  [unwired: 15 in]
            n104 = for {
              tunnel: w234 -> [w240] mode=indexing
              tunnel: [w239] -> w229 mode=indexing
              tunnel: 1000.0 ("t") -> [w238]
              tunnel: 1000000.0 ("y") -> [w237]
              n105 = Greater?(x=w240, y=w237) -> (0:w241:bool)
              n106 = Select(t=w238, s=w241, f=w240) -> (s? t:f=w239:dbl)
            }
          }
          frame True {
          }
        }
        "Current Agilent Data" <- w209
        "Agilent\nRead Errors" <- w212
        n107 = To Unsigned Byte Integer(number=w221) -> (unsigned 8bit integer=w219:u8[])
        n108 = call "Read All Dryer Com Ports.vi"("Com Array"=w219, "Agilent Read Channels Array"=w211, "Station Test State"=w205, "Status Array In"=w207, "Enable"=w215, "All Test Stations"=w213, "error in (no error)"=w212, "Current Agilent Data"=w209) -> ("Log Coms Array"=→"Log Coms Array":string[], "Status Array Out"=w206:T5[], "Serial Error Array"=→"Serial Error Array":errorcluster[], "error out"=w214:errorcluster)  [unwired: 4 in]
        "Dryer Com Info" <- w206
        n109 = Bundle By Name(cluster=w224, "Elapsed Time (sec)"=w210, "Agilent Data"=w209, "Dryer Com Info"=w206) -> (w223:T12)
        n110 = case shown="No Error" w214 {
          selector: w214 -> [_ w245]
          frame No Error {
            w244 = TRUE
            n111 = property on="Gathering Data Latch" class="Bool (strict)"("Val(Sgnl)"=w244) -> ()  [unwired: 2 in, 2 out]
            "Gathering Data Latch" <- w244
          }
          frame Error {
            n112 = local write "DAQ error out"(w245) -> ()
          }
        }
        n113 = call <vilib>:"Add State(s) to Queue__jki_lib_state_machine.vi"("State(s) in (\"\")"=w228) -> ("States Out"=w227:string)  [unwired: 14 in]
      }
      frame "GUI: Update Dryer Info" {
        # "Upadate Aisle Info with Agilent Data."
        n114 = Unbundle By Name(w248) -> ("Dryer Com Info"=w246:T5[], "Agilent Data"=w247:dbl[])
        n115 = local read "Day"() -> (w249:bool)
        n116 = flat-sequence {
          tunnel: [w341] -> w254
          frame #0 {
            n117 = local read "Agilent Station Data Index Array"() -> (w341:i32[][])
            n118 = local write "GUI Update"(TRUE ("GUI Updatge")) -> ()
          }
        }
        n119 = flat-sequence {
          tunnel: w246 -> [w295]
          tunnel: [w295] -> w270
          tunnel: [w293] -> w269
          tunnel: w247 -> [w302]
          tunnel: w254 -> [w301]
          tunnel: w270 -> [w300]
          tunnel: [w299] -> w268
          tunnel: w269 -> [w299]
          tunnel: [w298] -> w261
          tunnel: w249 -> [w297]
          tunnel: w268 -> [w304]
          tunnel: [w303] -> w258
          frame #0 {
            n120 = local read "1A"() -> (w294:T9)
            n121 = call <vilib>:"Acquire Semaphore.vi"("semaphore"=w294) -> ("semaphore out"=w293:T9)  [unwired: 4 in, 2 out]
          }
          frame #1 {
            n122 = local read "GUI Aisle 1A"() -> (w296:T1[])
            n123 = call "Update Aisle of Records.vi"("GUI Aisle In"=w296, "Day Shift?"=w297, "Dryer Com Info"=w300, "Current Agilent Data"=w302, "Agilent Station Data Index Array"=w301) -> ("Aisle Array Out"=w298:T1[])  [unwired: 10 in]
            n124 = local write "GUI Aisle 1A"(w298) -> ()
          }
          frame #2 {
            n125 = call <vilib>:"Release Semaphore.vi"("semaphore"=w304) -> ("error out"=w303:errorcluster)  [unwired: 5 in, 1 out]
          }
        }
        n126 = flat-sequence {
          tunnel: w246 -> [w331]
          tunnel: [w331] -> w279
          tunnel: [w329] -> w278
          tunnel: w247 -> [w338]
          tunnel: w254 -> [w337]
          tunnel: w279 -> [w336]
          tunnel: [w335] -> w277
          tunnel: w278 -> [w335]
          tunnel: [w334] -> w264
          tunnel: w249 -> [w333]
          tunnel: w277 -> [w340]
          tunnel: [w339] -> w255
          frame #0 {
            n127 = local read "4"() -> (w330:T9)
            n128 = call <vilib>:"Acquire Semaphore.vi"("semaphore"=w330) -> ("semaphore out"=w329:T9)  [unwired: 4 in, 2 out]
          }
          frame #1 {
            n129 = local read "GUI Aisle 4"() -> (w332:T1[])
            n130 = call "Update Aisle of Records.vi"("GUI Aisle In"=w332, "Day Shift?"=w333, "Dryer Com Info"=w336, "Current Agilent Data"=w338, "Agilent Station Data Index Array"=w337) -> ("Aisle Array Out"=w334:T1[])  [unwired: 10 in]
            n131 = local write "GUI Aisle 4"(w334) -> ()
          }
          frame #2 {
            n132 = call <vilib>:"Release Semaphore.vi"("semaphore"=w340) -> ("error out"=w339:errorcluster)  [unwired: 5 in, 1 out]
          }
        }
        n133 = flat-sequence {
          tunnel: w246 -> [w319]
          tunnel: [w319] -> w276
          tunnel: [w317] -> w275
          tunnel: w247 -> [w326]
          tunnel: w254 -> [w325]
          tunnel: w276 -> [w324]
          tunnel: [w323] -> w274
          tunnel: w275 -> [w323]
          tunnel: [w322] -> w263
          tunnel: w249 -> [w321]
          tunnel: w274 -> [w328]
          tunnel: [w327] -> w256
          frame #0 {
            n134 = local read "3"() -> (w318:T9)
            n135 = call <vilib>:"Acquire Semaphore.vi"("semaphore"=w318) -> ("semaphore out"=w317:T9)  [unwired: 4 in, 2 out]
          }
          frame #1 {
            n136 = local read "GUI Aisle 3"() -> (w320:T1[])
            n137 = call "Update Aisle of Records.vi"("GUI Aisle In"=w320, "Day Shift?"=w321, "Dryer Com Info"=w324, "Current Agilent Data"=w326, "Agilent Station Data Index Array"=w325) -> ("Aisle Array Out"=w322:T1[])  [unwired: 10 in]
            n138 = local write "GUI Aisle 3"(w322) -> ()
          }
          frame #2 {
            n139 = call <vilib>:"Release Semaphore.vi"("semaphore"=w328) -> ("error out"=w327:errorcluster)  [unwired: 5 in, 1 out]
          }
        }
        n140 = flat-sequence {
          tunnel: w246 -> [w307]
          tunnel: [w307] -> w273
          tunnel: [w305] -> w272
          tunnel: w254 -> [w314]
          tunnel: w273 -> [w313]
          tunnel: [w312] -> w271
          tunnel: w272 -> [w312]
          tunnel: w247 -> [w311]
          tunnel: [w310] -> w262
          tunnel: w249 -> [w309]
          tunnel: w271 -> [w316]
          tunnel: [w315] -> w257
          frame #0 {
            n141 = local read "2"() -> (w306:T9)
            n142 = call <vilib>:"Acquire Semaphore.vi"("semaphore"=w306) -> ("semaphore out"=w305:T9)  [unwired: 4 in, 2 out]
          }
          frame #1 {
            n143 = local read "GUI Aisle 2"() -> (w308:T1[])
            n144 = call "Update Aisle of Records.vi"("GUI Aisle In"=w308, "Day Shift?"=w309, "Dryer Com Info"=w313, "Current Agilent Data"=w311, "Agilent Station Data Index Array"=w314) -> ("Aisle Array Out"=w310:T1[])  [unwired: 10 in]
            n145 = local write "GUI Aisle 2"(w310) -> ()
          }
          frame #2 {
            n146 = call <vilib>:"Release Semaphore.vi"("semaphore"=w316) -> ("error out"=w315:errorcluster)  [unwired: 5 in, 1 out]
          }
        }
        n147 = flat-sequence {
          tunnel: w246 -> [w283]
          tunnel: [w283] -> w267
          tunnel: [w281] -> w266
          tunnel: w247 -> [w290]
          tunnel: w254 -> [w289]
          tunnel: w267 -> [w288]
          tunnel: [w287] -> w265
          tunnel: w266 -> [w287]
          tunnel: [w286] -> w260
          tunnel: w249 -> [w285]
          tunnel: w265 -> [w292]
          tunnel: [w291] -> w259
          frame #0 {
            n148 = local read "1"() -> (w282:T9)
            n149 = call <vilib>:"Acquire Semaphore.vi"("semaphore"=w282) -> ("semaphore out"=w281:T9)  [unwired: 4 in, 2 out]
          }
          frame #1 {
            n150 = local read "GUI Aisle 1"() -> (w284:T1[])
            n151 = call "Update Aisle of Records.vi"("GUI Aisle In"=w284, "Day Shift?"=w285, "Dryer Com Info"=w288, "Current Agilent Data"=w290, "Agilent Station Data Index Array"=w289) -> ("Aisle Array Out"=w286:T1[])  [unwired: 10 in]
            n152 = local write "GUI Aisle 1"(w286) -> ()
          }
          frame #2 {
            n153 = call <vilib>:"Release Semaphore.vi"("semaphore"=w292) -> ("error out"=w291:errorcluster)  [unwired: 5 in, 1 out]
          }
        }
        n154 = flat-sequence {
          tunnel: w255 -> [_]
          tunnel: w256 -> [_]
          tunnel: w257 -> [_]
          tunnel: w258 -> [_]
          tunnel: w259 -> [_]
          frame #0 {
            "GUI Update" <- FALSE ("GUI Updatge")
          }
        }
        n155 = Bundle By Name(cluster=w248, "GUI Aisle 4"=w264, "GUI Aisle 3"=w263, "GUI Aisle 2"=w262, "GUI Aisle 1A"=w261, "GUI Aisle 1"=w260) -> (w252:T12)
        n156 = call <vilib>:"Add State(s) to Queue__jki_lib_state_machine.vi"("State(s) in (\"\")"=w250) -> ("States Out"=w253:string)  [unwired: 14 in]
      }
      frame "Save Data Sample" {
        # "FIXME: Data Sample FILENAME and FILEDIRECTORY confusion."
        # "Template Separator\n(You can make a copy of, or modify, this frame)"
        n157 = Unbundle By Name(w351) -> ("Data Sample Directory"=w354:path, "GUI Aisle 1"=w355:T1[], "GUI Aisle 1A"=w356:T1[], "GUI Aisle 2"=w357:T1[], "GUI Aisle 3"=w358:T1[], "GUI Aisle 4"=w359:T1[], "Last Save Hour"=w347:string, "Data Sample Filename"=w349:path)
        n158 = call "Counter.vi"() -> ("Count"=→"Samples":dbl)  [unwired: 11 in]
        n159 = Build Array (concatenate)(w355, w356, w357, w358, w359) -> (w360:T1[])
        n160 = call "File Wilt.vi"("Dryer Aisle In"=w360, "Dryer Data Dir"=w354, "RW  Mode"=T11."Write Sample Data", "Last Save Hour"=w347, "error in (no error)"=w353, "Sample Data Current Filename"=w349) -> ("Last Save Hour Out"=w346:string, "Sample Data Current Filename Out"=w343:path, "error out"=w352:errorcluster)  [unwired: 6 in, 1 out]
        n161 = call <vilib>:"Add State(s) to Queue__jki_lib_state_machine.vi"("State(s) in (\"\")"=w362) -> ("States Out"=w361:string)  [unwired: 14 in]
        n162 = Not Equal?(x=w347, y=w346) -> (x != y?=w345:bool)
        n163 = local write "Data Sample Filename"(w343) -> ()
        n164 = Bundle By Name(cluster=w351, "Last Save Hour"=w346, "Data Sample Filename"=w343, "Save Bool"=w345) -> (w350:T12)
      }
      frame "Save Data History" {
        # "Template Separator\n(You can make a copy of, or modify, this frame)"
        n165 = Unbundle By Name(w365) -> ("Save Bool"=w364:bool)
        n166 = case shown="True" w364 {
          frame False {
          }
          frame True {
            # "In 3rd state machine."
            # "In first state machine"
            n167 = local write "Save Setup"(TRUE ("Save Setup")) -> ()
            n168 = property on="Robocopy" class="Bool (strict)"("Val(Sgnl)"=TRUE ("Value (Signaling)")) -> ()  [unwired: 2 in, 2 out]
          }
        }
        n169 = call <vilib>:"Add State(s) to Queue__jki_lib_state_machine.vi"("State(s) in (\"\")"=w367) -> ("States Out"=w366:string)  [unwired: 14 in]
      }
    }
  }
  n170 = while "Main Control Loop" {
    shift-right: [w379] -> _
    shift-left: _ -> [w378]
    shift-right: [w381] -> _
    shift-left: errorcluster {"status"=FALSE, "code"=0, "source"=""} ("error out") -> [w376]
    shift-right: [w380] -> _
    shift-left: w11 -> [w382]
    tunnel: [w375] -> w6
    shift-right: [w373] -> _
    shift-left: string[] [] -> [w372]
    stop <- w375 stop-if-true
    w377 = -1  # Timeout
    n171 = call <vilib>:"Parse State Queue__jki_lib_state_machine.vi"("State Queue"=w382, "Error In (no error)"=w376) -> ("Remaining States"=w384:string, "Current State"=w374:string, "Arguments"=w383:string)  [unwired: 11 in]
    "Current State" <- w374
    n172 = case shown="\"Data: Initialize\"" w374 {
      selector: w374 -> [_ _ _ w431 _ _ _ _ _ _ _ _ w719 _ _ _ _ _ _ _ _ _ _ _ _ _ _ _ _ _ _ _ _ _ _ _ _ _ _ _]
      tunnel: w384 -> [w397 w405 w430 w435 w454 w475 w504 w518 w523 w563 w606 w648 w725 w762 w795 w810 w835 w880 w912 w923 w953 w957 w967 w971 w975 w980 w997 w1124 w1170 w1264 w1311 w1362 w1438 w1643 w1717 w1801 w1884 w2027 w2042 w2134]
      tunnel: w383 -> [_ _ _ _ _ _ _ _ _ _ _ _ _ _ _ _ _ _ w907 w917 _ _ _ _ _ _ _ _ _ _ _ _ _ _ _ _ _ _ _ _]
      tunnel: w378 -> [w398 w403 w427 w433 w445 w470 w501 w508 w520 _ w599 w628 w712 w752 w792 w797 w833 w866 w910 w919 w950 w954 w964 w968 w972 w977 w985 w1122 w1159 w1261 w1304 w1358 w1435 w1641 w1714 w1798 w1882 w2024 w2031 w2129]
      tunnel: [w396 w402 w428 w437 w451 w471 errorcluster {"status"=FALSE, "code"=0, "source"=""} ("error out") w516 w521 w534 w604 w646 w714 w753 w793 w808 w829 w869 w908 w920 w951 w955 w965 w969 w973 w978 w995 w1119 w1155 w1262 w1309 w1359 w1428 w1638 w1706 w1790 w1873 w2025 w2035 w2130] -> w381
      tunnel: w376 -> [w396 w401 w428 w436 w451 w472 w493 w516 w521 w534 w604 w646 w723 w759 w793 w808 w830 w875 w909 w921 w951 w955 w965 w969 w973 w978 w995 w1119 w1168 w1262 w1309 w1359 w1429 w1638 w1707 w1793 w1874 w2025 w2036 w2130]
      tunnel: [w397 w404 w429 w434 w453 w474 w503 w517 w522 w562 w605 w647 w724 w761 w794 w809 w834 w879 w911 w922 w952 w956 w966 w970 w974 w979 w996 w1123 w1169 w1263 w1310 w1361 w1437 w1642 w1716 w1800 w1883 w2026 w2041 w2133] -> w380
      tunnel: [_ _ _ _ _ _ _ TRUE _ _ _ _ _ _ _ _ _ _ _ _ _ _ _ _ _ _ _ _ _ _ _ _ _ _ _ _ _ _ _ _] -> w375
      tunnel: [w398 w400 w427 w433 w452 w470 w501 w508 w520 w561 w603 w628 w709 w756 w792 w798 w833 w860 w910 w919 w950 w954 w964 w968 w972 w977 w992 w1121 w1158 w1260 w1308 w1357 w1434 w1640 w1713 w1797 w1881 w2023 w2030 w2131] -> w379
      tunnel: w377 -> [_ w399 _ _ _ _ _ _ _ _ _ _ _ _ _ _ _ _ _ _ _ _ _ _ _ _ _ _ _ _ _ _ _ _ _ _ _ _ _ _]
      frame "ABOUT" {
        # "Two different scenarios, \n1.  in the big room, we use Agilent for data logging up to 56 dryers simultaneously.\n2.  On the remote stations, we have up to 4 per station."
        # "Wilt testing for dryers."
      }
      frame "", "Idle" {
        n173 = event shown="[2] \"Save Setup\": Value Change" {
          selector: _ -> [_ _ _ _]
          dyn-events: _ -> [_ _ _ _]
          timeout: w399 -> [_ _ _ _]
          tunnel: w405 -> [w409 w415 w420 w426]
          tunnel: [w408 w414 w419 w425] -> w404
          tunnel: w403 -> [w406 w412 w417 w423]
          tunnel: [w407 w413 w418 w424] -> w402
          tunnel: w401 -> [w407 w413 w418 w424]
          tunnel: [w406 w412 w417 w423] -> w400
          event Timeout {
            n174 = event-data() -> ()  [unwired: 1 in, 1 out]
            n175 = call <vilib>:"Add State(s) to Queue__jki_lib_state_machine.vi"("State(s) in (\"\")"=w409) -> ("States Out"=w408:string)  [unwired: 14 in]
          }
          event "Stop Test": Value Change {
            # "Exit Button Value Change (pressed) Event\n(this executes Macro: Exit to terminate the VI)"
            n176 = event-data() -> ()  [unwired: 1 in, 1 out]
            n177 = property on="Stop Test" class="Bool (strict)"("Val(Sgnl)"="Stop Test") -> ()  [unwired: 2 in, 2 out]
            n178 = call <vilib>:"Add State(s) to Queue__jki_lib_state_machine.vi"("State(s) in Front (\"\")"="UI: Save Current State\nMacro: Exit", "State(s) in (\"\")"=w415) -> ("States Out"=w414:string)  [unwired: 13 in]
          }
          event "Save Setup": Value Change {
            # "Exit Button Value Change (pressed) Event\n(this executes Macro: Exit to terminate the VI)"
            n179 = event-data() -> ()  [unwired: 1 in, 1 out]
            n180 = call <vilib>:"Add State(s) to Queue__jki_lib_state_machine.vi"("State(s) in Front (\"\")"="UI: Save Current State\nStart Test", "State(s) in (\"\")"=w420) -> ("States Out"=w419:string)  [unwired: 13 in]
          }
          event Panel Close? {
            # "Discard the event because we'll close the front panel ourselves in Macro: Exit"
            # "Close Panel button (pressed) Event\n(this executes Macro: Exit to terminate the VI)"
            n181 = event-data() -> ()  [unwired: 1 in, 1 out]
            n182 = call <vilib>:"Add State(s) to Queue__jki_lib_state_machine.vi"("State(s) in Front (\"\")"="Exit", "State(s) in (\"\")"=w426) -> ("States Out"=w425:string)  [unwired: 13 in]
            n183 = event-data("Discard?"=TRUE) -> ()  [unwired: 1 in, 1 out]
          }
        }
      }
      frame "---------- Core ----------" {
        # "Do not put any code in this frame.\n(it is a separator no-op)"
        n184 = call <vilib>:"Add State(s) to Queue__jki_lib_state_machine.vi"("State(s) in (\"\")"=w430) -> ("States Out"=w429:string)  [unwired: 14 in]
      }
      frame Default {
        w440 = 42 items=["No error", "Argument error", "Memory is full", "Out of zone", "End of file", "File already open", "Generic file I/O error", "File not found", "File permission error", "Disk is full", "Duplicate path", "Too many files open", "System feature not enabled", "Resource file not found", "Cannot add resource", "Resource not found", "Image not found", "Image memory error", "Pen does not exist", "Config type invalid", "Config token not found", "Config parse error", "Config memory error", "Bad external code format", "Bad external code offset", "External code not present", "Null window", "Destroy window error", "Null menu", "Print aborted", "Bad print record", "Print driver error", "Windows error during printing", "Memory error during printing", "Print dialog error", "Generic print error", "Invalid device refnum", "Device not found", "Device parameter error", "Device unit error", "Cannot open device", "Device call aborted", "Generic error", "Cancelled by user", "Object ID too low", "Object ID too high", "Object not in heap", "Unknown heap", "Unknown object (invalid DefProc)", "Unknown object (DefProc not in table)", "Message out of range", "Invalid (null) method", "Unknown message", "Manager call not supported", "Bad address", "Network operation in progress", "Network operation timed out", "Connection is busy", "Network attribute not supported", "Network error", "Address in use", "System out of memory", "Connection aborted", "Connection refused", "Not connected", "Already connected", "Connection closed", "Initialization error (interapplication manager)", "Bad occurrence", "Wait on unbound occurrence handler", "Occurrence queue overflow", "Datalog type conflict", "Unused", "Unrecognized type (interapplication manager)", "Memory corrupt", "Failed to make temporary DLL", "Old CIN version", "Drag socket not found", "Failed to load drop-object", "Failed to register OLE object", "Failed to release OLE object", "Format specifier type mismatch", "Unknown format specifier", "Too few format specifiers", "Too many format specifiers", "Scan failed", "Newer CIN version", "Error converting to variant", "Runtime menu error", "Password tampered", "Variant attribute not found", "Incompatible variant data type", "Event data is not available", "Event Store is not present", "Occurrence is not found", "Event Queue is not created", "Event info is not available", "Refnum passed is NULL", "Error retrieving Class GUID", "Error retrieving CoClass GUID", "Error retrieving TypeLib GUID.", "Bad built application magic bytes.", "Specific driver is different from the specific driver associated with the Logical Name.", "There is no session opened to the class driver.", "Max Error", "MAX - Error with config objects", "MAX - Error loading configuration", "MAX - Group not supported"]
        # "Current State"
        # "Do not delete, rename, or modify this frame.\n(this is used to capture unhandled states and typos)"
        # "Handle mistyped state name (developer tool)"
        n185 = Format Into String(format string="Software Exception: Unhandled State \"%s\"." ("message"), error in=w436, w431) -> (resulting string=w439:string, error out=w438:errorcluster)  [unwired: 1 in]
        n186 = call <vilib>:"Error Cluster From Error Code.vi"("show call chain? (False)"=TRUE, "error in (no error)"=w438, "error message (\"\")"=w439, "error code (0)"=w440) -> ("error out"=w437:errorcluster)  [unwired: 5 in]
        n187 = call <vilib>:"Add State(s) to Queue__jki_lib_state_machine.vi"("State(s) in (\"\")"=w435) -> ("States Out"=w434:string)  [unwired: 14 in]
      }
      frame "Initialize Core Data" {
        w442 = FALSE ("Tool Bar:Show Abort Button")
        # "Do not delete, rename, or modify this frame.\n(this is used to determine panel behavior on exit)"
        # "originally closed?"
        # "exe?"
        # "If panel starts closed or is an EXE, then close it when we exit"
        n188 = property class="VI"() -> ("Front Panel.Open"=w450:bool)  [unwired: 2 in, 2 out]
        n189 = Not(x=w450) -> (.not. x?=w447:bool)
        n190 = control-ref of="Current VI Reference"() -> (w443:refnum<vi>)
        n191 = property class="App"() -> ("App.Kind"=w449:T10)  [unwired: 2 in, 2 out]
        n192 = Equal?(x=w449, y=T10."Run Time System" ("Application:Kind")) -> (x = y?=w446:bool)
        n193 = Or(x=w447, y=w446) -> (x .or. y?=w444:bool)
        n194 = Bundle By Name(cluster=w445, "Core.Current VI Reference"=w443, "Core.Close Panel on Exit?"=w444) -> (w452:T16)
        n195 = property class="VI"(reference=w443, "TB.ShowAbortBut"=w442, "TB.ShowFreeRunBut"=w442) -> ()  [unwired: 1 in, 2 out]
        n196 = call <vilib>:"Add State(s) to Queue__jki_lib_state_machine.vi"("State(s) in (\"\")"=w454) -> ("States Out"=w453:string)  [unwired: 14 in]
      }
      frame "Data: Cleanup" {
        # "Cleanup any data and references, here.\n(this is called automatically, by the Macro: Exit)"
        n197 = Unbundle By Name(w470) -> ("Remote Station"=w455:bool, "USB6008"=w458:tag, "Agilent Channels Water Valves."=w457:T3[], "All Test Stations Control"=w459:T1[], "Core.Current VI Reference"=w473:refnum<vi>)
        n198 = local read "3"() -> (w460:T9)
        n199 = call <vilib>:"Release Semaphore Reference.vi"("semaphore"=w460) -> ("error out"=w467:errorcluster)  [unwired: 9 in, 1 out]
        n200 = local read "2"() -> (w461:T9)
        n201 = call <vilib>:"Release Semaphore Reference.vi"("error in (no error)"=w467, "semaphore"=w461) -> ("error out"=w468:errorcluster)  [unwired: 8 in, 1 out]
        n202 = local read "1A"() -> (w462:T9)
        n203 = call <vilib>:"Release Semaphore Reference.vi"("error in (no error)"=w468, "semaphore"=w462) -> ()  [unwired: 8 in, 2 out]
        n204 = Close Reference(reference=w473, error in (no error)=w472) -> (error out=w471:errorcluster)
        n205 = for {
          tunnel: w459 -> [w481] mode=indexing
          tunnel: w458 -> [w479]
          tunnel: w457 -> [w478]
          tunnel: [w477] -> w456
          tunnel: w455 -> [w476]
          n206 = Unbundle By Name(w481) -> ("Station Index"=w480:i32)
          n207 = case shown="False" w476 {
            tunnel: w480 -> [w486 w491]
            tunnel: [w483 _] -> w477
            tunnel: w478 -> [w482 _]
            tunnel: w479 -> [_ w488]
            frame False {
              # "Turn off valve"
              n208 = local read "Agilent"() -> (w484:T9)
              n209 = Number To Decimal String(number=w486) -> (decimal integer string=w485:string)  [unwired: 1 in]
              n210 = call "Agilent Valve Control.vi"("Station In"=w485, "Agilent Channels In"=w482, "Agilent"=w484, "Open/Close (F:Close)"=TRUE) -> ("error out"=w483:errorcluster)  [unwired: 9 in, 2 out]
            }
            frame True {
              # "Turn off valve"
              n211 = To Long Integer(number=w491) -> (32bit integer=w490:i32)
              n212 = call "Valve Control Single 6008.vi"("Valve On?"=FALSE, "Valve Number"=w490, "Port"=w488) -> ()  [unwired: 8 in, 1 out]
            }
          }
        }
        n213 = call <vilib>:"Add State(s) to Queue__jki_lib_state_machine.vi"("State(s) in (\"\")"=w475) -> ("States Out"=w474:string)  [unwired: 14 in]
        n214 = local read "Agilent"() -> (w465:T9)
        n215 = local read "1"() -> (w463:T9)
        n216 = call <vilib>:"Release Semaphore Reference.vi"("error in (no error)"=w456, "semaphore"=w463) -> ("error out"=w469:errorcluster)  [unwired: 8 in, 1 out]
        n217 = call <vilib>:"Release Semaphore Reference.vi"("error in (no error)"=w469, "semaphore"=w465) -> ("error out"=w466:errorcluster)  [unwired: 8 in, 1 out]
        n218 = local read "4"() -> (w464:T9)
        n219 = call <vilib>:"Release Semaphore Reference.vi"("error in (no error)"=w466, "semaphore"=w464) -> ()  [unwired: 8 in, 2 out]
      }
      frame "Error Handler" {
        # "Handle any errors here.\nYou can also output any states to clean-up after errors occur"
        # "Clear error"
        n220 = local read "Debug"() -> (w492:bool)
        n221 = case shown="True" w492 {
          tunnel: w493 -> [_ w505]
          frame False {
          }
          frame True {
            # "Unhandled Error -- Display it"
            n222 = call <vilib>:"General Error Handler.vi"("error in (no error)"=w505) -> ()  [unwired: 10 in, 5 out]
          }
        }
        n223 = local read "Control Error List"() -> (w499:string)
        n224 = Unbundle By Name(w493) -> ("source"=w497:string)
        n225 = Concatenate Strings("ERROR(control): " ("string"), w497) -> (w495:string)
        n226 = Concatenate Strings(w497, "\n", w499) -> (→"Control Error List":string)
        n227 = local write "User Notice"(w495) -> ()
        n228 = call <vilib>:"Add State(s) to Queue__jki_lib_state_machine.vi"("State(s) in Front (\"\")"="/* Post Error States", "State(s) in (\"\")"=w504) -> ("States Out"=w503:string)  [unwired: 13 in]
      }
      frame "Exit" {
        # "Do not put any code in this frame.\n(No errors that occur here will be handled.)"
        n229 = Unbundle By Name(w508) -> ("Agilent Refs"=w507:refnum<visa-resource-name>[], "Water Times Filepath"=w506:path)
        n230 = local read "Aisle 2 (21-32)"() -> (w513:dbl[])
        n231 = local read "Aisle 3 (33-44)"() -> (w512:dbl[])
        n232 = local read "Aisle 4 (45-56)"() -> (w511:dbl[])
        n233 = local read "Aisle 1 (1-20)"() -> (w514:dbl[])
        n234 = Build Array (concatenate)(w514, w513, w512, w511) -> (w510:dbl[])
        n235 = call-poly <vilib>:"Write To Spreadsheet File.vi"("delimiter (\\t)"="," ("delimiter (\\t)"), "1D data"=w510, "file path (dialog if empty)"=w506) -> ()  [unwired: 5 in, 1 out]
        n236 = for {
          tunnel: w507 -> [w519] mode=indexing
          n237 = VISA Close(VISA resource name=w519) -> ()  [unwired: 1 in, 1 out]
        }
        n238 = call <vilib>:"Add State(s) to Queue__jki_lib_state_machine.vi"("State(s) in (\"\")"=w518) -> ("States Out"=w517:string)  [unwired: 14 in]
      }
      frame "---------- Init ----------" {
        # "Do not put any code in this frame.\n(It is a separator no-op. You can make a copy of this frame to create a new Data frame)"
        n239 = call <vilib>:"Add State(s) to Queue__jki_lib_state_machine.vi"("State(s) in (\"\")"=w523) -> ("States Out"=w522:string)  [unwired: 14 in]
      }
      frame "Data: Initialize" {
        w559 = refnum<visa-resource-name>[] ["AGILENT1", "AGILENT2", "AGILENT3", "AGILENT4", "AGILENT5", "AGILENT6"] ("Agilent Refs")
        # "Either 4 or 56 water times in file."
        # "Data names and types of shift register data are defined by this bundle."
        # "Initialize the shift-register data, here.\n(data names are defined by what you wire into the bundle function)"
        n240 = local read "Remote Station"() -> (w529:bool)
        n241 = call <vilib>:"Check if File or Folder Exists.vi"("path"="Water Times Filepath") -> ("file or folder exists?"=w543:bool)  [unwired: 8 in, 2 out]
        n242 = case shown="True" w543 {
          tunnel: [dbl[] [] ("all rows") w571] -> w549
          tunnel: "Water Times Filepath" -> [_ w568]
          frame False {
          }
          frame True {
            n243 = call-poly <vilib>:"Read From Spreadsheet File.vi"("delimiter (\\t)"="," ("delimiter (\\t)"), "file path (dialog if empty)"=w568) -> ("all rows"=w570:dbl[][])  [unwired: 5 in, 4 out]
            n244 = Index Array(array=w570, index (row)=0 ("disabled index (col)")) -> (element=w571:dbl[])  [unwired: 1 in]
          }
        }
        n245 = local write "valve error out"(w534) -> ()
        n246 = Select(t="C:\\Data\\", s=w529, f="D:\\Data\\") -> (s? t:f=w538:string)
        n247 = Concatenate Strings(w538, "Wilt Backup.ini") -> (w537:string)
        n248 = String To Path(string=w537) -> (path=w536:path)
        n249 = Array Size(array=w549) -> (size(s)=w548:i32)
        n250 = case shown="56" w548 {
          tunnel: w549 -> [_ w589 w591]
          tunnel: [w575 w580 w591] -> w544
          tunnel: [w572 w579 w590] -> w545
          tunnel: [w572 w578 w590] -> w546
          tunnel: [w572 w577 w590] -> w547
          frame 0, Default {
            w573 = 64.6 ("element")
            n251 = Initialize Array(w573, 12 ("dimension size")) -> (w572:dbl[])
            n252 = Initialize Array(w573, 20 ("dimension size")) -> (w575:dbl[])
          }
          frame 56 {
            n253 = Delete From Array(array=w589, length=20, index=0) -> (deleted portion=w580:dbl[], array with subset deleted=w584:dbl[])
            n254 = Delete From Array(array=w584, length=12, index=0) -> (deleted portion=w579:dbl[], array with subset deleted=w581:dbl[])
            n255 = Delete From Array(array=w581, length=12, index=0) -> (deleted portion=w578:dbl[], array with subset deleted=w577:dbl[])
          }
          frame 4 {
            w590 = dbl[] [] ("all rows")
          }
        }
        n256 = flat-sequence {
          tunnel: w536 -> [w564]
          tunnel: [w565] -> w535
          frame #0 {
            "Dryer Bank Filename" <- w564
          }
          frame #1 {
            n257 = local read "Dryer Bank Filename"() -> (w565:path)
          }
        }
        n258 = local write "DAQ error out"(w534) -> ()
        n259 = local write "User Notice"("Initializing..." ("User Notice")) -> ()
        n260 = local write "Aisle 4 (45-56)"(w547) -> ()
        n261 = local write "Aisle 3 (33-44)"(w546) -> ()
        n262 = local write "Aisle 2 (21-32)"(w545) -> ()
        n263 = local write "Aisle 1 (1-20)"(w544) -> ()
        n264 = local read "All Confgured Com Array"() -> (w528:u8[])
        n265 = local write "Tab Control 2"(enum32{"Configuration", "Main"}."Main" ("Tab Control 2")) -> ()
        n266 = Bundle("Water Times Filepath"="Water Times Filepath", "Core"=T13 {"Current VI Reference"=refnum, "Close Panel on Exit?"=FALSE}, "Agilent Refs"=w559, "GUI Aisle 4"="GUI Aisle 4", "GUI Aisle 3"="GUI Aisle 3", "GUI Aisle 2"="GUI Aisle 2", "GUI Aisle 1A"="GUI Aisle 1A", "GUI Aisle 1"="GUI Aisle 1", "Station Timer"="Station Timer", "Station Test State"="Station Test State", "Saved Test State"="Saved Test State", "Dryer Bank Filename"=w535, "Station Com List"="Station Com List", "Start Buttons."="Start Buttons.", "Agilent Channels Water Valves."="Agilent Channels Water Valves.", "Pause Timer"="Pause Timer", "Remote Station"=w529, "All Confgured Com Array"=w528, "All Test Stations Control"="All Test Stations Control", "USB6008"="USB6008", "Emergency Timer"="Emergency Timer") -> (w561:T16)  [unwired: 1 in]
        n267 = call <vilib>:"Add State(s) to Queue__jki_lib_state_machine.vi"("State(s) in (\"\")"=w563) -> ("States Out"=w562:string)  [unwired: 14 in]
        "All Agilent Refs" <- w559
      }
      frame "Init: Test States" {
        # "If State is Wait Com, set timer for first broadcast."
        # "Initialization Macro\n(This is called once, when the VI starts)"
        n268 = Unbundle By Name(w599) -> ("Station Test State"=w598:T8[], "GUI Aisle 1"=w596:T1[], "GUI Aisle 1A"=w595:T1[], "GUI Aisle 2"=w594:T1[], "GUI Aisle 3"=w593:T1[], "GUI Aisle 4"=w592:T1[])
        n269 = Build Array (concatenate)(w596, w595, w594, w593, w592) -> (w602:T1[])
        n270 = for {
          tunnel: w602 -> [w621] mode=indexing
          tunnel: [w607] -> w597 mode=indexing
          tunnel: [w613] -> w601 mode=indexing
          tunnel: [w612] -> w600 mode=indexing
          tunnel: w598 -> [w611] mode=indexing
          w609 = Dryer_Test_State."Com Fault" ("Test State")
          n271 = Unbundle By Name(w621) -> ("Lab ID"=w620:string, "Com Port"=w612:u8)
          n272 = Equal?(x=w620, y="") -> (x = y?=w616:bool)
          n273 = Select(t=Dryer_Test_State."No SN" ("Test State"), s=w616, f=Dryer_Test_State."Wait Com" ("Test State")) -> (s? t:f=w608:T8)
          n274 = Equal?(x=w609, y=w611) -> (x = y?=w610:bool)
          n275 = call "E-Time.vi"() -> ("Elapsed Time (sec)"=w614:dbl)  [unwired: 9 in, 2 out]
          n276 = Select(t=w609, s=w610, f=w608) -> (s? t:f=w607:T8)
          n277 = Select(t=0.0, s=w616, f=w614) -> (s? t:f=w613:dbl)
        }
        n278 = local write "Station Test State"(w597) -> ()
        n279 = Bundle By Name(cluster=w599, "Saved Test State"=w597, "Station Test State"=w597, "Station Timer"=w601, "Station Com List"=w600) -> (w603:T16)
        n280 = local write "Station Com List"(w600) -> ()
        n281 = call <vilib>:"Add State(s) to Queue__jki_lib_state_machine.vi"("State(s) in (\"\")"=w606) -> ("States Out"=w605:string)  [unwired: 14 in]
      }
      frame "Init: Station Numbers" {
        w629 = Update_Wilt_GUI_Control."Init Station Number" ("Enum")
        # "Stations 45-56"
        # "Stations 33-44"
        # "Stations 21-32"
        # "Stations 13-20"
        # "Stations 1-12"
        # "Initialization Macro\nINIT COM PORT AND STATION NUMBER."
        n282 = Unbundle By Name(w628) -> ("GUI Aisle 1"=w627:T1[], "GUI Aisle 1A"=w626:T1[], "GUI Aisle 2"=w625:T1[], "GUI Aisle 3"=w624:T1[], "GUI Aisle 4"=w623:T1[], "All Confgured Com Array"=w622:u8[])
        n283 = local read "Station Labels"() -> (w641:string[])
        n284 = call "Parse Labels and Com Arrays.vi"("All Confgured Com Array"=w622, "Station Labels"=w641) -> ("Labels1"=w640:string[], "Com1"=w639:u8[], "Labels1A"=w638:string[], "Com1a"=w637:u8[], "Labels2"=w636:string[], "Com2"=w635:u8[], "Labels3"=w634:string[], "Com4"=w631:u8[], "Labels4"=w632:string[], "Com3"=w633:u8[])  [unwired: 4 in]
        n285 = for {
          tunnel: w627 -> [w698] mode=indexing
          tunnel: [w705] -> w642 mode=indexing
          tunnel: w629 -> [w704]
          tunnel: w640 -> [w703] mode=indexing
          tunnel: w639 -> [w702] mode=indexing
          i -> [w701]
          n286 = Unbundle By Name(w698) -> ("Dryer Details.24 Hour Water Injection"=w697:i32)
          n287 = case shown="0, Default" w697 {
            tunnel: [w706 TRUE ("Day")] -> w699
            frame 0, Default {
              n288 = local read "Day"() -> (w706:bool)
            }
            frame 1 {
            }
          }
          n289 = Increment(x=w701) -> (x+1=w700:i32)
          n290 = call "Update Wilt GUI.vi"("Dryer In"=w698, "Day Shift?"=w699, "Enum"=w704, "Station Index"=w700, "Station Label In"=w703, "Com Port In"=w702) -> ("Dryer Out 2"=w705:T1)  [unwired: 7 in, 2 out]
        }
        n291 = for {
          tunnel: w626 -> [w686] mode=indexing
          tunnel: [w694] -> w643 mode=indexing
          tunnel: w629 -> [w693]
          tunnel: w638 -> [w692] mode=indexing
          tunnel: w637 -> [w691] mode=indexing
          i -> [w690]
          n292 = Unbundle By Name(w686) -> ("Dryer Details.24 Hour Water Injection"=w685:i32)
          n293 = case shown="0, Default" w685 {
            tunnel: [w695 TRUE ("Day")] -> w687
            frame 0, Default {
              n294 = local read "Day"() -> (w695:bool)
            }
            frame 1 {
            }
          }
          n295 = Add(x=13 ("y"), y=w690) -> (x+y=w688:i32)
          n296 = call "Update Wilt GUI.vi"("Dryer In"=w686, "Day Shift?"=w687, "Enum"=w693, "Station Index"=w688, "Station Label In"=w692, "Com Port In"=w691) -> ("Dryer Out 2"=w694:T1)  [unwired: 7 in, 2 out]
        }
        n297 = for {
          tunnel: w625 -> [w674] mode=indexing
          tunnel: [w682] -> w645 mode=indexing
          tunnel: [w676] -> _
          tunnel: w636 -> [w681] mode=indexing
          tunnel: w635 -> [w680] mode=indexing
          tunnel: w629 -> [w676]
          i -> [w678]
          n298 = Unbundle By Name(w674) -> ("Dryer Details.24 Hour Water Injection"=w673:i32)
          n299 = case shown="0, Default" w673 {
            tunnel: [w683 TRUE ("Day")] -> w675
            frame 0, Default {
              n300 = local read "Day"() -> (w683:bool)
            }
            frame 1 {
            }
          }
          n301 = Add(x=21 ("y"), y=w678) -> (x+y=w677:i32)
          n302 = call "Update Wilt GUI.vi"("Dryer In"=w674, "Day Shift?"=w675, "Enum"=w676, "Station Index"=w677, "Station Label In"=w681, "Com Port In"=w680) -> ("Dryer Out 2"=w682:T1)  [unwired: 7 in, 2 out]
        }
        n303 = for {
          tunnel: w624 -> [w662] mode=indexing
          tunnel: [w670] -> w644 mode=indexing
          tunnel: w629 -> [w669]
          tunnel: w634 -> [w668] mode=indexing
          tunnel: w633 -> [w667] mode=indexing
          i -> [w665]
          n304 = Unbundle By Name(w662) -> ("Dryer Details.24 Hour Water Injection"=w661:i32)
          n305 = case shown="0, Default" w661 {
            tunnel: [w671 TRUE ("Day")] -> w663
            frame 0, Default {
              n306 = local read "Day"() -> (w671:bool)
            }
            frame 1 {
            }
          }
          n307 = Add(x=33 ("y"), y=w665) -> (x+y=w664:i32)
          n308 = call "Update Wilt GUI.vi"("Dryer In"=w662, "Day Shift?"=w663, "Enum"=w669, "Station Index"=w664, "Station Label In"=w668, "Com Port In"=w667) -> ("Dryer Out 2"=w670:T1)  [unwired: 7 in, 2 out]
        }
        n309 = for {
          tunnel: w623 -> [w650] mode=indexing
          tunnel: [w658] -> w630 mode=indexing
          tunnel: w629 -> [w657]
          tunnel: w632 -> [w656] mode=indexing
          tunnel: w631 -> [w655] mode=indexing
          i -> [w654]
          n310 = Unbundle By Name(w650) -> ("Dryer Details.24 Hour Water Injection"=w649:i32)
          n311 = case shown="0, Default" w649 {
            tunnel: [w659 TRUE ("Day")] -> w651
            frame 0, Default {
              n312 = local read "Day"() -> (w659:bool)
            }
            frame 1 {
            }
          }
          n313 = Add(x=w654, y=45) -> (x+y=w652:i32)
          n314 = call "Update Wilt GUI.vi"("Dryer In"=w650, "Day Shift?"=w651, "Enum"=w657, "Station Index"=w652, "Station Label In"=w656, "Com Port In"=w655) -> ("Dryer Out 2"=w658:T1)  [unwired: 7 in, 2 out]
        }
        n315 = local write "GUI Aisle 1A"(w643) -> ()
        n316 = local write "GUI Aisle 1"(w642) -> ()
        n317 = local write "GUI Aisle 2"(w645) -> ()
        n318 = local write "GUI Aisle 3"(w644) -> ()
        n319 = local write "GUI Aisle 4"(w630) -> ()
        n320 = call <vilib>:"Add State(s) to Queue__jki_lib_state_machine.vi"("State(s) in (\"\")"=w648) -> ("States Out"=w647:string)  [unwired: 14 in]
      }
      frame "Agilent: Initialize" {
        # "Do not put any code in this frame.\n(It is a separator no-op. You can make a copy of this frame to create a new Data frame)"
        n321 = Unbundle By Name(w712) -> ("Agilent Refs"=w720:refnum<visa-resource-name>[])
        n322 = call "Agilent Channels.vi"("file path (dialog if empty)"="Agilent Channel Assignment") -> ("Temperature Channels"=→"Temperature Channels":T3[], "Station Data Headers"=→"Agilent Station Data Headers":string[][], "Index Array"=→"Agilent Station Data Index Array":i32[][], "Agilent Channels To Read"=w715:T3[], "Start Buttons"=w708:T3[], "Agilent Channel Water Valves"=w711:T3[])  [unwired: 8 in, 1 out]
        "Agilent Read Channels Array" <- w715
        "Agilent Channels Water Valves" <- w711
        "Start Buttons" <- w708
        n323 = for {
          tunnel: w720 -> [w728] mode=indexing
          tunnel: w715 -> [w731]
          shift-right: [w729] -> w717
          shift-left: refnum<visa-resource-name>[] [] -> [w727]
          shift-right: [w735] -> w714
          shift-left: w723 -> [w734]
          i -> [w733]
          n324 = Increment(x=w733) -> (x+1=w732:i32)
          n325 = call "Init Agilent Channels Wilt.vi"("Agilent Number"=w732, "VISA Resource Name"=w728, "Agilent Channels Array"=w731, "error in (no error)"=w734) -> ("Number of Read Channels"=w730:i32, "error out"=w735:errorcluster)  [unwired: 10 in]
          n326 = Greater Than 0?(x=w730) -> (x > 0?=w726:bool)
          n327 = case shown="True" w726 {
            tunnel: [w736 w739] -> w729
            tunnel: w728 -> [_ w738]
            tunnel: w727 -> [w736 w737]
            frame False {
            }
            frame True {
              n328 = Build Array (concatenate)(w737, w738) -> (w739:refnum<visa-resource-name>[])
            }
          }
        }
        "Agilent Read Refs" <- w717
        n329 = Bundle By Name(cluster=w712, "Start Buttons."=w708, "Agilent Channels Water Valves."=w711) -> (w709:T16)
        n330 = case shown="No Error" w714 {
          selector: w714 -> [_ w743]
          tunnel: w719 -> [_ w744]
          tunnel: [_ w740] -> w713
          frame No Error {
          }
          frame Error {
            n331 = Unbundle By Name(w743) -> ("source"=w742:string)
            n332 = disable-structure shown="Enabled" {
              disable-tunnel: ["Macro: Exit" ("State(s) in Front (\"\")") _] -> w740
              frame Disabled {
                n333 = property on="Stop Test" class="Bool (strict)"("Val(Sgnl)"=TRUE ("Value (Signaling)")) -> ()  [unwired: 2 in, 2 out]
              }
              frame Enabled {
              }
            }
            n334 = Concatenate Strings("Error with Agilents: " ("string"), w744, w742) -> (w741:string)
            n335 = One Button Dialog(message=w741) -> ()  [unwired: 1 in, 1 out]
          }
        }
        n336 = call <vilib>:"Add State(s) to Queue__jki_lib_state_machine.vi"("State(s) in Front (\"\")"=w713, "State(s) in (\"\")"=w725) -> ("States Out"=w724:string)  [unwired: 13 in]
      }
      frame "Com: Initialize" {
        # "Ignore Init Errors"
        # "Fixme! once com [oprts in"
        # "Do not put any code in this frame.\nInitialize all the com ports to GEA2 specs."
        n337 = Unbundle By Name(w752) -> ("All Confgured Com Array"=w751:u8[])
        n338 = call "Find Valid Com Ports.vi"("Valid Com Port List(100,2:56)"=w751) -> ("Valid Com Ports"=w760:refnum<visa-resource-name>[])  [unwired: 13 in, 1 out]
        n339 = for {
          N: 10 -> [_]
          tunnel: w760 -> [w769]
          tunnel: w759 -> [w768]
          tunnel: u8[] [] ("All Com Array") -> [w767]
          tunnel: [w766] -> w757
          tunnel: [w765] -> w755
          tunnel: [w764] -> w754
          tunnel: [w763] -> w750
          n340 = for {
            tunnel: w769 -> [w776] mode=indexing
            tunnel: w768 -> [w778]
            tunnel: [w771] -> w764
            shift-right: [w775] -> w763
            shift-left: w767 -> [w774]
            tunnel: [w773] -> w766 mode=indexing
            tunnel: [w772] -> w765 mode=indexing
            n341 = call "GEA2_ICP_Dryer_SM.vi"("ComPort"=w776, "Mode"=GEA2_Dryer_Interface_Ctrl."Init Com Port", "Error In"=w778) -> ("Dryer Status Serial Data Out"=w773:T5, "Error Out"=w771:errorcluster)  [unwired: 7 in, 4 out]
            n342 = case shown="No Error" w771 {
              tunnel: w776 -> [w782 w784]
              tunnel: [w781 w786] -> w775
              tunnel: w774 -> [w783 w785]
              tunnel: [Dryer_Test_State."No SN" ("Test State") Dryer_Test_State."Com Fault" ("Test State")] -> w772
              frame No Error {
                n343 = call "Com Chan Type Conversion.vi"("Com Chan In"=w782) -> ("Com Channel #"=w780:u8)  [unwired: 11 in, 3 out]
                n344 = Build Array (concatenate)(w783, w780) -> (w781:u8[])
              }
              frame Error {
                w791 = "COM Init Error.  "
                n345 = call "Com Chan Type Conversion.vi"("Com Chan In"=w784) -> ("Com Channel #"=w787:u8)  [unwired: 11 in, 3 out]
                n346 = Build Array (concatenate)(w785, w787) -> (w786:u8[])
                n347 = Type Cast(type=w791, x=w784) -> (*(type *) &x=w789:string)
                n348 = Concatenate Strings(w791, w789) -> (w790:string)
                n349 = One Button Dialog(message=w790) -> ()  [unwired: 1 in, 1 out]
              }
            }
            n350 = Wait Until Next ms Multiple(millisecond multiple=u32 20) -> ()  [unwired: 1 out]
          }
        }
        n351 = local write "User Notice"("Sending Start Commands" ("User Notice")) -> ()
        n352 = call <vilib>:"Clear Errors.vi"("error in (no error)"=w754) -> ("error out"=w753:errorcluster)  [unwired: 6 in]
        n353 = local write "All Confgured Com Array"(w750) -> ()
        n354 = local write "Station Test State"(w755) -> ()
        n355 = Bundle By Name(cluster=w752, "Station Test State"=w755, "All Confgured Com Array"=w750) -> (w756:T16)
        n356 = call <vilib>:"Add State(s) to Queue__jki_lib_state_machine.vi"("State(s) in (\"\")"=w762) -> ("States Out"=w761:string)  [unwired: 14 in]
        n357 = local write "Dryer Com Info"(w757) -> ()
      }
      frame "---------- UI ----------" {
        # "Do not put any code in this frame.\n(It is a separator no-op. You can make a copy of this frame to create a new UI frame)"
        n358 = call <vilib>:"Add State(s) to Queue__jki_lib_state_machine.vi"("State(s) in (\"\")"=w795) -> ("States Out"=w794:string)  [unwired: 14 in]
      }
      frame "UI: Initialize" {
        w800 = T1 {"Lab ID"="", "Day Cycle Count"=0, "Station Label"="", "Dryer Details"={"Station"="", "Cycle Count Day"="", "Status"="", "Debug ASCII"="", "Notes"="", "Lab ID"="", "Total Time On"="", "TR Number"="", "Cycle Count Night"="", "Time On Day"="", "Time On Night"="", "Run w/o Newfi"=0, "24 Hour Water Injection"=0, "Stop Dryer"=0}, "Sample Record "=[], "Hist Record "=[], "Status Color"=0, "Boolean"=FALSE, "Com Port"=0, "Bad Com Count"=0, "Current Run Start Time"=0.0, "Night Cycle Count"=0, "Station Index"=0, "Cycle Index"="", "Audit Alert"=FALSE}  # Initial Dryer Cluster
        # "Initialize the User Interface, here.\n(this is called automatically, by the Macro: Init)"
        n359 = global read "Globals Wilt.vi" "Temperature Fault"() -> (→"Temperature Fault":u32)
        n360 = global read "Globals Wilt.vi" "No Com Color"() -> (→"No Com":u32)
        n361 = global read "Globals Wilt.vi" "Stopped Color"() -> (→"Stopped":u32)
        n362 = global read "Globals Wilt.vi" "Running Color"() -> (→"Running":u32)
        n363 = global read "Globals Wilt.vi" "UnConfigured"() -> (→"Unused":u32)
        n364 = global read "Globals Wilt.vi" "Paused Color"() -> (→"Paused":u32)
        n365 = global read "Globals Wilt.vi" "Fault Color"() -> (→"Fault":u32)
        n366 = Unbundle By Name(w797) -> ("Remote Station"=w796:bool)
        n367 = Not(x=w796) -> (.not. x?=w801:bool)
        n368 = property on="GUI Aisle 4" class="Arr (strict)"("Visible"=w801) -> ()  [unwired: 2 in, 2 out]
        n369 = property on="GUI Aisle 2" class="Arr (strict)"("Visible"=w801) -> ()  [unwired: 2 in, 2 out]
        n370 = property on="GUI Aisle 1A" class="Arr (strict)"("Visible"=w801) -> ()  [unwired: 2 in, 2 out]
        n371 = property on="GUI Aisle 3" class="Arr (strict)"("Visible"=w801) -> ()  [unwired: 2 in, 2 out]
        n372 = case shown="False" w796 {
          tunnel: w801 -> [_ _]
          tunnel: w800 -> [w817 w822]
          tunnel: w797 -> [w816 w821]
          tunnel: [w815 w820] -> w798
          frame False {
            w812 = u32 8 ("Len of 1A")
            w813 = u32 12 ("Len of Ailes")
            n373 = Initialize Array(w817, w813) -> (w811:T1[])
            n374 = Initialize Array(w817, w812) -> (w814:T1[])
            n375 = property on="GUI Aisle 3" class="Arr (strict)"("Number of Columns"=w813) -> ()  [unwired: 2 in, 2 out]
            n376 = property on="GUI Aisle 2" class="Arr (strict)"("Number of Columns"=w813) -> ()  [unwired: 2 in, 2 out]
            n377 = property on="GUI Aisle 1" class="Arr (strict)"("Number of Columns"=w813) -> ()  [unwired: 2 in, 2 out]
            n378 = property on="GUI Aisle 4" class="Arr (strict)"("Number of Columns"=w813) -> ()  [unwired: 2 in, 2 out]
            n379 = property on="GUI Aisle 1A" class="Arr (strict)"("Number of Columns"=w812) -> ()  [unwired: 2 in, 2 out]
            n380 = Bundle By Name(cluster=w816, "GUI Aisle 1A"=w814, "GUI Aisle 1"=w811, "GUI Aisle 2"=w811, "GUI Aisle 3"=w811, "GUI Aisle 4"=w811) -> (w815:T16)
          }
          frame True {
            w819 = T1[] [] ("GUI Aisle 1A")
            w823 = u32 4 ("Number of Rows")
            n381 = Initialize Array(w822, w823) -> (w818:T1[])
            n382 = property on="GUI Aisle 1" class="Arr (strict)"("Number of Columns"=w823) -> ()  [unwired: 2 in, 2 out]
            n383 = Bundle By Name(cluster=w821, "GUI Aisle 1A"=w819, "GUI Aisle 1"=w818, "GUI Aisle 2"=w819, "GUI Aisle 3"=w819, "GUI Aisle 4"=w819) -> (w820:T16)
          }
        }
        n384 = call <vilib>:"Add State(s) to Queue__jki_lib_state_machine.vi"("State(s) in (\"\")"=w810) -> ("States Out"=w809:string)  [unwired: 14 in]
      }
      frame "UI: Save Current State" {
        # "Initialize the User Interface, here.\n(this is called automatically, by the Macro: Init)"
        n385 = flat-sequence {
          tunnel: [string[] ["Aisle1", "Aisle1A", "Aisle2", "Aisle3", "Aisle4"]] -> w832
          frame #0 {
            n386 = local read "User Notice"() -> (w839:string)
            n387 = Concatenate Strings(w839, "Saving Setup:  ") -> (w841:string)
            n388 = local write "User Notice"(w841) -> ()
          }
        }
        n389 = Unbundle By Name(w833) -> ("Dryer Bank Filename"=w831:path, "GUI Aisle 1"=w828:T1[], "GUI Aisle 1A"=w827:T1[], "GUI Aisle 2"=w826:T1[], "GUI Aisle 3"=w825:T1[], "GUI Aisle 4"=w824:T1[])
        n390 = for {
          tunnel: w832 -> [w853] mode=indexing
          tunnel: w831 -> [w851]
          shift-right: [w849] -> w829
          shift-left: w830 -> [w850]
          tunnel: w828 -> [w847]
          tunnel: w827 -> [w846]
          tunnel: w826 -> [w845]
          tunnel: w825 -> [w844]
          tunnel: w824 -> [w843]
          i -> [w854]
          n391 = case shown="0, Default" w854 {
            tunnel: [w855 w856 w857 w858 w859] -> w852
            tunnel: w847 -> [w855 _ _ _ _]
            tunnel: w846 -> [_ w856 _ _ _]
            tunnel: w845 -> [_ _ w857 _ _]
            tunnel: w844 -> [_ _ _ w858 _]
            tunnel: w843 -> [_ _ _ _ w859]
            frame 0, Default {
            }
            frame 1 {
            }
            frame 2 {
            }
            frame 3 {
            }
            frame 4 {
            }
          }
          n392 = call "File Wilt.vi"("Dryer Aisle In"=w852, "RW  Mode"=T11."Write Dryer Bank", "Dryer Bank Filename"=w851, "Aisle Label"=w853, "error in (no error)"=w850) -> ("error out"=w849:errorcluster)  [unwired: 7 in, 3 out]
        }
        n393 = flat-sequence {
          tunnel: w829 -> [_]
          frame #0 {
            n394 = local read "Debug"() -> (w836:bool)
            n395 = case shown="False" w836 {
              frame False {
                n396 = local write "User Notice"("" ("User Notice")) -> ()
              }
              frame True {
              }
            }
            n397 = local write "Save Setup"(FALSE ("Save Setup")) -> ()
          }
        }
        n398 = call <vilib>:"Add State(s) to Queue__jki_lib_state_machine.vi"("State(s) in (\"\")"=w835) -> ("States Out"=w834:string)  [unwired: 14 in]
      }
      frame "UI: Read State" {
        w878 = T11."Read Dryer Bank" ("RW  Mode")
        # "I re-did this section from a for loop to this.\nThis allowed me to remove the local variables"
        n399 = Unbundle By Name(w866) -> ("Dryer Bank Filename"=w876:path, "Remote Station"=w868:bool, "GUI Aisle 1"=w867:T1[], "GUI Aisle 1A"=w864:T1[], "GUI Aisle 2"=w863:T1[], "GUI Aisle 3"=w862:T1[], "GUI Aisle 4"=w861:T1[])
        n400 = call "File Wilt.vi"("Dryer Aisle In"=w867, "RW  Mode"=w878, "Dryer Bank Filename"=w876, "Aisle Label"="Aisle1", "error in (no error)"=w875) -> ("Dryer Aisle Out"=w865:T1[], "error out"=w874:errorcluster)  [unwired: 7 in, 2 out]
        n401 = case shown="False" w868 {
          tunnel: w878 -> [w902 _]
          tunnel: w876 -> [w897 _]
          tunnel: w875 -> [w896 w906]
          tunnel: [w895 w906] -> w873
          tunnel: [w894 w906] -> w872
          tunnel: [w893 w906] -> w871
          tunnel: [w892 w906] -> w870
          tunnel: w866 -> [w891 w905]
          tunnel: w865 -> [w890 w904]
          tunnel: [w889 w903] -> w860
          tunnel: w864 -> [w884 _]
          tunnel: w863 -> [w883 _]
          tunnel: w862 -> [w882 _]
          tunnel: w861 -> [w881 _]
          frame False {
            n402 = call "File Wilt.vi"("Dryer Aisle In"=w884, "RW  Mode"=w902, "Dryer Bank Filename"=w897, "Aisle Label"="Aisle1A", "error in (no error)"=w896) -> ("Dryer Aisle Out"=w888:T1[], "error out"=w895:errorcluster)  [unwired: 7 in, 2 out]
            n403 = call "File Wilt.vi"("Dryer Aisle In"=w883, "RW  Mode"=w902, "Dryer Bank Filename"=w897, "Aisle Label"="Aisle2", "error in (no error)"=w896) -> ("Dryer Aisle Out"=w887:T1[], "error out"=w894:errorcluster)  [unwired: 7 in, 2 out]
            n404 = call "File Wilt.vi"("Dryer Aisle In"=w882, "RW  Mode"=w902, "Dryer Bank Filename"=w897, "Aisle Label"="Aisle3", "error in (no error)"=w896) -> ("Dryer Aisle Out"=w886:T1[], "error out"=w893:errorcluster)  [unwired: 7 in, 2 out]
            n405 = call "File Wilt.vi"("Dryer Aisle In"=w881, "RW  Mode"=w902, "Dryer Bank Filename"=w897, "Aisle Label"="Aisle4", "error in (no error)"=w896) -> ("Dryer Aisle Out"=w885:T1[], "error out"=w892:errorcluster)  [unwired: 7 in, 2 out]
            n406 = Bundle By Name(cluster=w891, "GUI Aisle 1"=w890, "GUI Aisle 1A"=w888, "GUI Aisle 2"=w887, "GUI Aisle 3"=w886, "GUI Aisle 4"=w885) -> (w889:T16)
          }
          frame True {
            n407 = Bundle By Name(cluster=w905, "GUI Aisle 1"=w904) -> (w903:T16)
          }
        }
        n408 = call <vilib>:"Add State(s) to Queue__jki_lib_state_machine.vi"("State(s) in (\"\")"=w880) -> ("States Out"=w879:string)  [unwired: 14 in]
        n409 = Merge Errors(w874, w873, w872, w871, w870) -> (w869:errorcluster)
      }
      frame "UI: Cursor Set" {
        # "Argument"
        # "Set and Unset Cursor Busy.\n(Usage: \"UI: Cursor Set >> Busy|Idle\")"
        n410 = case shown="\"Idle\", Default" w907 {
          tunnel: w909 -> [w914 w916]
          tunnel: [w913 w915] -> w908
          frame "Idle", Default {
            n411 = call <vilib>:"Unset Busy.vi"("error in (no error)"=w914) -> ("error out"=w913:errorcluster)  [unwired: 10 in]
          }
          frame "Busy" {
            n412 = call <vilib>:"Set Busy.vi"("error in (no error)"=w916) -> ("error out"=w915:errorcluster)  [unwired: 9 in, 1 out]
          }
        }
        n413 = call <vilib>:"Add State(s) to Queue__jki_lib_state_machine.vi"("State(s) in (\"\")"=w912) -> ("States Out"=w911:string)  [unwired: 14 in]
      }
      frame "UI: Front Panel State" {
        # "Argument"
        # "Set Front Panel Open or Closed\n(Usage: \"UI: Front Panel State >> Open|Close\")"
        n414 = Unbundle By Name(w919) -> ("Core.Current VI Reference"=w918:refnum<vi>)
        n415 = case shown="\"Open\", Default" w917 {
          tunnel: w921 -> [w927 w944]
          tunnel: [w929 w945] -> w920
          tunnel: w918 -> [w928 w942]
          frame "Open", Default {
            n416 = property class="VI"(reference=w928, error in=w927) -> (reference out=w925:refnum<vi>, error out=w926:errorcluster, "Front Panel.Open"=w924:bool)
            n417 = case shown="True" w924 {
              tunnel: [w932 w938] -> w929
              tunnel: w926 -> [w931 w939]
              tunnel: w925 -> [w930 w937]
              frame False {
                n418 = invoke class="VI" method="FP.Open"(reference=w930, error in=w931, "Activate"=TRUE, "State"=T15."Maximized") -> (error out=w932:errorcluster)  [unwired: 1 in, 4 out]
              }
              frame True {
                n419 = invoke class="VI" method="FP.Open"(reference=w937, error in=w939, "Activate"=TRUE ("Activate?"), "State"=T15."Maximized") -> (error out=w938:errorcluster)  [unwired: 1 in, 4 out]
              }
            }
          }
          frame "Close" {
            n420 = property class="VI"(reference=w942, error in=w944) -> (reference out=w941:refnum<vi>, error out=w943:errorcluster, "Front Panel.Open"=w940:bool)
            n421 = case shown="True" w940 {
              tunnel: [w946 w949] -> w945
              tunnel: w943 -> [w946 w948]
              tunnel: w941 -> [_ w947]
              frame False {
              }
              frame True {
                n422 = invoke class="VI" method="FP.Close"(reference=w947, error in=w948) -> (error out=w949:errorcluster)  [unwired: 1 in, 2 out]
              }
            }
          }
        }
        n423 = call <vilib>:"Add State(s) to Queue__jki_lib_state_machine.vi"("State(s) in (\"\")"=w923) -> ("States Out"=w922:string)  [unwired: 14 in]
      }
      frame "---------- Macro ----------" {
        # "Do not put any code in this frame.\n(It is a separator no-op. You can make a copy of this frame to create a new Macro frame)"
        n424 = call <vilib>:"Add State(s) to Queue__jki_lib_state_machine.vi"("State(s) in (\"\")"=w953) -> ("States Out"=w952:string)  [unwired: 14 in]
      }
      frame "Macro: Initialize" {
        # "Initialization Macro\n(This is called once, when the VI starts)"
        n425 = call <vilib>:"Add State(s) to Queue__jki_lib_state_machine.vi"("State(s) in (\"\")"=w957) -> ("States Out"=w956:string)  [unwired: 14 in]
      }
      frame "Macro: Exit" {
        # "Exit Macro\n(This is called once, when the VI exits)"
        n426 = Unbundle By Name(w964) -> ("Core.Close Panel on Exit?"=w963:bool)
        n427 = Select(t="UI: Front Panel State >> Close", s=w963, f="") -> (s? t:f=w960:string)
        n428 = call <vilib>:"Add State(s) to Queue__jki_lib_state_machine.vi"("State(s) in (\"\")"=w960, "State(s) at Back (\"\")"="Data: Cleanup\nExit") -> ("States Out"=w958:string)  [unwired: 13 in]
        n429 = call <vilib>:"Add State(s) to Queue__jki_lib_state_machine.vi"("State(s) in Front (\"\")"=w958, "State(s) in (\"\")"=w967) -> ("States Out"=w966:string)  [unwired: 13 in]
      }
      frame "---------- Main ----------" {
        # "Start Datalogging and Start Test.  Datalogging continues on its own loop.\nUpdating the gui and saving data is a second loop.\n\nThe test will continue."
        # "Template Separator\n(You can make a copy of, or modify, this frame)"
        n430 = call <vilib>:"Add State(s) to Queue__jki_lib_state_machine.vi"("State(s) in (\"\")"=w971) -> ("States Out"=w970:string)  [unwired: 14 in]
      }
      frame "Start: DataLogging" {
        # "Your code here.\n(You can make a copy of, or modify, this frame)"
        n431 = flat-sequence {
          frame #0 {
            w976 = TRUE ("Init Complete")
            n432 = property on="Init Complete" class="Bool (strict)"("Val(Sgnl)"=w976) -> ()  [unwired: 2 in, 2 out]
            "Init Complete" <- w976
          }
        }
        n433 = call <vilib>:"Add State(s) to Queue__jki_lib_state_machine.vi"("State(s) in (\"\")"=w975) -> ("States Out"=w974:string)  [unwired: 14 in]
      }
      frame "-------Test----------" {
        # "Template Separator\n(You can make a copy of, or modify, this frame)"
        n434 = call <vilib>:"Add State(s) to Queue__jki_lib_state_machine.vi"("State(s) in (\"\")"=w980) -> ("States Out"=w979:string)  [unwired: 14 in]
      }
      frame "Start Test" {
        # "Delay 500 ms.  If \"Transition\"  reset, set all counts to 0.  Compile data into All Test Station Arry.  First time thru, close valves."
        n435 = Unbundle By Name(w985) -> ("USB6008"=w981:tag, "GUI Aisle 1"=w987:T1[], "GUI Aisle 1A"=w988:T1[], "GUI Aisle 2"=w989:T1[], "GUI Aisle 3"=w990:T1[], "GUI Aisle 4"=w991:T1[], "Agilent Channels Water Valves."=w986:T3[], "Remote Station"=w982:bool)
        n436 = Build Array (concatenate)(w987, w988, w989, w990, w991) -> (w983:T1[])
        "All Test Stations" <- w983
        n437 = Bundle By Name(cluster=w985, "All Test Stations Control"=w983) -> (w984:T16)
        n438 = stacked-sequence {
          tunnel: [FALSE ("Transition") _] -> w993
          tunnel: w985 -> [w1004 _]
          tunnel: w984 -> [w1002 _]
          tunnel: [w1001 _] -> w992
          tunnel: w983 -> [w1000 w1088]
          tunnel: w986 -> [_ w1087]
          tunnel: w982 -> [w998 w1086]
          tunnel: w981 -> [w999 w1085]
          frame #0 {
            n439 = event shown="[1] \"Transition\": Value Change" {
              selector: _ -> [_ _]
              dyn-events: _ -> [_ _]
              timeout: 500 ("milliseconds to wait") -> [_ _]
              tunnel: w1004 -> [w1008 w1017]
              tunnel: [w1007 w1016] -> w1003
              tunnel: w1000 -> [_ w1011]
              tunnel: w999 -> [_ w1010]
              tunnel: w998 -> [_ w1009]
              event Timeout {
                n440 = event-data() -> ()  [unwired: 1 in, 2 out]
                n441 = Unbundle By Name(w1008) -> ("Station Test State"=w1007:T8[])
              }
              event "Transition": Value Change {
                n442 = event-data() -> ()  [unwired: 1 in, 4 out]
                n443 = call <vilib>:"Three Button Dialog.vi"("Right Button Text (\"Cancel\")"="Night Shift" ("F button name (\"Cancel\")"), "Center Button Text (\"No\")"="Cancel" ("F button name (\"Cancel\")"), "Left Button Text (\"Yes\")"="Day Shift" ("T button name (\"OK\")"), "message"="Select Shift") -> ("Which Button?"=w1018:T18)  [unwired: 7 in]
                n444 = case shown="\"Right Button\"" w1018 {
                  tunnel: [TRUE ("x") _ TRUE ("x") _] -> w1012
                  frame "Left Button", Default {
                    w1079 = TRUE
                    n445 = local write "Day"(w1079) -> ()
                    n446 = property on="Day" class="Bool (strict)"("Val(Sgnl)"=w1079) -> ()  [unwired: 2 in, 2 out]
                    n447 = Not(x=w1079) -> (.not. x?=w1081:bool)
                    n448 = local write "Night"(w1081) -> ()
                  }
                  frame "Center Button" {
                  }
                  frame "Right Button" {
                    w1082 = FALSE ("x")
                    n449 = local write "Day"(w1082) -> ()
                    n450 = Not(x=w1082) -> (.not. x?=→"Night":bool)
                  }
                  frame "Window Close" {
                  }
                }
                n451 = case shown="True" w1012 {
                  tunnel: w1017 -> [w1021 w1028]
                  tunnel: w1011 -> [_ w1026]
                  tunnel: [w1020 w1025] -> w1016
                  tunnel: w1010 -> [_ w1023]
                  tunnel: w1009 -> [_ w1022]
                  frame False {
                    # "no transition"
                    n452 = Unbundle By Name(w1021) -> ("Station Test State"=w1020:T8[])
                  }
                  frame True {
                    n453 = Unbundle By Name(w1028) -> ("Station Test State"=w1027:T8[], "Agilent Channels Water Valves."=w1024:T3[])
                    n454 = for {
                      tunnel: w1027 -> [w1036] mode=indexing
                      tunnel: [w1035] -> w1025 mode=indexing
                      tunnel: w1026 -> [w1034] mode=indexing
                      tunnel: w1024 -> [w1032]
                      tunnel: w1023 -> [w1031]
                      tunnel: w1022 -> [w1030]
                      n455 = Unbundle By Name(w1034) -> ("Station Index"=w1033:i32, "Dryer Details.Run w/o Newfi"=w1029:i32)
                      n456 = case shown="1" w1029 {
                        tunnel: w1036 -> [w1042 w1068]
                        tunnel: [w1041 w1069] -> w1035
                        tunnel: w1033 -> [w1040 _]
                        tunnel: w1032 -> [w1039 _]
                        tunnel: w1031 -> [w1038 _]
                        tunnel: w1030 -> [w1037 w1067]
                        frame 0, Default {
                          n457 = case shown="\"Watering\"" w1042 {
                            selector: w1042 -> [w1043 w1044 _ _ _ _ _ _ w1066]
                            tunnel: [w1043 w1044 Dryer_Test_State."Wait Com" ("Test State") Dryer_Test_State."Wait Com" ("Test State") Dryer_Test_State."Wait Com" ("Test State") Dryer_Test_State."Wait Com" ("Test State") Dryer_Test_State."Wait Com" ("Test State") Dryer_Test_State."Wait Com" ("Test State") w1066] -> w1041
                            tunnel: w1040 -> [_ _ _ w1051 _ _ _ _ _]
                            tunnel: w1039 -> [_ _ _ w1048 _ _ _ _ _]
                            tunnel: w1038 -> [_ _ _ w1047 _ _ _ _ _]
                            tunnel: w1037 -> [_ _ _ w1046 _ _ _ _ _]
                            frame "No SN", Default {
                            }
                            frame "Wait Com" {
                            }
                            frame "Wait to Start" {
                            }
                            frame "Watering" {
                              n458 = case shown="False" w1046 {
                                tunnel: w1051 -> [w1056 w1061]
                                tunnel: [w1053 _] -> w1049
                                tunnel: w1048 -> [w1052 _]
                                tunnel: w1047 -> [_ w1058]
                                frame False {
                                # "Turn off valve"
                                n459 = Number To Decimal String(number=w1056) -> (decimal integer string=w1055:string)  [unwired: 1 in]
                                n460 = local read "Agilent"() -> (w1054:T9)
                                n461 = call "Agilent Valve Control.vi"("Station In"=w1055, "Agilent Channels In"=w1052, "Agilent"=w1054, "Open/Close (F:Close)"=TRUE) -> ("error out"=w1053:errorcluster)  [unwired: 9 in, 2 out]
                                }
                                frame True {
                                # "Turn off valve"
                                n462 = To Long Integer(number=w1061) -> (32bit integer=w1060:i32)
                                n463 = call "Valve Control Single 6008.vi"("Valve On?"=FALSE, "Valve Number"=w1060, "Port"=w1058) -> ()  [unwired: 8 in, 1 out]
                                }
                              }
                              "valve error out" <- w1049
                            }
                            frame "Drying" {
                            }
                            frame "Cooldown" {
                            }
                            frame "Paused" {
                            }
                            frame "Temp Fault" {
                            }
                            frame "Com Fault" {
                            }
                          }
                        }
                        frame 1 {
                          n464 = case shown="\"Paused\"" w1068 {
                            selector: w1068 -> [w1070 w1071 w1072 w1073 w1074 w1075 w1076 w1077 w1078]
                            tunnel: [w1070 w1071 w1072 w1073 w1074 w1075 w1076 w1077 w1078] -> w1069
                            tunnel: w1067 -> [_ _ _ _ _ _ _ _ _]
                            frame "No SN", Default {
                            }
                            frame "Wait Com" {
                            }
                            frame "Wait to Start" {
                            }
                            frame "Watering" {
                            }
                            frame "Drying" {
                            }
                            frame "Cooldown" {
                            }
                            frame "Paused" {
                            }
                            frame "Temp Fault" {
                            }
                            frame "Com Fault" {
                            }
                          }
                        }
                      }
                    }
                  }
                }
              }
            }
            n465 = Bundle By Name(cluster=w1002, "Station Test State"=w1003) -> (w1001:T16)
          }
          frame #1 {
            n466 = call "Counter.vi"() -> ("Count"=w1091:dbl)  [unwired: 11 in]
            "Main Loop Count" <- w1091
            n467 = Equal?(x=w1091, y=1.0) -> (x = y?=w1089:bool)
            n468 = case shown="True" w1089 {
              tunnel: w1088 -> [_ w1097]
              tunnel: w1087 -> [_ w1095]
              tunnel: w1086 -> [_ w1094]
              tunnel: w1085 -> [_ w1093]
              frame False {
              }
              frame True {
                n469 = for {
                  tunnel: w1097 -> [w1103] mode=indexing
                  tunnel: w1095 -> [w1101]
                  tunnel: w1094 -> [w1100]
                  tunnel: w1093 -> [w1099]
                  tunnel: [w1098] -> w1092 mode=indexing
                  # "Turn off valve"
                  n470 = Unbundle By Name(w1103) -> ("Station Index"=w1102:i32)
                  n471 = case shown="False" w1100 {
                    tunnel: w1101 -> [w1107 _]
                    tunnel: w1102 -> [w1104 w1112]
                    tunnel: w1099 -> [_ w1111]
                    tunnel: [w1105 "USB6009"] -> w1098
                    frame False {
                      n472 = local read "Agilent"() -> (w1106:T9)
                      n473 = Number To Decimal String(number=w1104) -> (decimal integer string=w1109:string)  [unwired: 1 in]
                      n474 = call "Agilent Valve Control.vi"("Station In"=w1109, "Agilent Channels In"=w1107, "Agilent"=w1106, "Open/Close (F:Close)"=TRUE) -> ("Channel State?"=w1105:string)  [unwired: 9 in, 2 out]
                    }
                    frame True {
                      n475 = To Long Integer(number=w1112) -> (32bit integer=w1114:i32)
                      n476 = call "Valve Control Single 6008.vi"("Valve On?"=FALSE, "Valve Number"=w1114, "Port"=w1111) -> ()  [unwired: 8 in, 1 out]
                    }
                  }
                }
                "Valve States" <- w1092
                n477 = local write "User Notice"("Test Running." ("User Notice")) -> ()
              }
            }
          }
        }
        n478 = call <vilib>:"Add State(s) to Queue__jki_lib_state_machine.vi"("State(s) in Front (\"\")"="No SN\nWait Com\nWait to Start\nWatering\nPause Manual Stations\nDrying\nCooldown\nContinue\nUpdate From DAQ Loop\nEmergency Shutoff\nCheck E-Timer" ("State(s) in Front (\"\")"), "State(s) in (\"\")"=w997) -> ("States Out"=w996:string)  [unwired: 13 in]
        n479 = local write "Transition"(w993) -> ()
      }
      frame "No SN" {
        # "Ifserial number is changed from \"\" to something, then state goes to Wait Com.  This implies that\nthe user should change the serial number before installing a new dryer."
        n480 = Unbundle By Name(w1122) -> ("Station Test State"=w1118:T8[], "All Test Stations Control"=w1116:T1[], "Emergency Timer"=w1115:i32[])
        n481 = local write "Station Test State"(w1118) -> ()
        n482 = for {
          tunnel: w1116 -> [w1127] mode=indexing
          tunnel: [w1131] -> w1120 mode=indexing
          tunnel: w1118 -> [w1130] mode=indexing
          tunnel: Dryer_Test_State."Com Fault" ("Test State") -> [w1129]
          tunnel: w1115 -> [w1126] mode=indexing
          n483 = Greater Than 0?(x=w1126) -> (x > 0?=w1125:bool)
          n484 = Not Equal?(x=w1130, y=w1129) -> (x != y?=w1128:bool)
          n485 = case shown="False" w1125 {
            tunnel: w1127 -> [w1135 _]
            tunnel: [w1134 w1147] -> w1131
            tunnel: w1130 -> [w1133 w1147]
            tunnel: w1128 -> [w1132 _]
            frame False {
              n486 = case shown="True" w1132 {
                tunnel: w1135 -> [_ w1146]
                tunnel: [w1136 w1139] -> w1134
                tunnel: w1133 -> [w1136 w1138]
                frame False {
                }
                frame True {
                  n487 = Unbundle By Name(w1146) -> ("Lab ID"=w1145:string)
                  n488 = Equal?(x=w1138, y=Dryer_Test_State."No SN" ("Test State")) -> (x = y?=w1142:bool)
                  n489 = Not Equal?(x=w1145, y="") -> (x != y?=w1141:bool)
                  n490 = And(x=w1141, y=w1142) -> (x .and. y?=w1140:bool)
                  n491 = Select(t=Dryer_Test_State."Wait Com" ("Test State"), s=w1140, f=w1138) -> (s? t:f=w1139:T8)
                }
              }
            }
            frame True {
            }
          }
        }
        n492 = Bundle By Name(cluster=w1122, "Station Test State"=w1120) -> (w1121:T16)
        n493 = call <vilib>:"Add State(s) to Queue__jki_lib_state_machine.vi"("State(s) in (\"\")"=w1124) -> ("States Out"=w1123:string)  [unwired: 14 in]
      }
      frame "Wait Com" {
        # "If in wait com, if the elapsed time is > wait com timer, then send out the wilt startup commands.\nTransition when the status is not Err to wait to start."
        n494 = Unbundle By Name(w1159) -> ("All Confgured Com Array"=w1149:u8[], "Station Timer"=w1152:dbl[], "Station Test State"=w1154:T8[], "Station Com List"=w1156:u8[], "Emergency Timer"=w1148:i32[])
        n495 = call "E-Time.vi"() -> ("Elapsed Time (sec)"=w1166:dbl)  [unwired: 9 in, 2 out]
        n496 = local write "Station Timer"(w1152) -> ()
        n497 = Subtract(x=w1166, y=w1152) -> (x-y=w1165:dbl[])
        n498 = local write "Station Test State"(w1154) -> ()
        n499 = Subtract(x=w1165, y="Wait Com Timer") -> (x-y=w1163:dbl[])
        n500 = local read "Dryer Com Info"() -> (w1151:T5[])
        n501 = Greater Than 0?(x=w1163) -> (x > 0?=w1162:bool[])
        n502 = Equal?(x=w1154, y=Dryer_Test_State."Wait Com" ("Test State")) -> (x = y?=w1150:bool[])
        n503 = And(x=w1162, y=w1150) -> (x .and. y?=w1161:bool[])
        n504 = for {
          tunnel: w1161 -> [w1191]
          tunnel: w1149 -> [w1189] mode=indexing
          tunnel: w1156 -> [w1190]
          shift-right: [w1184] -> w1153
          shift-left: w1154 -> [w1185]
          tunnel: w1151 -> [w1183] mode=indexing
          shift-right: [w1182] -> _
          shift-left: _ -> [w1181]
          shift-right: [w1188] -> w1160
          shift-left: w1152 -> [w1187]
          shift-right: [w1186] -> w1155
          shift-left: w1168 -> [w1192]
          tunnel: w1148 -> [w1180] mode=indexing
          n505 = Greater Than 0?(x=w1180) -> (x > 0?=w1179:bool)
          n506 = case shown="False" w1179 {
            tunnel: w1192 -> [w1210 w1251]
            tunnel: w1191 -> [w1209 _]
            tunnel: w1190 -> [w1206 _]
            tunnel: w1189 -> [w1205 _]
            tunnel: [w1204 w1252] -> w1188
            tunnel: w1187 -> [w1203 w1252]
            tunnel: [w1200 w1251] -> w1186
            tunnel: w1185 -> [w1199 w1249]
            tunnel: [w1197 w1249] -> w1184
            tunnel: w1183 -> [w1196 _]
            tunnel: [w1194 w1250] -> w1182
            tunnel: w1181 -> [w1193 w1250]
            frame False {
              n507 = Search 1D Array(1D array=w1206, element=w1205) -> (index of element=w1198:i32)  [unwired: 1 in]
              n508 = Index Array(array=w1209, index=w1198) -> (element=w1207:bool)
              n509 = Index Array(array=w1203, index=w1198) -> (element=w1208:dbl)
              n510 = case shown="True" w1207 {
                tunnel: w1210 -> [w1223 w1242]
                tunnel: [w1223 w1234] -> w1201
                tunnel: [_ w1226] -> w1195
                tunnel: [w1222 w1240] -> w1202
                tunnel: w1208 -> [w1222 _]
                tunnel: w1205 -> [_ w1239]
                tunnel: [w1221 w1237] -> w1197
                tunnel: w1199 -> [w1221 w1238]
                tunnel: w1198 -> [_ w1236]
                tunnel: w1196 -> [_ w1231]
                tunnel: [w1220 w1227] -> w1194
                tunnel: w1193 -> [w1220 w1224]
                frame False {
                }
                frame True {
                  # "Wait for com station test state."
                  n511 = Unbundle By Name(w1231) -> ("Last Read Status"=w1230:T6)
                  n512 = local read "Gathering Data Latch"() -> (w1232:bool)
                  n513 = Not Equal?(x=w1230, y=Dryer_Status_Ctrl."Err" ("Last Read Status")) -> (x != y?=w1228:bool)
                  n514 = And(x=w1228, y=w1232) -> (x .and. y?=w1233:bool)
                  n515 = local read "Debug"() -> (w1225:bool)
                  n516 = case shown="True" w1233 {
                    tunnel: [Dryer_Test_State."Wait Com" ("Test State") Dryer_Test_State."Wait to Start" ("Test State")] -> w1235
                    frame False {
                    }
                    frame True {
                    }
                  }
                  n517 = call "Com Chan Type Conversion.vi"("Com Chan"=w1239) -> ("VISA resource name"=w1226:refnum<visa-resource-name>)  [unwired: 11 in, 3 out]
                  n518 = call "GEA2_ICP_Dryer_SM.vi"("ComPort"=w1226, "Mode"=GEA2_Dryer_Interface_Ctrl."Send WILT Startup CMDs", "Error In"=w1242) -> ("Error Out"=w1234:errorcluster)  [unwired: 7 in, 5 out]
                  n519 = case shown="False" w1225 {
                    tunnel: w1226 -> [_ w1246]
                    tunnel: [w1243 w1245] -> w1227
                    tunnel: w1224 -> [w1243 w1244]
                    frame False {
                    }
                    frame True {
                      n520 = Build Array (concatenate)(w1244, w1246) -> (w1245:refnum<visa-resource-name>[])
                      "Startup Coms" <- w1245
                    }
                  }
                  n521 = call "E-Time.vi"() -> ("Elapsed Time (sec)"=w1240:dbl)  [unwired: 9 in, 2 out]
                  n522 = Replace Array Subset(array=w1238, new element=w1235, index=w1236) -> (w1237:T8[])
                }
              }
              n523 = Replace Array Subset(array=w1203, new element=w1202, index=w1198) -> (w1204:dbl[])
              n524 = case shown="Error" w1201 {
                selector: w1201 -> [w1212 w1214]
                tunnel: w1195 -> [_ w1217]
                tunnel: [w1212 w1216] -> w1200
                frame No Error {
                  n525 = local write "User Notice"("No Com Error" ("User Notice")) -> ()
                }
                frame Error {
                  w1219 = "Wait COM Error.   "
                  n526 = Unbundle By Name(w1214) -> ("source"=w1213:string)
                  n527 = Type Cast(type=w1219, x=w1217) -> (*(type *) &x=w1218:string)
                  n528 = Concatenate Strings(w1219, w1218, w1213) -> (w1215:string)
                  n529 = local write "User Notice"(w1215) -> ()
                  n530 = call <vilib>:"Clear Errors.vi"("error in (no error)"=w1214) -> ("error out"=w1216:errorcluster)  [unwired: 6 in]
                }
              }
            }
            frame True {
              # "If the user or program sets stop dryer command. This will allows the dryer to continue\ndrying but will not start the next cycle"
            }
          }
        }
        n531 = stacked-sequence {
          tunnel: [w1172] -> w1157
          tunnel: w1155 -> [_]
          frame #0 {
            n532 = local read "Save Setup"() -> (w1171:bool)
            n533 = local read "Stop Test"() -> (w1173:bool)
            n534 = case shown="False" w1173 {
              tunnel: [w1175 "UI: Save Current State\nExit" ("State(s) in Front (\"\")")] -> w1172
              tunnel: w1171 -> [w1174 _]
              frame False {
                n535 = case shown="False" w1174 {
                  tunnel: ["Check Wait" ("State(s) in Front (\"\")") "UI: Save Current State\nCheck Wait" ("State(s) in Front (\"\")")] -> w1175
                  frame False {
                  }
                  frame True {
                  }
                }
              }
              frame True {
              }
            }
          }
        }
        n536 = Bundle By Name(cluster=w1159, "Station Timer"=w1160, "Station Test State"=w1153) -> (w1158:T16)
        n537 = call <vilib>:"Add State(s) to Queue__jki_lib_state_machine.vi"("State(s) in Front (\"\")"=w1157, "State(s) in (\"\")"=w1170) -> ("States Out"=w1169:string)  [unwired: 13 in]
      }
      frame "Check Wait" {
        # "Wait for both status and log to be reported."
        n538 = Unbundle By Name(w1261) -> ("Station Test State"=w1254:T8[], "Station Timer"=w1256:dbl[], "All Test Stations Control"=w1253:T1[])
        n539 = local write "Station Test State"(w1254) -> ()
        n540 = Equal?(x=w1254, y=Dryer_Test_State."Wait to Start" ("Test State")) -> (x = y?=w1258:bool[])
        n541 = disable-structure shown="Enabled" {
          disable-tunnel: w1258 -> [w1270 _]
          disable-tunnel: w1253 -> [w1269 _]
          disable-tunnel: [w1268 w1298] -> w1257
          disable-tunnel: w1256 -> [w1267 w1297]
          disable-tunnel: [w1266 w1297] -> w1255
          disable-tunnel: w1254 -> [w1265 w1298]
          frame Disabled {
            # "The check is that both string lengths are > 0. Assumes that these are initializied to \"\".\nReset the timer value to the current time once you wait to start."
            n542 = for {
              tunnel: w1270 -> [w1276] mode=indexing
              tunnel: w1269 -> [w1275] mode=indexing
              tunnel: [w1274] -> w1268 mode=indexing
              tunnel: w1265 -> [w1273] mode=indexing
              tunnel: w1267 -> [w1272] mode=indexing
              tunnel: [w1271] -> w1266 mode=indexing
              i -> [w1277]
              n543 = case shown="True" w1276 {
                tunnel: w1277 -> [_ _]
                tunnel: w1275 -> [_ w1294]
                tunnel: [w1279 w1285] -> w1274
                tunnel: w1273 -> [w1279 _]
                tunnel: w1272 -> [w1278 w1282]
                tunnel: [w1278 w1284] -> w1271
                frame False {
                }
                frame True {
                  n544 = Unbundle By Name(w1294) -> ("Sample Record"=w1293:string[])
                  n545 = Index Array(array=w1293, index #1=3 ("disabled index (col)"), index #2=4 ("disabled index (col)")) -> (element #1=w1292:string, element #2=w1291:string)
                  n546 = String Length(string=w1292) -> (length=w1290:i32)
                  n547 = String Length(string=w1291) -> (length=w1289:i32)
                  n548 = Multiply(x=w1290, y=w1289) -> (x*y=w1288:i32)
                  n549 = Not Equal To 0?(x=w1288) -> (x != 0?=w1283:bool)
                  n550 = Select(t=Dryer_Test_State."Wait to Start" ("Test State"), s=w1283, f=Dryer_Test_State."Wait Com" ("Test State")) -> (s? t:f=w1285:T8)
                  n551 = case shown="True" w1283 {
                    tunnel: [w1295 w1296] -> w1284
                    tunnel: w1282 -> [w1295 _]
                    frame False {
                    }
                    frame True {
                      n552 = call "E-Time.vi"() -> ("Elapsed Time (sec)"=w1296:dbl)  [unwired: 9 in, 2 out]
                    }
                  }
                }
              }
            }
          }
          frame Enabled {
            # "Not sure why this is here, to verify the output of wait com.\nThis depends on the periodic output of the serial port.  It is not \nlike this in the  first real dryer."
          }
        }
        n553 = call <vilib>:"Add State(s) to Queue__jki_lib_state_machine.vi"("State(s) in (\"\")"=w1264) -> ("States Out"=w1263:string)  [unwired: 14 in]
        n554 = Bundle By Name(cluster=w1261, "Station Test State"=w1257, "Station Timer"=w1255) -> (w1260:T16)
      }
      frame "Check for Fault" {
        # "If the color is indicating fault, set test state to fault.  Reset will reset back to Wait Com.\nA notice will be sent to user notice block in the case of a fault."
        n555 = Unbundle By Name(w1304) -> ("All Test Stations Control"=w1300:T1[], "Station Test State"=w1301:T8[], "Emergency Timer"=w1299:i32[])
        n556 = Equal?(x=w1301, y=Dryer_Test_State."Temp Fault" ("Test State")) -> (x = y?=w1306:bool[])
        n557 = local write "Station Test State"(w1301) -> ()
        n558 = for {
          tunnel: w1306 -> [w1321] mode=indexing
          tunnel: w1300 -> [w1316] mode=indexing
          tunnel: [w1320] -> w1305 mode=indexing
          tunnel: w1301 -> [w1319] mode=indexing
          tunnel: [w1318] -> w1303
          tunnel: "Reset Faults" -> [w1317]
          tunnel: w1299 -> [w1315] mode=indexing
          n559 = Greater Than 0?(x=w1315) -> (x > 0?=w1314:bool)
          n560 = case shown="False" w1314 {
            tunnel: w1321 -> [w1327 _]
            tunnel: [w1326 w1346] -> w1320
            tunnel: w1319 -> [w1325 w1346]
            tunnel: [w1324 w1347] -> w1318
            tunnel: w1317 -> [w1323 w1347]
            tunnel: w1316 -> [w1322 _]
            frame False {
              n561 = case shown="True" w1327 {
                tunnel: w1322 -> [w1337 _]
                tunnel: [w1334 w1343] -> w1326
                tunnel: w1325 -> [_ w1342]
                tunnel: [w1331 w1341] -> w1324
                tunnel: w1323 -> [w1331 w1341]
                frame False {
                  n562 = Unbundle By Name(w1337) -> ("Station Index"=w1330:i32, "Status Color"=w1333:u32)
                  n563 = global read "Globals Wilt.vi" "Fault Color"() -> (w1332:u32)
                  n564 = Equal?(x=w1333, y=w1332) -> (x = y?=w1329:bool)
                  n565 = Number To Decimal String(number=w1330) -> (decimal integer string=w1328:string)  [unwired: 1 in]
                  n566 = Select(t=Dryer_Test_State."Temp Fault" ("Test State"), s=w1329, f=Dryer_Test_State."Wait Com" ("Test State")) -> (s? t:f=w1334:T8)
                  n567 = case shown="True" w1329 {
                    tunnel: w1328 -> [_ w1338]
                    frame False {
                    }
                    frame True {
                      n568 = Concatenate Strings("Temp Fault Station " ("string"), w1338) -> (w1340:string)
                      n569 = local write "User Notice"(w1340) -> ()
                    }
                  }
                }
                frame True {
                  n570 = case shown="True" w1341 {
                    tunnel: [w1344 Dryer_Test_State."Wait Com" ("Test State")] -> w1343
                    tunnel: w1342 -> [w1344 _]
                    frame False {
                    }
                    frame True {
                    }
                  }
                }
              }
            }
            frame True {
              # "If the user or program sets stop dryer command. This will allows the dryer to continue drying but will not start the next cycle"
            }
          }
        }
        n571 = case shown="True" w1303 {
          frame False {
          }
          frame True {
            n572 = local write "Reset Faults"(FALSE ("Reset Faults")) -> ()
            n573 = local write "User Notice"("" ("User Notice")) -> ()
          }
        }
        n574 = Bundle By Name(cluster=w1304, "Station Test State"=w1305) -> (w1308:T16)
        n575 = call <vilib>:"Add State(s) to Queue__jki_lib_state_machine.vi"("State(s) in (\"\")"=w1311) -> ("States Out"=w1310:string)  [unwired: 14 in]
      }
      frame "Wait to Start" {
        # "Transition to Watering if the dryer status is cycle running.\nTransition to Wait Com if elapsed time > Resend Start Limit"
        n576 = Unbundle By Name(w1358) -> ("Station Test State"=w1353:T8[], "Station Timer"=w1354:dbl[], "Pause Timer"=w1350:i32[], "All Test Stations Control"=w1349:T1[], "Emergency Timer"=w1348:i32[])
        n577 = Equal?(x=Dryer_Test_State."Wait to Start" ("Test State"), y=w1353) -> (x = y?=w1360:bool[])
        n578 = local write "Station Test State"(w1353) -> ()
        n579 = for {
          tunnel: w1360 -> [w1372] mode=indexing
          tunnel: w1349 -> [w1365] mode=indexing
          tunnel: [w1371] -> w1356 mode=indexing
          tunnel: w1353 -> [w1370] mode=indexing
          tunnel: w1354 -> [w1369] mode=indexing
          tunnel: [w1368] -> w1352 mode=indexing
          tunnel: [w1367] -> w1351 mode=indexing
          tunnel: w1350 -> [w1366] mode=indexing
          tunnel: w1348 -> [w1364] mode=indexing
          n580 = Greater Than 0?(x=w1364) -> (x > 0?=w1363:bool)
          n581 = case shown="False" w1363 {
            tunnel: w1372 -> [w1380 _]
            tunnel: [w1379 w1414] -> w1371
            tunnel: w1370 -> [w1378 w1414]
            tunnel: w1369 -> [w1377 w1416]
            tunnel: [w1376 w1416] -> w1368
            tunnel: [w1375 w1415] -> w1367
            tunnel: w1366 -> [w1374 w1415]
            tunnel: w1365 -> [w1373 _]
            frame False {
              n582 = case shown="True" w1380 {
                tunnel: w1373 -> [_ w1398]
                tunnel: [w1383 w1389] -> w1379
                tunnel: w1378 -> [w1383 _]
                tunnel: w1377 -> [w1382 w1386]
                tunnel: [w1382 w1388] -> w1376
                tunnel: [w1381 w1385] -> w1375
                tunnel: w1374 -> [w1381 w1384]
                frame False {
                }
                frame True {
                  n583 = call "E-Time.vi"() -> ("Elapsed Time (sec)"=w1394:dbl)  [unwired: 9 in, 2 out]
                  n584 = Subtract(x=w1394, y=w1386) -> (x-y=w1393:dbl)
                  n585 = Unbundle By Name(w1398) -> ("Dryer Details.Status"=w1395:string)
                  n586 = Subtract(x=w1393, y="Resend Start Limit") -> (x-y=w1391:dbl)
                  n587 = call "Type Conv - Dryer Status to Txt.vi"("Status"=Dryer_Status_Ctrl."Cycle Running") -> ("Ring Text.Text"=w1396:string)  [unwired: 10 in]
                  n588 = Greater Than 0?(x=w1391) -> (x > 0?=w1387:bool)
                  n589 = Equal?(x=w1395, y=w1396) -> (x = y?=w1390:bool)
                  n590 = case shown="False" w1390 {
                    tunnel: [w1403 Dryer_Test_State."Watering" ("Test State")] -> w1389
                    tunnel: [w1402 0.0 ("element")] -> w1388
                    tunnel: w1387 -> [w1404 _]
                    tunnel: w1386 -> [w1401 _]
                    tunnel: [w1399 0 ("element")] -> w1385
                    tunnel: w1384 -> [w1400 _]
                    frame False {
                      n591 = case shown="True" w1404 {
                        tunnel: [Dryer_Test_State."Wait to Start" ("Test State") Dryer_Test_State."Wait Com" ("Test State")] -> w1403
                        tunnel: [w1406 w1410] -> w1402
                        tunnel: w1401 -> [w1406 w1410]
                        tunnel: w1400 -> [w1405 w1408]
                        tunnel: [w1405 w1408] -> w1399
                        frame False {
                          # "Wait"
                        }
                        frame True {
                          # "Resend Command"
                        }
                      }
                    }
                    frame True {
                      # "Continue.  Having a timer\nvalue of 0 is trigger to turn on valve"
                    }
                  }
                }
              }
            }
            frame True {
              # "If the user or program sets stop dryer command. This will allows the dryer to continue\ndrying but will not start the next cycle"
            }
          }
        }
        n592 = Bundle By Name(cluster=w1358, "Station Test State"=w1356, "Station Timer"=w1352, "Pause Timer"=w1351) -> (w1357:T16)
        n593 = call <vilib>:"Add State(s) to Queue__jki_lib_state_machine.vi"("State(s) in (\"\")"=w1362) -> ("States Out"=w1361:string)  [unwired: 14 in]
      }
      frame "Watering" {
        n594 = Unbundle By Name(w1435) -> ("Emergency Timer"=w1417:i32[], "USB6008"=w1418:tag, "Remote Station"=w1419:bool, "All Test Stations Control"=w1420:T1[], "Station Test State"=w1427:T8[], "Station Timer"=w1431:dbl[], "Agilent Channels Water Valves."=w1421:T3[])
        n595 = local write "Station Test State"(w1427) -> ()
        n596 = Build Array (concatenate)("Aisle 1 (1-20)", "Aisle 2 (21-32)", "Aisle 3 (33-44)", "Aisle 4 (45-56)") -> (w1422:dbl[])
        n597 = Equal?(x=Dryer_Test_State."Watering" ("Test State"), y=w1427) -> (x = y?=w1436:bool[])
        n598 = for {
          tunnel: w1436 -> [w1452] mode=indexing
          tunnel: w1420 -> [w1441] mode=indexing
          tunnel: [w1451] -> w1433 mode=indexing
          tunnel: w1427 -> [w1450] mode=indexing
          tunnel: w1431 -> [w1449] mode=indexing
          tunnel: [w1448] -> w1430 mode=indexing
          tunnel: w1429 -> [w1447]
          tunnel: [w1446] -> w1428
          tunnel: w1422 -> [w1445] mode=indexing
          tunnel: w1418 -> [w1444]
          tunnel: w1421 -> [w1443]
          tunnel: w1419 -> [w1442]
          tunnel: w1417 -> [w1439] mode=indexing
          n599 = Greater Than 0?(x=w1439) -> (x > 0?=w1440:bool)
          n600 = case shown="False" w1440 {
            tunnel: w1452 -> [w1464 _]
            tunnel: [w1463 w1626] -> w1451
            tunnel: w1450 -> [w1462 w1626]
            tunnel: w1449 -> [w1461 w1625]
            tunnel: [w1460 w1625] -> w1448
            tunnel: w1447 -> [w1459 w1624]
            tunnel: [w1458 w1624] -> w1446
            tunnel: w1445 -> [w1457 _]
            tunnel: w1444 -> [w1456 _]
            tunnel: w1443 -> [w1455 _]
            tunnel: w1442 -> [w1454 _]
            tunnel: w1441 -> [w1453 _]
            frame False {
              # "Cycle thru stations"
              n601 = case shown="True" w1464 {
                tunnel: w1453 -> [_ w1471]
                tunnel: [w1467 w1482] -> w1463
                tunnel: w1462 -> [w1467 w1470]
                tunnel: w1461 -> [w1466 w1485]
                tunnel: [w1466 w1486] -> w1460
                tunnel: w1459 -> [w1465 w1484]
                tunnel: [w1465 w1483] -> w1458
                tunnel: w1457 -> [_ w1481]
                tunnel: w1456 -> [_ w1477]
                tunnel: w1455 -> [_ w1472]
                tunnel: w1454 -> [_ w1469]
                frame False {
                  # "station not watering, skip to next station state"
                }
                frame True {
                  # "Station Watering"
                  n602 = Unbundle By Name(w1471) -> ("Com Port"=w1474:u8, "Station Index"=w1480:i32, "Station Label"=w1475:string, "Cycle Index"=w1476:string, "Dryer Details.Run w/o Newfi"=w1473:i32, "Dryer Details.24 Hour Water Injection"=w1468:i32)
                  n603 = local read "Agilent"() -> (w1479:T9)
                  n604 = Equal To 0?(x=w1485) -> (x = 0?=w1487:bool)
                  n605 = case shown="False" w1487 {
                    tunnel: w1480 -> [w1502 w1587]
                    tunnel: [w1494 w1586] -> w1486
                    tunnel: w1485 -> [w1494 _]
                    tunnel: w1484 -> [w1509 w1579]
                    tunnel: [w1509 w1580] -> w1483
                    tunnel: [w1504 w1573] -> w1482
                    tunnel: w1481 -> [w1495 _]
                    tunnel: w1472 -> [w1503 w1585]
                    tunnel: w1479 -> [w1501 w1584]
                    tunnel: [w1500 w1580] -> w1478
                    tunnel: w1469 -> [w1499 w1582]
                    tunnel: w1477 -> [w1498 w1581]
                    tunnel: w1476 -> [w1497 w1577]
                    tunnel: w1474 -> [_ w1574]
                    tunnel: w1473 -> [w1496 w1571]
                    tunnel: w1470 -> [w1493 _]
                    tunnel: w1468 -> [w1492 w1570]
                    frame False {
                      # "watering.  wait for time to expire.  check cycle index and stop if wrong."
                      # "keep going till time out"
                      n606 = call "E-Time.vi"() -> ("Elapsed Time (sec)"=w1508:dbl)  [unwired: 9 in, 2 out]
                      n607 = Subtract(x=w1508, y=w1494) -> (x-y=w1507:dbl)
                      n608 = Subtract(x=w1507, y=w1495) -> (x-y=w1506:dbl)
                      n609 = Greater Than 0?(x=w1506) -> (x > 0?=w1505:bool)
                      n610 = case shown="True" w1505 {
                        tunnel: [w1520 w1556] -> w1504
                        tunnel: w1503 -> [w1516 w1555]
                        tunnel: w1502 -> [w1514 w1554]
                        tunnel: w1501 -> [w1515 w1553]
                        tunnel: [errorcluster {"status"=FALSE, "code"=0, "source"=""} ("error out") w1552] -> w1500
                        tunnel: w1499 -> [w1512 w1551]
                        tunnel: w1498 -> [w1513 w1550]
                        tunnel: w1497 -> [w1518 _]
                        tunnel: w1496 -> [w1510 w1549]
                        tunnel: w1493 -> [_ w1548]
                        tunnel: w1492 -> [w1511 _]
                        frame False {
                          n611 = case shown="1" w1510 {
                            tunnel: w1518 -> [w1523 _]
                            tunnel: [w1522 w1525] -> w1517
                            tunnel: w1511 -> [_ w1524]
                            frame 0, Default {
                              n612 = local read "Day"() -> (w1521:bool)
                              n613 = call "Check Cycle Index.vi"("Day"=w1521, "Cycle Index"=w1523) -> ("Correct Cycle"=w1522:bool)  [unwired: 8 in, 1 out]
                            }
                            frame 1 {
                              n614 = case shown="1" w1524 {
                                tunnel: [w1526 TRUE ("Day")] -> w1525
                                frame 0, Default {
                                n615 = local read "Day"() -> (w1526:bool)
                                }
                                frame 1 {
                                }
                              }
                            }
                          }
                          n616 = case shown="True" w1517 {
                            tunnel: [w1534 Dryer_Test_State."Watering" ("Test State")] -> w1520
                            tunnel: w1516 -> [w1533 _]
                            tunnel: w1515 -> [w1532 _]
                            tunnel: w1514 -> [w1531 _]
                            tunnel: w1513 -> [w1530 _]
                            tunnel: w1512 -> [w1529 _]
                            tunnel: w1510 -> [w1528 _]
                            frame False {
                              # "wrong cycle.  stop vavle"
                              n617 = case shown="False" w1529 {
                                tunnel: w1533 -> [w1542 _]
                                tunnel: w1531 -> [w1540 w1545]
                                tunnel: w1532 -> [w1539 _]
                                tunnel: [w1538 _] -> _
                                tunnel: w1530 -> [_ w1546]
                                frame False {
                                n618 = Number To Decimal String(number=w1540) -> (decimal integer string=w1537:string)  [unwired: 1 in]
                                n619 = call "Agilent Valve Control.vi"("Station In"=w1537, "Agilent Channels In"=w1542, "Agilent"=w1539, "Open/Close (F:Close)"=TRUE) -> ("error out"=w1538:errorcluster)  [unwired: 9 in, 2 out]
                                }
                                frame True {
                                n620 = To Long Integer(number=w1545) -> (32bit integer=w1544:i32)
                                n621 = call "Valve Control Single 6008.vi"("Valve On?"=FALSE, "Valve Number"=w1544, "Port"=w1546) -> ()  [unwired: 8 in, 1 out]
                                }
                              }
                              n622 = case shown="1" w1528 {
                                tunnel: [Dryer_Test_State."Wait to Start" ("Test State") Dryer_Test_State."Watering" ("Test State")] -> w1534
                                frame 0, Default {
                                }
                                frame 1 {
                                }
                              }
                            }
                            frame True {
                              # "correct cycle, continue"
                            }
                          }
                        }
                        frame True {
                          # "time expired"
                          # "Turn off valve"
                          n623 = case shown="1" w1549 {
                            tunnel: [Dryer_Test_State."Drying" ("Test State") Dryer_Test_State."Pause Manual Station" ("Test State")] -> w1556
                            tunnel: w1548 -> [_ _]
                            frame 0, Default {
                            }
                            frame 1 {
                            }
                          }
                          n624 = case shown="False" w1551 {
                            tunnel: w1555 -> [w1564 _]
                            tunnel: w1554 -> [w1562 w1567]
                            tunnel: w1553 -> [w1561 _]
                            tunnel: [w1560 _] -> w1552
                            tunnel: w1550 -> [_ w1568]
                            frame False {
                              n625 = Number To Decimal String(number=w1562) -> (decimal integer string=w1559:string)  [unwired: 1 in]
                              n626 = call "Agilent Valve Control.vi"("Station In"=w1559, "Agilent Channels In"=w1564, "Agilent"=w1561, "Open/Close (F:Close)"=TRUE) -> ("error out"=w1560:errorcluster)  [unwired: 9 in, 2 out]
                            }
                            frame True {
                              n627 = To Long Integer(number=w1567) -> (32bit integer=w1566:i32)
                              n628 = call "Valve Control Single 6008.vi"("Valve On?"=FALSE, "Valve Number"=w1566, "Port"=w1568) -> ()  [unwired: 8 in, 1 out]
                            }
                          }
                        }
                      }
                    }
                    frame True {
                      # "initial watering, turn on water"
                      # "TURN ON VALVE during day shift.  Night, turn off valve."
                      n629 = call <vilib>:"Trim Whitespace.vi"("string"=w1577) -> ("trimmed string"=w1572:string)  [unwired: 1 in]
                      n630 = case shown="1" w1570 {
                        tunnel: [w1588 TRUE ("Day")] -> w1569
                        frame 0, Default {
                          n631 = local read "Day"() -> (w1588:bool)
                        }
                        frame 1 {
                        }
                      }
                      n632 = case shown="1" w1571 {
                        tunnel: w1579 -> [w1594 w1596]
                        tunnel: [w1593 w1596] -> w1578
                        tunnel: [w1592 TRUE ("Correct Cycle")] -> w1575
                        tunnel: w1572 -> [w1591 _]
                        tunnel: w1569 -> [w1590 _]
                        frame 0, Default {
                          n633 = call "Check Cycle Index.vi"("error in"=w1594, "Day"=w1590, "Cycle Index"=w1591) -> ("error out"=w1593:errorcluster, "Correct Cycle"=w1592:bool)  [unwired: 7 in]
                        }
                        frame 1 {
                        }
                      }
                      n634 = Compound Arithmetic op=AND(w1569, w1575) -> (w1576:bool)
                      n635 = case shown="False" w1582 {
                        tunnel: w1587 -> [w1613 w1622]
                        tunnel: w1578 -> [w1618 w1620]
                        tunnel: w1585 -> [w1617 _]
                        tunnel: w1584 -> [w1616 _]
                        tunnel: [w1615 w1619] -> w1583
                        tunnel: w1581 -> [_ w1623]
                        tunnel: w1576 -> [w1611 w1621]
                        frame False {
                          n636 = Not(x=w1611) -> (.not. x?=w1614:bool)
                          n637 = Number To Decimal String(number=w1613) -> (decimal integer string=w1612:string)  [unwired: 1 in]
                          n638 = call "Agilent Valve Control.vi"("Station In"=w1612, "Agilent Channels In"=w1617, "Agilent"=w1616, "Open/Close (F:Close)"=w1614, "error in (no error)"=w1618) -> ("error out"=w1615:errorcluster)  [unwired: 8 in, 2 out]
                        }
                        frame True {
                          n639 = call "Valve Control Single 6008.vi"("error in"=w1620, "Valve On?"=w1621, "Valve Number"=w1622, "Port"=w1623) -> ("error out"=w1619:errorcluster)  [unwired: 7 in]
                        }
                      }
                      n640 = case shown="True" w1575 {
                        tunnel: [0.0 ("Elapsed Time (sec)") w1609] -> w1586
                        tunnel: w1583 -> [w1607 w1610]
                        tunnel: [w1606 w1610] -> w1580
                        tunnel: w1574 -> [w1599 _]
                        tunnel: [Dryer_Test_State."Wait Com" ("Test State") Dryer_Test_State."Watering" ("Test State")] -> w1573
                        frame False {
                          w1601 = T19 7 items=["CMD_Eval_Mode_Entry_CC1", "CMD_Eval_Mode_Entry_CC2", "CMD_Eval_Mode_Continue", "CMD_Send_DIAG_Info", "CMD_Enable_Debug_Log ", "CMD_Disable_Debug_Log ", "CMD_Send_Log_Data", "CMD_Stop", "RQST_Version"] ("Command")
                          # "send error and turn off dryer\nif mismatch"
                          n641 = call "Com Chan Type Conversion.vi"("Com Chan"=w1599) -> ("VISA resource name"=w1600:refnum<visa-resource-name>)  [unwired: 11 in, 3 out]
                          n642 = call "GEA2_ICP_Dryer_SM.vi"("ComPort"=w1600, "Mode"=GEA2_Dryer_Interface_Ctrl."SendCMD", "Command"=w1601) -> ("Error Out"=w1597:errorcluster)  [unwired: 7 in, 5 out]
                          n643 = call <vilib>:"Clear Errors.vi"("error in (no error)"=w1597) -> ()  [unwired: 6 in, 1 out]
                          n644 = call "Error Bool Add Message.vi"("Error?"=TRUE, "Message"="Index Mismatch for Shift", "Error In"=w1607) -> ("Error Out"=w1606:errorcluster)  [unwired: 12 in]
                        }
                        frame True {
                          n645 = call "E-Time.vi"() -> ("Elapsed Time (sec)"=w1609:dbl)  [unwired: 9 in, 2 out]
                        }
                      }
                    }
                  }
                  n646 = case shown="Error" w1478 {
                    selector: w1478 -> [_ w1488]
                    tunnel: w1475 -> [_ w1491]
                    frame No Error {
                    }
                    frame Error {
                      n647 = local write "valve error out"(w1488) -> ()
                      n648 = Concatenate Strings("Valve Com Error Station: ", w1491) -> (→"User Notice":string)
                    }
                  }
                }
              }
            }
            frame True {
              # "If the user or program sets stop dryer command. This will allows the dryer to continue\ndrying but will not start the next cycle"
            }
          }
        }
        n649 = call <vilib>:"Add State(s) to Queue__jki_lib_state_machine.vi"("State(s) in (\"\")"=w1438) -> ("States Out"=w1437:string)  [unwired: 14 in]
        n650 = Bundle By Name(cluster=w1435, "Station Test State"=w1433, "Station Timer"=w1430) -> (w1434:T16)
      }
      frame "Pause Manual Stations" {
        # "This state allows dryers without GEA2 communications to start and stop.\nIn its current state, you must short the start switch out on the board (this is what\nthe agilent is for)"
        # "Wait for both status and log to be reported."
        n651 = Unbundle By Name(w1641) -> ("Station Timer"=w1632:dbl[], "Station Test State"=w1636:T8[], "Start Buttons."=w1634:T3[], "Pause Timer"=w1630:i32[], "All Test Stations Control"=w1628:T1[], "Emergency Timer"=w1627:i32[])
        n652 = Equal?(x=Dryer_Test_State."Pause Manual Station" ("Test State"), y=w1636) -> (x = y?=w1637:bool[])
        n653 = for {
          tunnel: w1637 -> [w1655] mode=indexing
          tunnel: w1636 -> [w1654] mode=indexing
          tunnel: [w1653] -> w1635 mode=indexing
          tunnel: w1628 -> [w1646] mode=indexing
          tunnel: w1634 -> [w1652]
          tunnel: [w1649] -> w1633 mode=indexing
          tunnel: w1632 -> [w1651] mode=indexing
          tunnel: "Manual Station Pause" -> [w1650]
          tunnel: w1630 -> [w1648] mode=indexing
          tunnel: [w1647] -> w1629 mode=indexing
          tunnel: w1627 -> [w1644] mode=indexing
          n654 = Greater Than 0?(x=w1644) -> (x > 0?=w1645:bool)
          n655 = case shown="False" w1645 {
            tunnel: w1655 -> [w1665 _]
            tunnel: w1654 -> [w1664 w1702]
            tunnel: [w1663 w1702] -> w1653
            tunnel: w1652 -> [w1662 _]
            tunnel: w1651 -> [w1661 w1703]
            tunnel: w1650 -> [w1660 _]
            tunnel: [w1659 w1703] -> w1649
            tunnel: w1648 -> [w1658 w1701]
            tunnel: [w1657 w1701] -> w1647
            tunnel: w1646 -> [w1656 _]
            frame False {
              n656 = case shown="True" w1665 {
                tunnel: w1664 -> [w1668 _]
                tunnel: [w1668 w1682] -> w1663
                tunnel: w1656 -> [_ w1675]
                tunnel: w1662 -> [_ w1681]
                tunnel: [w1667 w1680] -> w1659
                tunnel: w1661 -> [w1667 w1672]
                tunnel: w1660 -> [_ w1673]
                tunnel: w1658 -> [w1666 w1670]
                tunnel: [w1666 w1669] -> w1657
                frame False {
                }
                frame True {
                  n657 = call "E-Time.vi"() -> ("Elapsed Time (sec)"=w1679:dbl)  [unwired: 9 in, 2 out]
                  n658 = Unbundle By Name(w1675) -> ("Station Index"=w1683:i32)
                  n659 = Subtract(x=w1679, y=w1672) -> (x-y=w1676:dbl)
                  n660 = Subtract(x=w1676, y=w1673) -> (x-y=w1678:dbl)
                  n661 = Equal?(x=w1670, y=0) -> (x = y?=w1674:bool)
                  n662 = Greater Than 0?(x=w1678) -> (x > 0?=w1677:bool)
                  n663 = case shown="False" w1674 {
                    tunnel: w1683 -> [w1688 w1698]
                    tunnel: [w1687 Dryer_Test_State."Pause Manual Station" ("Test State")] -> w1682
                    tunnel: w1681 -> [w1686 w1696]
                    tunnel: [w1684 w1695] -> w1680
                    tunnel: w1677 -> [w1685 _]
                    tunnel: w1672 -> [w1684 _]
                    frame False {
                      n664 = case shown="True" w1685 {
                        tunnel: w1688 -> [_ w1692]
                        tunnel: [Dryer_Test_State."Pause Manual Station" ("Test State") Dryer_Test_State."Drying" ("Test State")] -> w1687
                        tunnel: w1686 -> [_ w1690]
                        frame False {
                          # "Time is not up. Continue\nPause"
                        }
                        frame True {
                          # "Times up. Start drying"
                          n665 = Number To Decimal String(number=w1692) -> (decimal integer string=w1693:string)  [unwired: 1 in]
                          n666 = local read "Agilent"() -> (w1694:T9)
                          n667 = call "Agilent Start Button.vi"("Station In"=w1693, "Agilent Channels In"=w1690, "Agilent"=w1694) -> ()  [unwired: 11 in, 2 out]
                        }
                      }
                    }
                    frame True {
                      # "Turn off the dryer."
                      n668 = local read "Agilent"() -> (w1700:T9)
                      n669 = Number To Decimal String(number=w1698) -> (decimal integer string=w1699:string)  [unwired: 1 in]
                      n670 = call "Agilent Start Button.vi"("Station In"=w1699, "Agilent Channels In"=w1696, "Agilent"=w1700) -> ()  [unwired: 11 in, 2 out]
                      n671 = call "E-Time.vi"() -> ("Elapsed Time (sec)"=w1695:dbl)  [unwired: 9 in, 2 out]
                    }
                  }
                  n672 = Increment(x=w1670) -> (x+1=w1669:i32)
                }
              }
            }
            frame True {
              # "If the user or program sets stop dryer command. This will allows the dryer to continue\ndrying but will not start the next cycle"
            }
          }
        }
        n673 = Bundle By Name(cluster=w1641, "Station Test State"=w1635, "Station Timer"=w1633, "Pause Timer"=w1629) -> (w1640:T16)
        n674 = call <vilib>:"Add State(s) to Queue__jki_lib_state_machine.vi"("State(s) in (\"\")"=w1643) -> ("States Out"=w1642:string)  [unwired: 14 in]
      }
      frame "Drying" {
        # "Keyword New, means dryer has been replaced during dry cycle"
        # "The check is that both string lengths are > 0. Assumes that these are initializied to \"\""
        # "Wait for both status and log to be reported."
        n675 = Unbundle By Name(w1714) -> ("Emergency Timer"=w1704:i32[], "All Test Stations Control"=w1705:T1[], "Station Test State"=w1708:T8[], "Station Timer"=w1709:dbl[])
        n676 = Equal?(x=Dryer_Test_State."Drying" ("Test State"), y=w1708) -> (x = y?=w1715:bool[])
        n677 = local write "Station Test State"(w1708) -> ()
        n678 = for {
          tunnel: w1715 -> [w1727] mode=indexing
          tunnel: w1705 -> [w1720] mode=indexing
          tunnel: [w1726] -> w1712 mode=indexing
          tunnel: w1708 -> [w1725] mode=indexing
          tunnel: [w1724] -> w1710 mode=indexing
          tunnel: w1709 -> [w1723] mode=indexing
          tunnel: w1707 -> [w1722]
          tunnel: [w1721] -> w1706
          tunnel: w1704 -> [w1719] mode=indexing
          n679 = Greater Than 0?(x=w1719) -> (x > 0?=w1718:bool)
          n680 = case shown="True" w1718 {
            tunnel: w1727 -> [w1735 _]
            tunnel: [w1734 w1784] -> w1726
            tunnel: w1725 -> [w1733 w1784]
            tunnel: [w1732 w1783] -> w1724
            tunnel: w1723 -> [w1731 w1783]
            tunnel: w1722 -> [w1730 w1785]
            tunnel: [w1729 w1785] -> w1721
            tunnel: w1720 -> [w1728 _]
            frame False {
              # "Cycle through stations."
              n681 = case shown="True" w1735 {
                tunnel: w1728 -> [_ w1757]
                tunnel: [w1738 w1755] -> w1734
                tunnel: w1733 -> [w1738 w1754]
                tunnel: [w1737 w1753] -> w1732
                tunnel: w1731 -> [w1737 w1752]
                tunnel: w1730 -> [w1736 w1748]
                tunnel: [w1736 w1747] -> w1729
                frame False {
                  # "Not drying.  Continue to next state."
                }
                frame True {
                  n682 = Unbundle By Name(w1757) -> ("Dryer Details.Status"=w1743:string, "Bad Com Count"=w1740:i32)
                  n683 = global read "Globals Wilt.vi" "New Dryer Status String"() -> (w1750:string)
                  n684 = global read "Globals Wilt.vi" "Bad Com Limit"() -> (w1739:i32)
                  n685 = call "Type Conv - Dryer Status to Txt.vi"("Status"=Dryer_Status_Ctrl."Err") -> ("Ring Text.Text"=w1745:string)  [unwired: 10 in]
                  n686 = call "Type Conv - Dryer Status to Txt.vi"("Status"=Dryer_Status_Ctrl."Cycle Completed") -> ("Ring Text.Text"=w1744:string)  [unwired: 10 in]
                  n687 = Equal?(x=w1745, y=w1743) -> (x = y?=w1746:bool)
                  n688 = Equal?(x=w1743, y=w1750) -> (x = y?=w1751:bool)
                  n689 = Equal?(x=w1744, y=w1743) -> (x = y?=w1756:bool)
                  n690 = Greater?(x=w1740, y=w1739) -> (0:w1741:bool)
                  n691 = And(x=w1746, y=w1741) -> (x .and. y?=w1742:bool)
                  n692 = case shown="False" w1756 {
                    tunnel: [w1763 Dryer_Test_State."Cooldown" ("Test State")] -> w1755
                    tunnel: w1754 -> [w1762 _]
                    tunnel: [w1765 w1781] -> w1753
                    tunnel: w1752 -> [w1764 _]
                    tunnel: w1751 -> [w1766 _]
                    tunnel: w1748 -> [w1761 w1780]
                    tunnel: [w1760 w1780] -> w1747
                    tunnel: w1742 -> [w1759 _]
                    frame False {
                      n693 = case shown="False" w1766 {
                        tunnel: [w1772 w1779] -> w1765
                        tunnel: w1764 -> [w1772 w1779]
                        tunnel: [w1768 Dryer_Test_State."Wait Com" ("Test State")] -> w1763
                        tunnel: w1762 -> [w1767 _]
                        tunnel: w1761 -> [w1771 w1777]
                        tunnel: [w1770 w1777] -> w1760
                        tunnel: w1759 -> [w1769 _]
                        frame False {
                          n694 = case shown="True" w1769 {
                            tunnel: w1771 -> [w1774 w1775]
                            tunnel: [w1774 w1775] -> w1770
                            tunnel: [w1773 Dryer_Test_State."Wait Com" ("Test State")] -> w1768
                            tunnel: w1767 -> [w1773 _]
                            frame False {
                              # "Drying normally"
                            }
                            frame True {
                              # "Error"
                            }
                          }
                        }
                        frame True {
                          # "New dyer."
                        }
                      }
                    }
                    frame True {
                      # "Cycle is completed."
                      n695 = call "E-Time.vi"() -> ("Elapsed Time (sec)"=w1781:dbl)  [unwired: 9 in, 2 out]
                    }
                  }
                }
              }
            }
            frame True {
              # "If the user or program sets stop dryer command. This will allows the dryer to continue\ndrying but will not start the next cycle"
            }
          }
        }
        n696 = call <vilib>:"Add State(s) to Queue__jki_lib_state_machine.vi"("State(s) in (\"\")"=w1717) -> ("States Out"=w1716:string)  [unwired: 14 in]
        n697 = Bundle By Name(cluster=w1714, "Station Test State"=w1712, "Station Timer"=w1710) -> (w1713:T16)
      }
      frame "Cooldown" {
        # "The check is that both string lengths are > 0. Assumes that these are initializied to \"\""
        # "Wait for both status and log to be reported."
        n698 = Unbundle By Name(w1798) -> ("Station Test State"=w1791:T8[], "Station Timer"=w1794:dbl[], "Station Com List"=w1789:u8[], "Start Buttons."=w1788:T3[], "All Test Stations Control"=w1787:T1[], "Emergency Timer"=w1786:i32[])
        n699 = Equal?(x=Dryer_Test_State."Cooldown" ("Test State"), y=w1791) -> (x = y?=w1799:bool[])
        n700 = local write "Station Test State"(w1791) -> ()
        n701 = for {
          tunnel: w1799 -> [w1812] mode=indexing
          tunnel: [w1811] -> w1796 mode=indexing
          tunnel: w1791 -> [w1810] mode=indexing
          tunnel: w1794 -> [w1809] mode=indexing
          tunnel: w1793 -> [w1808]
          tunnel: [w1807] -> w1792
          tunnel: w1789 -> [w1806] mode=indexing
          tunnel: w1787 -> [w1804] mode=indexing
          tunnel: w1788 -> [w1805]
          tunnel: w1786 -> [w1802] mode=indexing
          n702 = Greater Than 0?(x=w1802) -> (x > 0?=w1803:bool)
          n703 = case shown="False" w1803 {
            tunnel: w1812 -> [w1821 _]
            tunnel: [w1820 w1866] -> w1811
            tunnel: w1810 -> [w1819 w1866]
            tunnel: w1809 -> [w1818 _]
            tunnel: w1808 -> [w1817 w1867]
            tunnel: [w1816 w1867] -> w1807
            tunnel: w1806 -> [w1815 _]
            tunnel: w1805 -> [w1814 _]
            tunnel: w1804 -> [w1813 _]
            frame False {
              # "cycle through stations"
              n704 = case shown="True" w1821 {
                tunnel: [w1823 w1838] -> w1820
                tunnel: w1819 -> [w1823 w1837]
                tunnel: w1818 -> [_ w1835]
                tunnel: w1817 -> [w1822 w1830]
                tunnel: [w1822 w1829] -> w1816
                tunnel: w1815 -> [_ w1828]
                tunnel: w1813 -> [_ w1827]
                tunnel: w1814 -> [_ w1824]
                frame False {
                }
                frame True {
                  # "in cooldown."
                  n705 = Unbundle By Name(w1827) -> ("Station Index"=w1825:i32, "Dryer Details.Run w/o Newfi"=w1826:i32)
                  n706 = call "E-Time.vi"() -> ("Elapsed Time (sec)"=w1836:dbl)  [unwired: 9 in, 2 out]
                  n707 = Subtract(x=w1836, y=w1835) -> (x-y=w1834:dbl)
                  n708 = Subtract(x=w1834, y="Cooldown time") -> (x-y=w1832:dbl)
                  n709 = Greater Than 0?(x=w1832) -> (x > 0?=w1831:bool)
                  n710 = case shown="True" w1831 {
                    tunnel: [w1840 Dryer_Test_State."Wait to Start" ("Test State")] -> w1838
                    tunnel: w1837 -> [w1840 _]
                    tunnel: w1830 -> [w1839 w1846]
                    tunnel: [w1839 w1845] -> w1829
                    tunnel: w1828 -> [_ w1844]
                    tunnel: w1826 -> [_ w1843]
                    tunnel: w1825 -> [_ w1842]
                    tunnel: w1824 -> [_ w1841]
                    frame False {
                      # "cooling down."
                    }
                    frame True {
                      # "after cooldown time, send continue cmd."
                      n711 = case shown="1" w1843 {
                        tunnel: w1846 -> [w1851 w1865]
                        tunnel: [w1850 w1862] -> w1845
                        tunnel: w1844 -> [w1849 _]
                        tunnel: w1842 -> [_ w1864]
                        tunnel: w1841 -> [_ w1857]
                        frame 0, Default {
                          n712 = for {
                            N: 3 -> [_]
                            tunnel: w1851 -> [w1856]
                            tunnel: [w1855] -> w1850
                            tunnel: w1849 -> [w1852]
                            n713 = call "Com Chan Type Conversion.vi"("Com Chan"=w1852) -> ("VISA resource name"=w1854:refnum<visa-resource-name>)  [unwired: 11 in, 3 out]
                            n714 = call "GEA2_ICP_Dryer_SM.vi"("ComPort"=w1854, "Mode"=GEA2_Dryer_Interface_Ctrl."Send Continue CMD", "Error In"=w1856) -> ("Error Out"=w1855:errorcluster)  [unwired: 7 in, 5 out]
                          }
                        }
                        frame 1 {
                          n715 = Number To Decimal String(number=w1864) -> (decimal integer string=w1861:string)  [unwired: 1 in]
                          n716 = local read "Agilent"() -> (w1863:T9)
                          n717 = call "Agilent Start Button.vi"("Station In"=w1861, "Agilent Channels In"=w1857, "Agilent"=w1863, "error in (no error)"=w1865) -> ("error out"=w1860:errorcluster)  [unwired: 10 in, 1 out]
                          n718 = call "Delay mS.vi"("Error In"=w1860, "milliseconds to wait"=u32 500) -> ("Error Out"=w1859:errorcluster)  [unwired: 13 in]
                          n719 = call "Agilent Start Button.vi"("Station In"=w1861, "Agilent Channels In"=w1857, "Agilent"=w1863, "error in (no error)"=w1859) -> ("error out"=w1862:errorcluster)  [unwired: 10 in, 1 out]
                        }
                      }
                    }
                  }
                }
              }
            }
            frame True {
              # "If the user or program sets stop dryer command. This will allows the dryer to continue\ndrying but will not start the next cycle"
            }
          }
        }
        n720 = call <vilib>:"Add State(s) to Queue__jki_lib_state_machine.vi"("State(s) in (\"\")"=w1801) -> ("States Out"=w1800:string)  [unwired: 14 in]
        n721 = call <vilib>:"Clear Errors.vi"("error in (no error)"=w1792) -> ("error out"=w1790:errorcluster)  [unwired: 6 in]
        n722 = Bundle By Name(cluster=w1798, "Station Test State"=w1796) -> (w1797:T16)
      }
      frame "Continue" {
        # "If Dryer goes paused, save the test state, restore it when the dryer becomes unpaused.\n\nIf the saved state is Watering, when going into paused, shut valve.  Save the Elapsed time into station timer.\nIf coming out of paused into watering, turn on the valve."
        n723 = Unbundle By Name(w1882) -> ("All Test Stations Control"=w1871:T1[], "Station Test State"=w1876:T8[], "Station Timer"=w1878:dbl[], "Saved Test State"=w1877:T8[], "Agilent Channels Water Valves."=w1872:T3[], "USB6008"=w1870:tag, "Remote Station"=w1869:bool, "Emergency Timer"=w1868:i32[])
        n724 = local write "Station Test State"(w1876) -> ()
        n725 = for {
          tunnel: w1871 -> [w1901] mode=indexing
          tunnel: [w1900] -> w1880 mode=indexing
          tunnel: w1876 -> [w1891] mode=indexing
          tunnel: [w1899] -> w1879 mode=indexing
          tunnel: w1878 -> [w1898] mode=indexing
          tunnel: w1877 -> [w1896] mode=indexing
          tunnel: [w1895] -> w1875 mode=indexing
          tunnel: w1874 -> [w1893]
          tunnel: [w1892] -> w1873
          tunnel: w1872 -> [w1890]
          tunnel: w1870 -> [w1889]
          tunnel: w1869 -> [w1888]
          tunnel: w1868 -> [w1885] mode=indexing
          n726 = Unbundle By Name(w1901) -> ("Station Index"=w1894:i32, "Dryer Details.Status"=w1897:string, "Dryer Details.24 Hour Water Injection"=w1887:i32)
          n727 = Greater Than 0?(x=w1885) -> (x > 0?=w1886:bool)
          n728 = case shown="False" w1886 {
            tunnel: [w1919 w2016] -> w1900
            tunnel: [w1918 w2017] -> w1899
            tunnel: w1898 -> [w1917 w2017]
            tunnel: w1897 -> [w1916 _]
            tunnel: w1896 -> [w1911 w2015]
            tunnel: [w1910 w2015] -> w1895
            tunnel: w1894 -> [w1909 _]
            tunnel: w1893 -> [w1908 w2014]
            tunnel: [w1907 w2014] -> w1892
            tunnel: w1891 -> [w1906 w2016]
            tunnel: w1890 -> [w1905 _]
            tunnel: w1889 -> [w1904 _]
            tunnel: w1888 -> [w1903 _]
            tunnel: w1887 -> [w1902 _]
            frame False {
              n729 = call "Type Conv - Dryer Status to Txt.vi"("Status"=Dryer_Status_Ctrl."Paused") -> ("Ring Text.Text"=w1915:string)  [unwired: 10 in]
              n730 = Equal?(x=w1916, y=w1915) -> (x = y?=w1913:bool)
              n731 = case shown="True" w1913 {
                tunnel: [w1929 Dryer_Test_State."Paused" ("Test State")] -> w1919
                tunnel: w1906 -> [w1932 w1970]
                tunnel: [w1935 w1968] -> w1918
                tunnel: w1917 -> [w1935 w1969]
                tunnel: Dryer_Test_State."Paused" ("Test State") -> [w1934 w1975]
                tunnel: w1911 -> [w1933 w1971]
                tunnel: [w1933 w1972] -> w1910
                tunnel: w1909 -> [w1926 w1973]
                tunnel: w1908 -> [w1925 w1967]
                tunnel: [w1924 w1967] -> w1907
                tunnel: w1905 -> [w1923 w1966]
                tunnel: w1904 -> [w1922 w1965]
                tunnel: w1903 -> [w1921 w1964]
                tunnel: w1902 -> [w1920 _]
                frame False {
                  # "Dryer not paused."
                  n732 = Equal?(x=w1932, y=w1934) -> (x = y?=w1927:bool)
                  n733 = Select(t=w1933, s=w1927, f=w1932) -> (s? t:f=w1929:T8)
                  n734 = Equal?(x=w1929, y=Dryer_Test_State."Watering" ("Test State")) -> (x = y?=w1930:bool)
                  n735 = And(x=w1927, y=w1930) -> (x .and. y?=w1928:bool)
                  n736 = case shown="True" w1928 {
                    tunnel: w1926 -> [_ w1943]
                    tunnel: w1925 -> [w1936 w1942]
                    tunnel: [w1936 w1941] -> w1924
                    tunnel: w1923 -> [_ w1940]
                    tunnel: w1922 -> [_ w1939]
                    tunnel: w1921 -> [_ w1938]
                    tunnel: w1920 -> [_ w1937]
                    frame False {
                    }
                    frame True {
                      # "TURN ON VALVE during day shift.  Night, turn off valve."
                      # "turn on valve"
                      n737 = local read "Agilent"() -> (w1944:T9)
                      n738 = case shown="False" w1938 {
                        tunnel: w1943 -> [w1947 w1959]
                        tunnel: w1942 -> [w1953 w1958]
                        tunnel: w1940 -> [w1952 _]
                        tunnel: w1944 -> [w1951 _]
                        tunnel: [w1950 w1957] -> w1941
                        tunnel: w1939 -> [_ w1961]
                        tunnel: w1937 -> [w1945 w1956]
                        frame False {
                          n739 = case shown="0, Default" w1945 {
                            tunnel: [w1954 TRUE ("Day")] -> w1949
                            frame 0, Default {
                              n740 = local read "Day"() -> (w1954:bool)
                            }
                            frame 1 {
                            }
                          }
                          n741 = Not(x=w1949) -> (.not. x?=w1948:bool)
                          n742 = Number To Decimal String(number=w1947) -> (decimal integer string=w1946:string)  [unwired: 1 in]
                          n743 = call "Agilent Valve Control.vi"("Station In"=w1946, "Agilent Channels In"=w1952, "Agilent"=w1951, "Open/Close (F:Close)"=w1948, "error in (no error)"=w1953) -> ("error out"=w1950:errorcluster)  [unwired: 8 in, 2 out]
                        }
                        frame True {
                          n744 = case shown="0, Default" w1956 {
                            tunnel: [w1962 TRUE ("Day")] -> w1960
                            frame 0, Default {
                              n745 = local read "Day"() -> (w1962:bool)
                            }
                            frame 1 {
                            }
                          }
                          n746 = call "Valve Control Single 6008.vi"("error in"=w1958, "Valve On?"=w1960, "Valve Number"=w1959, "Port"=w1961) -> ("error out"=w1957:errorcluster)  [unwired: 7 in]
                        }
                      }
                    }
                  }
                }
                frame True {
                  # "Dryer in paused state."
                  n747 = Not Equal?(x=w1970, y=w1975) -> (x != y?=w1974:bool)
                  n748 = case shown="True" w1974 {
                    tunnel: w1973 -> [_ w1993]
                    tunnel: [w1979 w1992] -> w1972
                    tunnel: w1971 -> [w1979 _]
                    tunnel: w1970 -> [_ w1992]
                    tunnel: w1969 -> [w1978 w1990]
                    tunnel: [w1977 w1991] -> w1968
                    tunnel: w1966 -> [_ w1989]
                    tunnel: w1965 -> [_ w1988]
                    tunnel: w1964 -> [_ w1987]
                    frame False {
                      # "Station In Paused State."
                      n749 = case shown="\"Cooldown\"" w1979 {
                        tunnel: w1978 -> [_ w1982 w1984]
                        tunnel: [w1980 w1981 w1985] -> w1977
                        frame "No SN", Default {
                          n750 = call "E-Time.vi"() -> ("Elapsed Time (sec)"=w1980:dbl)  [unwired: 9 in, 2 out]
                        }
                        frame "Watering" {
                          n751 = call "E-Time.vi"() -> ("Elapsed Time (sec)"=w1983:dbl)  [unwired: 9 in, 2 out]
                          n752 = Subtract(x=w1983, y=w1982) -> (x-y=w1981:dbl)
                        }
                        frame "Cooldown" {
                          n753 = call "E-Time.vi"() -> ("Elapsed Time (sec)"=w1986:dbl)  [unwired: 9 in, 2 out]
                          n754 = Subtract(x=w1986, y=w1984) -> (x-y=w1985:dbl)
                        }
                      }
                    }
                    frame True {
                      # "First time detected paused."
                      n755 = case shown="\"Watering\"" w1992 {
                        tunnel: w1993 -> [_ _ _ w2003]
                        tunnel: [w1994 w1995 0.0 ("element") w2001] -> w1991
                        tunnel: w1990 -> [_ _ _ w2000]
                        tunnel: w1989 -> [_ _ _ w1999]
                        tunnel: w1988 -> [_ _ _ w1998]
                        tunnel: w1987 -> [_ _ _ w1997]
                        frame "No SN", Default {
                          n756 = call "E-Time.vi"() -> ("Elapsed Time (sec)"=w1994:dbl)  [unwired: 9 in, 2 out]
                        }
                        frame "Wait Com" {
                          n757 = call "E-Time.vi"() -> ("Elapsed Time (sec)"=w1995:dbl)  [unwired: 9 in, 2 out]
                        }
                        frame "Wait to Start" {
                        }
                        frame "Watering" {
                          # "Turn off valve"
                          n758 = local read "Agilent"() -> (w2004:T9)
                          n759 = case shown="False" w1997 {
                            tunnel: w1999 -> [w2009 _]
                            tunnel: w2003 -> [w2007 w2012]
                            tunnel: w2004 -> [w2006 _]
                            tunnel: w1998 -> [_ w2013]
                            frame False {
                              n760 = Number To Decimal String(number=w2007) -> (decimal integer string=w2005:string)  [unwired: 1 in]
                              n761 = call "Agilent Valve Control.vi"("Station In"=w2005, "Agilent Channels In"=w2009, "Agilent"=w2006, "Open/Close (F:Close)"=TRUE) -> ()  [unwired: 9 in, 3 out]
                            }
                            frame True {
                              n762 = To Long Integer(number=w2012) -> (32bit integer=w2011:i32)
                              n763 = call "Valve Control Single 6008.vi"("Valve On?"=FALSE, "Valve Number"=w2011, "Port"=w2013) -> ()  [unwired: 8 in, 1 out]
                            }
                          }
                          n764 = call "E-Time.vi"() -> ("Elapsed Time (sec)"=w2002:dbl)  [unwired: 9 in, 2 out]
                          n765 = Subtract(x=w2002, y=w2000) -> (x-y=w2001:dbl)
                        }
                      }
                    }
                  }
                }
              }
            }
            frame True {
              # "If the user or program sets stop dryer command. This will allows the dryer to continue\ndrying but will not start the next cycle"
            }
          }
        }
        n766 = call <vilib>:"Add State(s) to Queue__jki_lib_state_machine.vi"("State(s) in (\"\")"=w1884) -> ("States Out"=w1883:string)  [unwired: 14 in]
        n767 = Bundle By Name(cluster=w1882, "Station Test State"=w1880, "Station Timer"=w1879, "Saved Test State"=w1875) -> (w1881:T16)
        n768 = local write "Saved Test State"(w1875) -> ()
      }
      frame "Update From DAQ Loop" {
        n769 = local read "GUI Aisle 1"() -> (w2022:T1[])
        n770 = local read "GUI Aisle 1A"() -> (w2021:T1[])
        n771 = local read "GUI Aisle 2"() -> (w2020:T1[])
        n772 = local read "GUI Aisle 3"() -> (w2019:T1[])
        n773 = local read "GUI Aisle 4"() -> (w2018:T1[])
        n774 = Bundle By Name(cluster=w2024, "GUI Aisle 1"=w2022, "GUI Aisle 1A"=w2021, "GUI Aisle 2"=w2020, "GUI Aisle 3"=w2019, "GUI Aisle 4"=w2018) -> (w2023:T16)
        n775 = call <vilib>:"Add State(s) to Queue__jki_lib_state_machine.vi"("State(s) in (\"\")"=w2027) -> ("States Out"=w2026:string)  [unwired: 14 in]
      }
      frame "Emergency Shutoff" {
        n776 = Unbundle By Name(w2031) -> ("USB6008"=w2038:tag, "All Test Stations Control"=w2040:T1[], "Remote Station"=w2039:bool, "Agilent Channels Water Valves."=w2037:T3[], "Station Timer"=w2034:dbl[], "Emergency Timer"=w2032:i32[])
        "Emergency Timer." <- w2032
        n777 = for {
          tunnel: w2040 -> [w2051] mode=indexing
          tunnel: w2039 -> [w2057]
          tunnel: w2038 -> [w2056]
          tunnel: w2037 -> [w2055]
          shift-right: [w2053] -> w2035
          shift-left: w2036 -> [w2054]
          tunnel: w2034 -> [w2043] mode=indexing
          tunnel: "Emergency Valve Timer" -> [w2044]
          tunnel: w2032 -> [w2045] mode=indexing
          tunnel: [w2052] -> w2029 mode=indexing
          tunnel: [w2046] -> w2028 mode=indexing
          n778 = Unbundle By Name(w2051) -> ("Status Color"=w2059:u32)
          n779 = global read "Globals Wilt.vi" "Temperature Fault"() -> (w2058:u32)
          n780 = Unbundle By Name(w2051) -> ("Station Index"=w2050:i32)
          n781 = Equal?(x=w2059, y=w2058) -> (x = y?=w2049:bool)
          n782 = Greater Than 0?(x=w2045) -> (x > 0?=w2048:bool)
          n783 = Or(x=w2049, y=w2048) -> (x .or. y?=w2047:bool)
          n784 = case shown="True" w2047 {
            tunnel: w2057 -> [_ w2079]
            tunnel: w2056 -> [_ w2078]
            tunnel: w2055 -> [_ w2077]
            tunnel: w2050 -> [_ w2076]
            tunnel: w2054 -> [w2062 w2075]
            tunnel: [w2062 w2074] -> w2053
            tunnel: w2045 -> [w2061 w2069]
            tunnel: [w2061 w2073] -> w2052
            tunnel: [w2060 w2072] -> w2046
            tunnel: w2044 -> [_ w2064]
            tunnel: w2043 -> [w2060 w2063]
            frame False {
            }
            frame True {
              n785 = call "E-Time.vi"() -> ("Elapsed Time (sec)"=w2066:dbl)  [unwired: 9 in, 2 out]
              n786 = Subtract(x=w2066, y=w2063) -> (x-y=w2067:dbl)
              n787 = Subtract(x=w2067, y=w2064) -> (x-y=w2068:dbl)
              n788 = Greater Than 0?(x=w2068) -> (x > 0?=w2065:bool)
              n789 = Equal?(x=w2069, y=0) -> (x = y?=w2070:bool)
              n790 = case shown="True" w2070 {
                tunnel: w2079 -> [w2081 w2113]
                tunnel: w2078 -> [w2083 w2112]
                tunnel: w2077 -> [w2085 w2111]
                tunnel: w2076 -> [w2084 w2110]
                tunnel: w2075 -> [w2087 w2109]
                tunnel: [w2086 w2108] -> w2074
                tunnel: w2065 -> [w2082 _]
                tunnel: [w2080 w2107] -> w2072
                tunnel: w2063 -> [w2080 _]
                frame False {
                  n791 = case shown="True" w2082 {
                    tunnel: w2087 -> [w2088 w2094]
                    tunnel: [w2088 w2093] -> w2086
                    tunnel: w2085 -> [_ w2092]
                    tunnel: w2084 -> [_ w2091]
                    tunnel: w2083 -> [_ w2090]
                    tunnel: w2081 -> [_ w2089]
                    frame False {
                    }
                    frame True {
                      n792 = case shown="False" w2089 {
                        tunnel: w2090 -> [_ w2106]
                        tunnel: w2092 -> [w2101 _]
                        tunnel: w2091 -> [w2100 w2105]
                        tunnel: w2094 -> [w2099 w2104]
                        tunnel: [w2098 w2103] -> w2093
                        frame False {
                          # "Turn Valve Off"
                          n793 = Number To Decimal String(number=w2100) -> (decimal integer string=w2097:string)  [unwired: 1 in]
                          n794 = local read "Agilent"() -> (w2096:T9)
                          n795 = call "Agilent Valve Control.vi"("Station In"=w2097, "Agilent Channels In"=w2101, "Agilent"=w2096, "Open/Close (F:Close)"=TRUE, "error in (no error)"=w2099) -> ("error out"=w2098:errorcluster)  [unwired: 8 in, 2 out]
                        }
                        frame True {
                          # "Turn Valve Off"
                          n796 = call "Valve Control Single 6008.vi"("error in"=w2104, "Valve On?"=FALSE, "Valve Number"=w2105, "Port"=w2106) -> ("error out"=w2103:errorcluster)  [unwired: 7 in]
                        }
                      }
                    }
                  }
                }
                frame True {
                  n797 = case shown="False" w2113 {
                    tunnel: w2112 -> [_ w2125]
                    tunnel: w2111 -> [w2120 _]
                    tunnel: w2110 -> [w2119 w2124]
                    tunnel: w2109 -> [w2118 w2123]
                    tunnel: [w2117 w2122] -> w2108
                    frame False {
                      # "Turn Valve On"
                      n798 = Number To Decimal String(number=w2119) -> (decimal integer string=w2116:string)  [unwired: 1 in]
                      n799 = local read "Agilent"() -> (w2115:T9)
                      n800 = call "Agilent Valve Control.vi"("Station In"=w2116, "Agilent Channels In"=w2120, "Agilent"=w2115, "Open/Close (F:Close)"=FALSE, "error in (no error)"=w2118) -> ("error out"=w2117:errorcluster)  [unwired: 8 in, 2 out]
                    }
                    frame True {
                      # "Turn Valve On"
                      n801 = call "Valve Control Single 6008.vi"("error in"=w2123, "Valve On?"=TRUE, "Valve Number"=w2124, "Port"=w2125) -> ("error out"=w2122:errorcluster)  [unwired: 7 in]
                    }
                  }
                  n802 = call "E-Time.vi"() -> ("Elapsed Time (sec)"=w2107:dbl)  [unwired: 9 in, 2 out]
                }
              }
              n803 = Increment(x=w2069) -> (x+1=w2073:i32)
            }
          }
        }
        n804 = Bundle By Name(cluster=w2031, "Station Timer"=w2028, "Emergency Timer"=w2029) -> (w2030:T16)
        n805 = call <vilib>:"Add State(s) to Queue__jki_lib_state_machine.vi"("State(s) in (\"\")"=w2042) -> ("States Out"=w2041:string)  [unwired: 14 in]
      }
      frame "Check E-Timer" {
        n806 = Unbundle By Name(w2129) -> ("Emergency Timer"=w2127:i32[])
        n807 = case shown="True" "Reset E-Timer" {
          tunnel: w2127 -> [w2135 w2137]
          tunnel: [w2135 w2136] -> w2126
          frame False {
          }
          frame True {
            n808 = Array Size(array=w2137) -> (size(s)=w2139:i32)
            n809 = Initialize Array(0 ("Number of Units"), w2139) -> (w2136:i32[])
          }
        }
        n810 = Bundle By Name(cluster=w2129, "Emergency Timer"=w2126) -> (w2131:T16)
        n811 = call <vilib>:"Add State(s) to Queue__jki_lib_state_machine.vi"("State(s) in Front (\"\")"="Start Test" ("State(s) in Front (\"\")"), "State(s) in (\"\")"=w2134) -> ("States Out"=w2133:string)  [unwired: 13 in]
      }
    }
    n812 = case shown="True" "Debug" {
      tunnel: w374 -> [_ w390]
      tunnel: [w385 w387] -> w373
      tunnel: w372 -> [w385 w389]
      frame False {
      }
      frame True {
        n813 = Build Array (concatenate)(w389, w390) -> (w386:string[])
        "Test State array" <- w386
        n814 = Array Size(array=w386) -> (size(s)=w388:i32)
        n815 = case shown="100" w388 {
          tunnel: [w391 w394] -> w387
          tunnel: w386 -> [w391 w395]
          frame 0, Default {
          }
          frame 100 {
            n816 = Delete From Array(array=w395, length=5, index=0) -> (array with subset deleted=w394:string[])  [unwired: 1 out]
          }
        }
      }
    }
    n817 = Wait Until Next ms Multiple(millisecond multiple=u32 50) -> ()  [unwired: 1 out]
  }
  "Test Complete" <- w6
  n818 = while "UI State Machine" {
    shift-right: [w2144] -> _
    shift-left: _ -> [w2143]
    shift-right: [w2147] -> _
    shift-left: errorcluster {"status"=FALSE, "code"=0, "source"=""} ("error out") -> [w2141]
    shift-right: [w2146] -> _
    shift-left: w8 -> [w2148]
    i -> [w2140]
    stop <- w2145 stop-if-true
    w2142 = -1  # Timeout
    n819 = call <vilib>:"Parse State Queue__jki_lib_state_machine.vi"("State Queue"=w2148, "Error In (no error)"=w2141) -> ("Remaining States"=w2150:string, "Current State"=w2151:string, "Arguments"=w2149:string)  [unwired: 11 in]
    "GUI" <- w2151
    n820 = case shown="\"\", \"Idle\"" w2151 {
      selector: w2151 -> [_ _ w2618 _ _ _]
      tunnel: w2150 -> [w2152 w2161 w2622 w2641 w2647 w2660]
      tunnel: w2149 -> [_ _ _ _ _ _]
      tunnel: w2143 -> [w2153 w2159 w2620 w2638 w2645 _]
      tunnel: [w2154 w2158 w2624 errorcluster {"status"=FALSE, "code"=0, "source"=""} ("error out") w2644 w2648] -> w2147
      tunnel: w2141 -> [w2154 w2157 w2623 w2631 w2644 w2648]
      tunnel: [w2152 w2160 w2621 w2640 w2646 w2659] -> w2146
      tunnel: [_ _ _ _ TRUE _] -> w2145
      tunnel: [w2153 w2156 w2620 w2638 w2645 w2658] -> w2144
      tunnel: w2142 -> [_ w2155 _ _ _ _]
      frame "ABOUT" {
        # "This state machine handles most of the the UI interrupts in the IDLE case.\n\nClicking on the dryer array elements, changes an invisible bool, which triggers the update to the name associated with\nthe dryer, or viewing the data for that dryer."
      }
      frame "", "Idle" {
        # "executes when the state queue is empty"
        n821 = event shown="[7] \"Robocopy\": Value Change" {
          selector: _ -> [_ _ _ _ _ _ _ _ _ _ _ _ _ _]
          dyn-events: _ -> [_ _ _ _ _ _ _ _ _ _ _ _ _ _]
          timeout: w2155 -> [_ _ _ _ _ _ _ _ _ _ _ _ _ _]
          tunnel: w2161 -> [w2165 w2170 w2180 w2247 w2314 w2381 w2448 w2506 w2525 w2547 w2571 w2607 w2612 w2616]
          tunnel: [w2164 w2169 w2179 w2246 w2313 w2380 w2447 w2506 w2525 w2547 w2571 w2607 w2612 w2616] -> w2160
          tunnel: w2159 -> [w2162 w2167 w2177 w2244 w2311 w2378 w2445 w2507 w2526 w2548 w2572 w2608 w2613 w2617]
          tunnel: [w2163 w2168 w2178 w2245 w2312 w2379 w2446 w2504 w2521 w2545 w2564 w2609 w2611 w2615] -> w2158
          tunnel: w2157 -> [w2163 w2168 w2178 w2245 w2312 w2379 w2446 w2505 w2523 w2546 w2565 w2609 w2611 w2615]
          tunnel: [w2162 w2167 w2177 w2244 w2311 w2378 w2445 w2507 w2526 w2548 w2572 w2608 w2613 w2617] -> w2156
          event Timeout {
            n822 = event-data() -> ()  [unwired: 1 in, 1 out]
            n823 = call <vilib>:"Add State(s) to Queue__jki_lib_state_machine.vi"("State(s) in (\"\")"=w2165) -> ("States Out"=w2164:string)  [unwired: 14 in]
          }
          event "Stop Test": Value Change {
            # "Exit Button Value Change (pressed) Event\n(this executes Macro: Exit to terminate the VI)"
            n824 = event-data() -> ()  [unwired: 1 in, 1 out]
            n825 = call <vilib>:"Add State(s) to Queue__jki_lib_state_machine.vi"("State(s) in Front (\"\")"="Exit", "State(s) in (\"\")"=w2170) -> ("States Out"=w2169:string)  [unwired: 13 in]
          }
          event "GUI Aisle 1": Value Change {
            n826 = event-data() -> ("NewVal"=w2171:T1[])  [unwired: 1 in, 5 out]
            n827 = for {
              tunnel: w2171 -> [w2234] mode=indexing
              tunnel: [w2230] -> w2173
              i -> [w2230]
              stop <- w2231 stop-if-true
              n828 = Unbundle By Name(w2234) -> ("Boolean"=w2233:bool)
              n829 = Equal?(x=w2233, y=TRUE) -> (x = y?=w2231:bool)
            }
            n830 = local read "Station Test State"() -> (w2174:T8[])
            n831 = Array Size(array=w2171) -> (size(s)=w2176:i32)
            n832 = Index Array(array=w2174, index=w2173) -> (element=w2172:T8)
            n833 = Greater?(x=w2176, y=w2173) -> (0:w2175:bool)
            n834 = case shown="True" w2175 {
              tunnel: w2173 -> [_ w2186]
              tunnel: [FALSE ("FileInit") w2190] -> _
              tunnel: w2171 -> [_ w2187]
              tunnel: w2172 -> [_ w2185]
              frame False {
              }
              frame True {
                n835 = local read "Data Sample Filename"() -> (w2188:path)
                n836 = Index Array(array=w2187, index=w2186) -> (element=w2189:T1)
                n837 = call "Panel Dryer Wilt Details.vi"("Dryer In"=w2189, "FileName"=w2188, "Test State"=w2185) -> ("Dryer Details Out"=w2182:T2, "Updated"=w2184:bool, "Audit Alert Out"=w2183:bool)  [unwired: 9 in, 1 out]
                n838 = case shown="True" w2184 {
                  tunnel: [_ w2207] -> w2190
                  tunnel: w2182 -> [_ w2206]
                  tunnel: w2186 -> [_ w2205]
                  tunnel: w2183 -> [_ w2202]
                  frame False {
                    n839 = local read "1"() -> (w2193:T9)
                    n840 = call <vilib>:"Acquire Semaphore.vi"("semaphore"=w2193) -> ("semaphore out"=w2191:T9)  [unwired: 4 in, 2 out]
                    n841 = flat-sequence {
                      tunnel: [w2195] -> w2192
                      tunnel: w2191 -> [w2194]
                      frame #0 {
                        n842 = local read "GUI Aisle 1"() -> (w2197:T1[])
                        n843 = for {
                          tunnel: w2197 -> [w2201] mode=indexing
                          tunnel: [w2199] -> w2196 mode=indexing
                          tunnel: [w2198] -> w2195
                          tunnel: w2194 -> [w2198]
                          n844 = Bundle By Name(cluster=w2201, "Boolean"=FALSE) -> (w2199:T1)
                        }
                        n845 = local write "GUI Aisle 1"(w2196) -> ()
                      }
                    }
                    n846 = call <vilib>:"Release Semaphore.vi"("semaphore"=w2192) -> ()  [unwired: 5 in, 2 out]
                  }
                  frame True {
                    n847 = flat-sequence {
                      tunnel: w2205 -> [w2214]
                      tunnel: w2206 -> [w2215]
                      tunnel: [w2215] -> w2210
                      tunnel: [w2214] -> w2209
                      tunnel: [w2212] -> w2208
                      tunnel: [w2211] -> w2203
                      tunnel: w2202 -> [w2211]
                      tunnel: [w2227] -> w2207
                      tunnel: [w2221] -> w2204
                      tunnel: w2210 -> [w2217]
                      tunnel: w2209 -> [w2223]
                      tunnel: w2208 -> [w2221]
                      tunnel: w2203 -> [w2218]
                      frame #0 {
                        n848 = local read "1"() -> (w2213:T9)
                        n849 = call <vilib>:"Acquire Semaphore.vi"("semaphore"=w2213) -> ("semaphore out"=w2212:T9)  [unwired: 4 in, 2 out]
                      }
                      frame #1 {
                        n850 = local read "GUI Aisle 1"() -> (w2220:T1[])
                        n851 = Index Array(array=w2220, index=w2223) -> (element=w2222:T1)
                        n852 = Unbundle By Name(w2217) -> ("24 Hour Water Injection"=w2216:i32)
                        n853 = case shown="0, Default" w2216 {
                          tunnel: [w2228 TRUE ("Day")] -> w2219
                          frame 0, Default {
                            n854 = local read "Day"() -> (w2228:bool)
                          }
                          frame 1 {
                          }
                        }
                        n855 = call "Update Wilt GUI.vi"("Dryer In"=w2222, "Day Shift?"=w2219, "Enum"=Update_Wilt_GUI_Control."Update Detail Data", "New Dryer Details In"=w2217, "Audit Alert"=w2218) -> ("Dryer Out 2"=w2226:T1, "New Dryer Testing File Init"=w2227:bool)  [unwired: 8 in, 1 out]
                        n856 = Replace Array Subset(array=w2220, new element=w2226, index=w2223) -> (w2225:T1[])
                        n857 = local write "GUI Aisle 1"(w2225) -> ()
                      }
                    }
                    n858 = call <vilib>:"Release Semaphore.vi"("semaphore"=w2204) -> ()  [unwired: 5 in, 2 out]
                  }
                }
              }
            }
            n859 = call <vilib>:"Add State(s) to Queue__jki_lib_state_machine.vi"("State(s) in (\"\")"=w2180) -> ("States Out"=w2179:string)  [unwired: 14 in]
          }
          event "GUI Aisle 1A": Value Change {
            w2238 = 12  # Len of Aisle 1
            n860 = event-data() -> ("NewVal"=w2235:T1[])  [unwired: 1 in, 5 out]
            n861 = local read "Station Test State"() -> (w2241:T8[])
            n862 = Array Size(array=w2235) -> (size(s)=w2243:i32)
            n863 = for {
              tunnel: w2235 -> [w2301] mode=indexing
              tunnel: [w2297] -> w2237
              i -> [w2297]
              stop <- w2298 stop-if-true
              n864 = Unbundle By Name(w2301) -> ("Boolean"=w2300:bool)
              n865 = Equal?(x=w2300, y=TRUE) -> (x = y?=w2298:bool)
            }
            n866 = Delete From Array(array=w2241, length=w2238, index=0) -> (array with subset deleted=w2240:T8[])  [unwired: 1 out]
            n867 = Index Array(array=w2240, index=w2237) -> (element=w2236:T8)
            n868 = Greater?(x=w2243, y=w2237) -> (0:w2242:bool)
            n869 = case shown="True" w2242 {
              tunnel: w2237 -> [_ w2252]
              tunnel: [FALSE ("FileInit") w2257] -> _
              tunnel: w2235 -> [_ w2253]
              tunnel: w2236 -> [_ w2251]
              frame False {
              }
              frame True {
                n870 = local read "Data Sample Filename"() -> (w2254:path)
                n871 = Index Array(array=w2253, index=w2252) -> (element=w2256:T1)
                n872 = call "Panel Dryer Wilt Details.vi"("Dryer In"=w2256, "FileName"=w2254, "Test State"=w2251) -> ("Dryer Details Out"=w2255:T2, "Updated"=w2249:bool, "Audit Alert Out"=w2250:bool)  [unwired: 9 in, 1 out]
                n873 = case shown="True" w2249 {
                  tunnel: [_ w2274] -> w2257
                  tunnel: w2255 -> [_ w2273]
                  tunnel: w2252 -> [_ w2272]
                  tunnel: w2250 -> [_ w2269]
                  frame False {
                    n874 = local read "1A"() -> (w2260:T9)
                    n875 = call <vilib>:"Acquire Semaphore.vi"("semaphore"=w2260) -> ("semaphore out"=w2258:T9)  [unwired: 4 in, 2 out]
                    n876 = flat-sequence {
                      tunnel: [w2262] -> w2259
                      tunnel: w2258 -> [w2261]
                      frame #0 {
                        n877 = local read "GUI Aisle 1A"() -> (w2264:T1[])
                        n878 = for {
                          tunnel: w2264 -> [w2268] mode=indexing
                          tunnel: [w2266] -> w2263 mode=indexing
                          tunnel: [w2265] -> w2262
                          tunnel: w2261 -> [w2265]
                          n879 = Bundle By Name(cluster=w2268, "Boolean"=FALSE) -> (w2266:T1)
                        }
                        n880 = local write "GUI Aisle 1A"(w2263) -> ()
                      }
                    }
                    n881 = call <vilib>:"Release Semaphore.vi"("semaphore"=w2259) -> ()  [unwired: 5 in, 2 out]
                  }
                  frame True {
                    n882 = flat-sequence {
                      tunnel: w2272 -> [w2281]
                      tunnel: w2273 -> [w2282]
                      tunnel: [w2282] -> w2277
                      tunnel: [w2281] -> w2276
                      tunnel: [w2279] -> w2275
                      tunnel: [w2278] -> w2270
                      tunnel: w2269 -> [w2278]
                      tunnel: [w2294] -> w2274
                      tunnel: [w2288] -> w2271
                      tunnel: w2277 -> [w2284]
                      tunnel: w2276 -> [w2290]
                      tunnel: w2275 -> [w2288]
                      tunnel: w2270 -> [w2285]
                      frame #0 {
                        n883 = local read "1A"() -> (w2280:T9)
                        n884 = call <vilib>:"Acquire Semaphore.vi"("semaphore"=w2280) -> ("semaphore out"=w2279:T9)  [unwired: 4 in, 2 out]
                      }
                      frame #1 {
                        n885 = local read "GUI Aisle 1A"() -> (w2287:T1[])
                        n886 = Unbundle By Name(w2284) -> ("24 Hour Water Injection"=w2283:i32)
                        n887 = case shown="0, Default" w2283 {
                          tunnel: [w2295 TRUE ("Day")] -> w2286
                          frame 0, Default {
                            n888 = local read "Day"() -> (w2295:bool)
                          }
                          frame 1 {
                          }
                        }
                        n889 = Index Array(array=w2287, index=w2290) -> (element=w2289:T1)
                        n890 = call "Update Wilt GUI.vi"("Dryer In"=w2289, "Day Shift?"=w2286, "Enum"=Update_Wilt_GUI_Control."Update Detail Data", "New Dryer Details In"=w2284, "Audit Alert"=w2285) -> ("Dryer Out 2"=w2293:T1, "New Dryer Testing File Init"=w2294:bool)  [unwired: 8 in, 1 out]
                        n891 = Replace Array Subset(array=w2287, new element=w2293, index=w2290) -> (w2292:T1[])
                        n892 = local write "GUI Aisle 1A"(w2292) -> ()
                      }
                    }
                    n893 = call <vilib>:"Release Semaphore.vi"("semaphore"=w2271) -> ()  [unwired: 5 in, 2 out]
                  }
                }
              }
            }
            n894 = call <vilib>:"Add State(s) to Queue__jki_lib_state_machine.vi"("State(s) in (\"\")"=w2247) -> ("States Out"=w2246:string)  [unwired: 14 in]
          }
          event "GUI Aisle 2": Value Change {
            w2305 = 20  # Len of Aisle 1+1A
            n895 = event-data() -> ("NewVal"=w2302:T1[])  [unwired: 1 in, 5 out]
            n896 = local read "Station Test State"() -> (w2307:T8[])
            n897 = Array Size(array=w2302) -> (size(s)=w2310:i32)
            n898 = for {
              tunnel: w2302 -> [w2368] mode=indexing
              tunnel: [w2364] -> w2303
              i -> [w2364]
              stop <- w2365 stop-if-true
              n899 = Unbundle By Name(w2368) -> ("Boolean"=w2367:bool)
              n900 = Equal?(x=w2367, y=TRUE) -> (x = y?=w2365:bool)
            }
            n901 = Delete From Array(array=w2307, length=w2305, index=0) -> (array with subset deleted=w2308:T8[])  [unwired: 1 out]
            n902 = Index Array(array=w2308, index=w2303) -> (element=w2304:T8)
            n903 = Greater?(x=w2310, y=w2303) -> (0:w2309:bool)
            n904 = case shown="True" w2309 {
              tunnel: w2303 -> [_ w2319]
              tunnel: [FALSE ("FileInit") w2324] -> _
              tunnel: w2302 -> [_ w2320]
              tunnel: w2304 -> [_ w2318]
              frame False {
              }
              frame True {
                n905 = local read "Data Sample Filename"() -> (w2321:path)
                n906 = Index Array(array=w2320, index=w2319) -> (element=w2323:T1)
                n907 = call "Panel Dryer Wilt Details.vi"("Dryer In"=w2323, "FileName"=w2321, "Test State"=w2318) -> ("Dryer Details Out"=w2322:T2, "Updated"=w2316:bool, "Audit Alert Out"=w2317:bool)  [unwired: 9 in, 1 out]
                n908 = case shown="True" w2316 {
                  tunnel: [_ w2341] -> w2324
                  tunnel: w2322 -> [_ w2340]
                  tunnel: w2319 -> [_ w2339]
                  tunnel: w2317 -> [_ w2336]
                  frame False {
                    n909 = local read "2"() -> (w2327:T9)
                    n910 = call <vilib>:"Acquire Semaphore.vi"("semaphore"=w2327) -> ("semaphore out"=w2326:T9)  [unwired: 4 in, 2 out]
                    n911 = flat-sequence {
                      tunnel: w2326 -> [w2331]
                      tunnel: [w2328] -> w2325
                      frame #0 {
                        n912 = local read "GUI Aisle 2"() -> (w2330:T1[])
                        n913 = for {
                          tunnel: w2330 -> [w2335] mode=indexing
                          tunnel: [w2333] -> w2329 mode=indexing
                          tunnel: [w2332] -> w2328
                          tunnel: w2331 -> [w2332]
                          n914 = Bundle By Name(cluster=w2335, "Boolean"=FALSE) -> (w2333:T1)
                        }
                        n915 = local write "GUI Aisle 2"(w2329) -> ()
                      }
                    }
                    n916 = call <vilib>:"Release Semaphore.vi"("semaphore"=w2325) -> ()  [unwired: 5 in, 2 out]
                  }
                  frame True {
                    n917 = flat-sequence {
                      tunnel: w2339 -> [w2348]
                      tunnel: w2340 -> [w2349]
                      tunnel: [w2349] -> w2344
                      tunnel: [w2348] -> w2343
                      tunnel: [w2346] -> w2342
                      tunnel: [w2345] -> w2337
                      tunnel: w2336 -> [w2345]
                      tunnel: [w2361] -> w2341
                      tunnel: [w2355] -> w2338
                      tunnel: w2344 -> [w2351]
                      tunnel: w2343 -> [w2357]
                      tunnel: w2342 -> [w2355]
                      tunnel: w2337 -> [w2352]
                      frame #0 {
                        n918 = local read "2"() -> (w2347:T9)
                        n919 = call <vilib>:"Acquire Semaphore.vi"("semaphore"=w2347) -> ("semaphore out"=w2346:T9)  [unwired: 4 in, 2 out]
                      }
                      frame #1 {
                        n920 = local read "GUI Aisle 2"() -> (w2354:T1[])
                        n921 = Unbundle By Name(w2351) -> ("24 Hour Water Injection"=w2350:i32)
                        n922 = case shown="0, Default" w2350 {
                          tunnel: [w2362 TRUE ("Day")] -> w2353
                          frame 0, Default {
                            n923 = local read "Day"() -> (w2362:bool)
                          }
                          frame 1 {
                          }
                        }
                        n924 = Index Array(array=w2354, index=w2357) -> (element=w2356:T1)
                        n925 = call "Update Wilt GUI.vi"("Dryer In"=w2356, "Day Shift?"=w2353, "Enum"=Update_Wilt_GUI_Control."Update Detail Data", "New Dryer Details In"=w2351, "Audit Alert"=w2352) -> ("Dryer Out 2"=w2360:T1, "New Dryer Testing File Init"=w2361:bool)  [unwired: 8 in, 1 out]
                        n926 = Replace Array Subset(array=w2354, new element=w2360, index=w2357) -> (w2359:T1[])
                        n927 = local write "GUI Aisle 2"(w2359) -> ()
                      }
                    }
                    n928 = call <vilib>:"Release Semaphore.vi"("semaphore"=w2338) -> ()  [unwired: 5 in, 2 out]
                  }
                }
              }
            }
            n929 = call <vilib>:"Add State(s) to Queue__jki_lib_state_machine.vi"("State(s) in (\"\")"=w2314) -> ("States Out"=w2313:string)  [unwired: 14 in]
          }
          event "GUI Aisle 3": Value Change {
            w2372 = 32  # Len of Aisle 1+1A+2
            n930 = event-data() -> ("NewVal"=w2369:T1[])  [unwired: 1 in, 5 out]
            n931 = Array Size(array=w2369) -> (size(s)=w2377:i32)
            n932 = for {
              tunnel: w2369 -> [w2435] mode=indexing
              tunnel: [w2431] -> w2371
              i -> [w2431]
              stop <- w2432 stop-if-true
              n933 = Unbundle By Name(w2435) -> ("Boolean"=w2434:bool)
              n934 = Equal?(x=w2434, y=TRUE) -> (x = y?=w2432:bool)
            }
            n935 = local read "Station Test State"() -> (w2374:T8[])
            n936 = Delete From Array(array=w2374, length=w2372, index=0) -> (array with subset deleted=w2375:T8[])  [unwired: 1 out]
            n937 = Index Array(array=w2375, index=w2371) -> (element=w2370:T8)
            n938 = Greater?(x=w2377, y=w2371) -> (0:w2376:bool)
            n939 = case shown="True" w2376 {
              tunnel: w2371 -> [_ w2386]
              tunnel: [FALSE ("FileInit") w2391] -> _
              tunnel: w2369 -> [_ w2387]
              tunnel: w2370 -> [_ w2385]
              frame False {
              }
              frame True {
                n940 = local read "Data Sample Filename"() -> (w2388:path)
                n941 = Index Array(array=w2387, index=w2386) -> (element=w2390:T1)
                n942 = call "Panel Dryer Wilt Details.vi"("Dryer In"=w2390, "FileName"=w2388, "Test State"=w2385) -> ("Dryer Details Out"=w2389:T2, "Updated"=w2383:bool, "Audit Alert Out"=w2384:bool)  [unwired: 9 in, 1 out]
                n943 = case shown="True" w2383 {
                  tunnel: [_ w2408] -> w2391
                  tunnel: w2389 -> [_ w2407]
                  tunnel: w2386 -> [_ w2406]
                  tunnel: w2384 -> [_ w2404]
                  frame False {
                    n944 = local read "3"() -> (w2394:T9)
                    n945 = call <vilib>:"Acquire Semaphore.vi"("semaphore"=w2394) -> ("semaphore out"=w2392:T9)  [unwired: 4 in, 2 out]
                    n946 = flat-sequence {
                      tunnel: [w2396] -> w2393
                      tunnel: w2392 -> [w2395]
                      frame #0 {
                        n947 = local read "GUI Aisle 3"() -> (w2398:T1[])
                        n948 = for {
                          tunnel: w2398 -> [w2402] mode=indexing
                          tunnel: [w2400] -> w2397 mode=indexing
                          tunnel: [w2399] -> w2396
                          tunnel: w2395 -> [w2399]
                          n949 = Bundle By Name(cluster=w2402, "Boolean"=FALSE) -> (w2400:T1)
                        }
                        n950 = local write "GUI Aisle 3"(w2397) -> ()
                      }
                    }
                    n951 = call <vilib>:"Release Semaphore.vi"("semaphore"=w2393) -> ()  [unwired: 5 in, 2 out]
                  }
                  frame True {
                    n952 = flat-sequence {
                      tunnel: w2406 -> [w2415]
                      tunnel: w2407 -> [w2416]
                      tunnel: [w2416] -> w2411
                      tunnel: [w2415] -> w2410
                      tunnel: [w2413] -> w2409
                      tunnel: w2404 -> [w2412]
                      tunnel: [w2412] -> w2403
                      tunnel: [w2428] -> w2408
                      tunnel: [w2422] -> w2405
                      tunnel: w2411 -> [w2418]
                      tunnel: w2410 -> [w2424]
                      tunnel: w2409 -> [w2422]
                      tunnel: w2403 -> [w2419]
                      frame #0 {
                        n953 = local read "3"() -> (w2414:T9)
                        n954 = call <vilib>:"Acquire Semaphore.vi"("semaphore"=w2414) -> ("semaphore out"=w2413:T9)  [unwired: 4 in, 2 out]
                      }
                      frame #1 {
                        n955 = Unbundle By Name(w2418) -> ("24 Hour Water Injection"=w2417:i32)
                        n956 = case shown="0, Default" w2417 {
                          tunnel: [w2429 TRUE ("Day")] -> w2420
                          frame 0, Default {
                            n957 = local read "Day"() -> (w2429:bool)
                          }
                          frame 1 {
                          }
                        }
                        n958 = local read "GUI Aisle 3"() -> (w2421:T1[])
                        n959 = Index Array(array=w2421, index=w2424) -> (element=w2423:T1)
                        n960 = call "Update Wilt GUI.vi"("Dryer In"=w2423, "Day Shift?"=w2420, "Enum"=Update_Wilt_GUI_Control."Update Detail Data", "New Dryer Details In"=w2418, "Audit Alert"=w2419) -> ("Dryer Out 2"=w2427:T1, "New Dryer Testing File Init"=w2428:bool)  [unwired: 8 in, 1 out]
                        n961 = Replace Array Subset(array=w2421, new element=w2427, index=w2424) -> (w2426:T1[])
                        n962 = local write "GUI Aisle 3"(w2426) -> ()
                      }
                    }
                    n963 = call <vilib>:"Release Semaphore.vi"("semaphore"=w2405) -> ()  [unwired: 5 in, 2 out]
                  }
                }
              }
            }
            n964 = call <vilib>:"Add State(s) to Queue__jki_lib_state_machine.vi"("State(s) in (\"\")"=w2381) -> ("States Out"=w2380:string)  [unwired: 14 in]
          }
          event "GUI Aisle 4": Value Change {
            w2439 = 44  # Len of Aisle 1+1A+2+3
            # "Update assumes that the bool has been\nset.  Looks for that element."
            n965 = event-data() -> ("NewVal"=w2436:T1[])  [unwired: 1 in, 5 out]
            n966 = Array Size(array=w2436) -> (size(s)=w2444:i32)
            n967 = for {
              tunnel: w2436 -> [w2502] mode=indexing
              tunnel: [w2498] -> w2438
              i -> [w2498]
              stop <- w2499 stop-if-true
              n968 = Unbundle By Name(w2502) -> ("Boolean"=w2501:bool)
              n969 = Equal?(x=w2501, y=TRUE) -> (x = y?=w2499:bool)
            }
            n970 = local read "Station Test State"() -> (w2441:T8[])
            n971 = Delete From Array(array=w2441, length=w2439, index=0) -> (array with subset deleted=w2442:T8[])  [unwired: 1 out]
            n972 = Index Array(array=w2442, index=w2438) -> (element=w2437:T8)
            n973 = Greater?(x=w2444, y=w2438) -> (0:w2443:bool)
            n974 = case shown="True" w2443 {
              tunnel: w2438 -> [_ w2453]
              tunnel: [FALSE ("FileInit") w2458] -> _
              tunnel: w2436 -> [_ w2454]
              tunnel: w2437 -> [_ w2452]
              frame False {
              }
              frame True {
                n975 = local read "Data Sample Filename"() -> (w2455:path)
                n976 = Index Array(array=w2454, index=w2453) -> (element=w2457:T1)
                n977 = call "Panel Dryer Wilt Details.vi"("Dryer In"=w2457, "FileName"=w2455, "Test State"=w2452) -> ("Dryer Details Out"=w2456:T2, "Updated"=w2450:bool, "Audit Alert Out"=w2451:bool)  [unwired: 9 in, 1 out]
                n978 = case shown="True" w2450 {
                  tunnel: [_ w2475] -> w2458
                  tunnel: w2456 -> [_ w2474]
                  tunnel: w2453 -> [_ w2473]
                  tunnel: w2451 -> [_ w2470]
                  frame False {
                    n979 = local read "4"() -> (w2461:T9)
                    n980 = call <vilib>:"Acquire Semaphore.vi"("semaphore"=w2461) -> ("semaphore out"=w2459:T9)  [unwired: 4 in, 2 out]
                    n981 = flat-sequence {
                      tunnel: [w2463] -> w2460
                      tunnel: w2459 -> [w2462]
                      frame #0 {
                        n982 = local read "GUI Aisle 4"() -> (w2465:T1[])
                        n983 = for {
                          tunnel: w2465 -> [w2469] mode=indexing
                          tunnel: [w2467] -> w2464 mode=indexing
                          tunnel: [w2466] -> w2463
                          tunnel: w2462 -> [w2466]
                          n984 = Bundle By Name(cluster=w2469, "Boolean"=FALSE) -> (w2467:T1)
                        }
                        n985 = local write "GUI Aisle 4"(w2464) -> ()
                      }
                    }
                    n986 = call <vilib>:"Release Semaphore.vi"("semaphore"=w2460) -> ()  [unwired: 5 in, 2 out]
                  }
                  frame True {
                    n987 = flat-sequence {
                      tunnel: w2473 -> [w2482]
                      tunnel: w2474 -> [w2483]
                      tunnel: [w2483] -> w2478
                      tunnel: [w2482] -> w2477
                      tunnel: [w2480] -> w2476
                      tunnel: [w2479] -> w2471
                      tunnel: w2470 -> [w2479]
                      tunnel: [w2495] -> w2475
                      tunnel: [w2489] -> w2472
                      tunnel: w2478 -> [w2485]
                      tunnel: w2477 -> [w2491]
                      tunnel: w2476 -> [w2489]
                      tunnel: w2471 -> [w2486]
                      frame #0 {
                        n988 = local read "4"() -> (w2481:T9)
                        n989 = call <vilib>:"Acquire Semaphore.vi"("semaphore"=w2481) -> ("semaphore out"=w2480:T9)  [unwired: 4 in, 2 out]
                      }
                      frame #1 {
                        n990 = Unbundle By Name(w2485) -> ("24 Hour Water Injection"=w2484:i32)
                        n991 = local read "GUI Aisle 4"() -> (w2488:T1[])
                        n992 = case shown="0, Default" w2484 {
                          tunnel: [w2496 TRUE ("Day")] -> w2487
                          frame 0, Default {
                            n993 = local read "Day"() -> (w2496:bool)
                          }
                          frame 1 {
                          }
                        }
                        n994 = Index Array(array=w2488, index=w2491) -> (element=w2490:T1)
                        n995 = call "Update Wilt GUI.vi"("Dryer In"=w2490, "Day Shift?"=w2487, "Enum"=Update_Wilt_GUI_Control."Update Detail Data", "New Dryer Details In"=w2485, "Audit Alert"=w2486) -> ("Dryer Out 2"=w2494:T1, "New Dryer Testing File Init"=w2495:bool)  [unwired: 8 in, 1 out]
                        n996 = Replace Array Subset(array=w2488, new element=w2494, index=w2491) -> (w2493:T1[])
                        n997 = local write "GUI Aisle 4"(w2493) -> ()
                      }
                    }
                    n998 = call <vilib>:"Release Semaphore.vi"("semaphore"=w2472) -> ()  [unwired: 5 in, 2 out]
                  }
                }
              }
            }
            n999 = call <vilib>:"Add State(s) to Queue__jki_lib_state_machine.vi"("State(s) in (\"\")"=w2448) -> ("States Out"=w2447:string)  [unwired: 14 in]
          }
          event "Robocopy": Value Change {
            n1000 = event-data() -> ()  [unwired: 1 in, 6 out]
            n1001 = local read "exe?"() -> (w2503:bool)
            n1002 = case shown="True" w2503 {
              tunnel: w2505 -> [w2508 w2510]
              tunnel: [w2508 w2509] -> w2504
              frame False {
              }
              frame True {
                n1003 = flat-sequence {
                  tunnel: w2510 -> [w2518]
                  tunnel: [w2515] -> w2511
                  tunnel: [w2519] -> w2509
                  tunnel: w2511 -> [w2519]
                  frame #0 {
                  }
                  frame #1 {
                    w2514 = TRUE ("run minimized? (F)")
                    w2513 = FALSE ("wait until completion? (T)")
                    n1004 = call <vilib>:"System Exec.vi"("run minimized? (F)"=w2514, "wait until completion? (T)"=w2513, "error in (no error)"=w2518, "command line"="Robocopy Location") -> ("error out"=w2516:errorcluster)  [unwired: 4 in, 3 out]
                    n1005 = call <vilib>:"System Exec.vi"("run minimized? (F)"=w2514, "wait until completion? (T)"=w2513, "error in (no error)"=w2516, "command line"="Daily Summary") -> ("error out"=w2515:errorcluster)  [unwired: 4 in, 3 out]
                  }
                  frame #2 {
                    n1006 = local write "Robocopy"(FALSE ("Stop Test 2")) -> ()
                  }
                }
              }
            }
          }
          event "Resend Start": Value Change {
            n1007 = event-data() -> ()  [unwired: 1 in, 6 out]
            n1008 = flat-sequence {
              tunnel: w2523 -> [w2532]
              tunnel: [w2533] -> w2522
              tunnel: [w2542] -> w2524
              tunnel: w2522 -> [w2542]
              frame #0 {
                n1009 = local write "WriteOK"(FALSE ("WriteOK")) -> ()
              }
              frame #1 {
                n1010 = local read "All Confgured Com Array"() -> (w2529:u8[])
                n1011 = local read "Station Labels"() -> (w2528:string[])
                n1012 = call "Panel Resend Start.vi"("All Confgured Com Array"=w2529, "Station Labels"=w2528) -> ("Com Port"=w2530:dbl, "Resend"=w2531:bool)  [unwired: 15 in, 1 out]
                n1013 = case shown="True" w2531 {
                  tunnel: [w2534 w2539] -> w2533
                  tunnel: w2532 -> [w2534 w2538]
                  tunnel: w2530 -> [_ w2537]
                  frame False {
                  }
                  frame True {
                    n1014 = To Unsigned Byte Integer(number=w2537) -> (unsigned 8bit integer=w2536:u8)
                    n1015 = call "Com Chan Type Conversion.vi"("Com Chan"=w2536) -> ("VISA resource name"=w2540:refnum<visa-resource-name>)  [unwired: 11 in, 3 out]
                    n1016 = call "GEA2_ICP_Dryer_SM.vi"("ComPort"=w2540, "Mode"=GEA2_Dryer_Interface_Ctrl."Send WILT Startup CMDs", "Error In"=w2538) -> ("WriteOK"=→"WriteOK":bool, "Error Out"=w2539:errorcluster)  [unwired: 7 in, 4 out]
                  }
                }
              }
              frame #2 {
                n1017 = local write "UI error out"(w2542) -> ()
                n1018 = local write "Resend Start"(FALSE ("Stop Test 2")) -> ()
              }
            }
            n1019 = call <vilib>:"Clear Errors.vi"("error in (no error)"=w2524) -> ("error out"=w2521:errorcluster)  [unwired: 6 in]
          }
          event "Stop All": Value Change {
            n1020 = event-data() -> ()  [unwired: 1 in, 6 out]
            n1021 = flat-sequence {
              tunnel: w2546 -> [w2551]
              tunnel: [w2549] -> w2544
              tunnel: [w2562] -> w2545
              tunnel: w2544 -> [w2562]
              frame #0 {
              }
              frame #1 {
                # "Shutdown newfi dryers"
                n1022 = for {
                  N: 2 -> [_]
                  tunnel: w2551 -> [w2554]
                  tunnel: [w2553] -> w2549
                  n1023 = Wait (ms)(milliseconds to wait=u32 50) -> ()  [unwired: 1 out]
                  n1024 = local read "All Confgured Com Array"() -> (w2555:u8[])
                  n1025 = for {
                    tunnel: w2555 -> [w2559] mode=indexing
                    tunnel: w2554 -> [w2557]
                    tunnel: [w2556] -> w2553
                    w2558 = T19 7 items=["CMD_Eval_Mode_Entry_CC1", "CMD_Eval_Mode_Entry_CC2", "CMD_Eval_Mode_Continue", "CMD_Send_DIAG_Info", "CMD_Enable_Debug_Log ", "CMD_Disable_Debug_Log ", "CMD_Send_Log_Data", "CMD_Stop", "RQST_Version"] ("Command")
                    n1026 = call "Com Chan Type Conversion.vi"("Com Chan"=w2559) -> ("VISA resource name"=w2560:refnum<visa-resource-name>)  [unwired: 11 in, 3 out]
                    n1027 = call "GEA2_ICP_Dryer_SM.vi"("ComPort"=w2560, "Mode"=GEA2_Dryer_Interface_Ctrl."SendCMD", "Error In"=w2557, "Command"=w2558) -> ("Error Out"=w2556:errorcluster)  [unwired: 6 in, 5 out]
                    "Error Stop All" <- w2556
                  }
                }
              }
              frame #2 {
                n1028 = local write "UI error out"(w2562) -> ()
                n1029 = local write "Stop All"(FALSE ("Stop Test 2")) -> ()
              }
            }
          }
          event "Day": Value Change {
            w2569 = string[][] [["Station", "LabID", "TR", "Cycle Count Day", "Cycle Count Night", "Time On Day", "Time On Night", "Total Run Time", "Notes"]]  # Summary Data Header
            # "Write Log File"
            n1030 = event-data() -> ()  [unwired: 1 in, 6 out]
            n1031 = local read "All Test Stations"() -> (w2570:T1[])
            n1032 = for {
              tunnel: w2570 -> [w2583] mode=indexing
              shift-right: [w2575] -> w2567
              shift-left: w2569 -> [w2574]
              n1033 = Unbundle By Name(w2583) -> ("Station Label"=w2579:string, "Lab ID"=w2580:string, "Dryer Details.TR Number"=w2578:string, "Dryer Details.Cycle Count Day"=w2577:string, "Dryer Details.Cycle Count Night"=w2576:string, "Dryer Details.Time On Day"=w2582:string, "Dryer Details.Time On Night"=w2581:string, "Dryer Details.Notes"=w2573:string)
              n1034 = case shown="\"True\", Default" w2580 {
                selector: w2580 -> [_ w2596]
                tunnel: w2582 -> [_ w2592]
                tunnel: w2581 -> [_ w2591]
                tunnel: w2579 -> [_ w2586]
                tunnel: w2578 -> [_ w2595]
                tunnel: w2577 -> [_ w2594]
                tunnel: w2576 -> [_ w2593]
                tunnel: [w2584 w2588] -> w2575
                tunnel: w2574 -> [w2584 w2587]
                tunnel: w2573 -> [_ w2585]
                frame "" {
                }
                frame "True", Default {
                  n1035 = call "Type Conv Seconds - Time String.vi"("Time String In"=w2591) -> ("Seconds Out"=w2598:dbl)  [unwired: 9 in, 1 out]
                  n1036 = call "Type Conv Seconds - Time String.vi"("Time String In"=w2592) -> ("Seconds Out"=w2599:dbl)  [unwired: 9 in, 1 out]
                  n1037 = Add(x=w2599, y=w2598) -> (x+y=w2597:dbl)
                  n1038 = call "Type Conv Seconds - Time String.vi"("Seconds In"=w2597) -> ("Time String Out"=w2590:string)  [unwired: 9 in, 1 out]
                  n1039 = Build Array(w2586, w2596, w2595, w2594, w2593, w2592, w2591, w2590, w2585) -> (w2589:string[])
                  n1040 = Build Array (concatenate)(w2587, w2589) -> (w2588:string[][])
                }
              }
            }
            n1041 = local read "Data Sample Directory"() -> (w2568:path)
            n1042 = call "File Path Generate and Write Wilt.vi"("Use Day In Path"=FALSE, "error in"=w2565, "Data Array"=w2567, "base path"=w2568) -> ("error out"=w2564:errorcluster)  [unwired: 6 in, 1 out]
          }
          event "Aisle 2 (21-32)", "Aisle 3 (33-44)", "Aisle 1 (1-20)", "Aisle 4 (45-56)": Value Change {
            # "Save watering times on change."
            n1043 = event-data() -> ()  [unwired: 1 in, 6 out]
            n1044 = local read "Water Times Filepath"() -> (w2601:path)
            n1045 = local read "Aisle 2 (21-32)"() -> (w2605:dbl[])
            n1046 = local read "Aisle 4 (45-56)"() -> (w2603:dbl[])
            n1047 = local read "Aisle 1 (1-20)"() -> (w2606:dbl[])
            n1048 = local read "Aisle 3 (33-44)"() -> (w2604:dbl[])
            n1049 = Build Array (concatenate)(w2606, w2605, w2604, w2603) -> (w2602:dbl[])
            n1050 = call-poly <vilib>:"Write To Spreadsheet File.vi"("delimiter (\\t)"="," ("delimiter (\\t)"), "1D data"=w2602, "file path (dialog if empty)"=w2601) -> ()  [unwired: 5 in, 1 out]
          }
          event "Settings": Value Change {
            n1051 = event-data() -> ()  [unwired: 1 in, 6 out]
            n1052 = local write "Tab Control 2"(enum32{"Configuration", "Main"}."Configuration" ("Tab Control 2")) -> ()
          }
          event "Back Button": Value Change {
            n1053 = event-data() -> ()  [unwired: 1 in, 6 out]
            n1054 = local write "Tab Control 2"(enum32{"Configuration", "Main"}."Main" ("Tab Control 2")) -> ()
          }
        }
      }
      frame Default {
        w2627 = 42 items=["No error", "Argument error", "Memory is full", "Out of zone", "End of file", "File already open", "Generic file I/O error", "File not found", "File permission error", "Disk is full", "Duplicate path", "Too many files open", "System feature not enabled", "Resource file not found", "Cannot add resource", "Resource not found", "Image not found", "Image memory error", "Pen does not exist", "Config type invalid", "Config token not found", "Config parse error", "Config memory error", "Bad external code format", "Bad external code offset", "External code not present", "Null window", "Destroy window error", "Null menu", "Print aborted", "Bad print record", "Print driver error", "Windows error during printing", "Memory error during printing", "Print dialog error", "Generic print error", "Invalid device refnum", "Device not found", "Device parameter error", "Device unit error", "Cannot open device", "Device call aborted", "Generic error", "Cancelled by user", "Object ID too low", "Object ID too high", "Object not in heap", "Unknown heap", "Unknown object (invalid DefProc)", "Unknown object (DefProc not in table)", "Message out of range", "Invalid (null) method", "Unknown message", "Manager call not supported", "Bad address", "Network operation in progress", "Network operation timed out", "Connection is busy", "Network attribute not supported", "Network error", "Address in use", "System out of memory", "Connection aborted", "Connection refused", "Not connected", "Already connected", "Connection closed", "Initialization error (interapplication manager)", "Bad occurrence", "Wait on unbound occurrence handler", "Occurrence queue overflow", "Datalog type conflict", "Unused", "Unrecognized type (interapplication manager)", "Memory corrupt", "Failed to make temporary DLL", "Old CIN version", "Drag socket not found", "Failed to load drop-object", "Failed to register OLE object", "Failed to release OLE object", "Format specifier type mismatch", "Unknown format specifier", "Too few format specifiers", "Too many format specifiers", "Scan failed", "Newer CIN version", "Error converting to variant", "Runtime menu error", "Password tampered", "Variant attribute not found", "Incompatible variant data type", "Event data is not available", "Event Store is not present", "Occurrence is not found", "Event Queue is not created", "Event info is not available", "Refnum passed is NULL", "Error retrieving Class GUID", "Error retrieving CoClass GUID", "Error retrieving TypeLib GUID.", "Bad built application magic bytes.", "Specific driver is different from the specific driver associated with the Logical Name.", "There is no session opened to the class driver.", "Max Error", "MAX - Error with config objects", "MAX - Error loading configuration", "MAX - Group not supported"]
        # "Current State"
        # "Do not delete, rename, or modify this frame.\n(this is used to capture unhandled states and typos)"
        # "Handle mistyped state name (developer tool)"
        n1055 = Format Into String(format string="Software Exception: Unhandled State \"%s\"." ("message"), error in=w2623, w2618) -> (resulting string=w2626:string, error out=w2625:errorcluster)  [unwired: 1 in]
        n1056 = call <vilib>:"Error Cluster From Error Code.vi"("show call chain? (False)"=TRUE, "error in (no error)"=w2625, "error message (\"\")"=w2626, "error code (0)"=w2627) -> ("error out"=w2624:errorcluster)  [unwired: 5 in]
        n1057 = call <vilib>:"Add State(s) to Queue__jki_lib_state_machine.vi"("State(s) in (\"\")"=w2622) -> ("States Out"=w2621:string)  [unwired: 14 in]
      }
      frame "Error Handler" {
        # "Handle any errors here.\nYou can also output any states to clean-up after errors occur"
        # "Clear error"
        n1058 = local read "Debug"() -> (w2629:bool)
        n1059 = case shown="True" w2629 {
          tunnel: w2631 -> [_ w2642]
          frame False {
          }
          frame True {
            # "Unhandled Error -- Display it"
            n1060 = call <vilib>:"General Error Handler.vi"("error in (no error)"=w2642) -> ()  [unwired: 10 in, 5 out]
          }
        }
        n1061 = Unbundle By Name(w2631) -> ("source"=w2630:string)
        n1062 = local read "UI Error List"() -> (w2636:string)
        n1063 = Concatenate Strings("ErrorUI: " ("string"), w2630) -> (w2633:string)
        n1064 = Concatenate Strings(w2630, "\n", w2636) -> (→"UI Error List":string)
        n1065 = local write "User Notice"(w2633) -> ()
        n1066 = call <vilib>:"Add State(s) to Queue__jki_lib_state_machine.vi"("State(s) in Front (\"\")"="/* Post Error States", "State(s) in (\"\")"=w2641) -> ("States Out"=w2640:string)  [unwired: 13 in]
        "UI error out" <- w2631
      }
      frame "Exit" {
        # "Do not put any code in this frame.\n(No errors that occur here will be handled.)"
        n1067 = call <vilib>:"Add State(s) to Queue__jki_lib_state_machine.vi"("State(s) in (\"\")"=w2647) -> ("States Out"=w2646:string)  [unwired: 14 in]
      }
      frame "Data: Init" {
        n1068 = local write "Error Stop All"(w2648) -> ()
        n1069 = flat-sequence {
          tunnel: [w2662] -> w2650
          tunnel: [w2674] -> w2657
          tunnel: [w2673] -> w2656
          tunnel: [w2672] -> w2655
          tunnel: [w2671] -> w2654
          tunnel: [w2670] -> w2653
          tunnel: ["Dryer To Save"] -> w2652
          tunnel: [w2675] -> w2651
          tunnel: w2650 -> [w2675]
          frame #0 {
            n1070 = while {
              tunnel: [w2663] -> w2662
              stop <- w2668 stop-if-true
              n1071 = local read "Gathering Data Latch"() -> (w2664:bool)
              n1072 = local read "Test Complete"() -> (w2663:bool)
              n1073 = local read "Init Complete"() -> (w2665:bool)
              n1074 = To Unsigned Long Integer(number="DAQ Delay") -> (unsigned 32bit integer=w2667:u32)
              n1075 = Wait (ms)(milliseconds to wait=w2667) -> ()  [unwired: 1 out]
              n1076 = And(x=w2664, y=w2665) -> (x .and. y?=w2666:bool)
              n1077 = Or(x=w2666, y=w2663) -> (x .or. y?=w2668:bool)
            }
          }
          frame #1 {
            n1078 = local read "GUI Aisle 1A"() -> (w2673:T1[])
            n1079 = local read "GUI Aisle 1"() -> (w2674:T1[])
            n1080 = local read "GUI Aisle 2"() -> (w2672:T1[])
            n1081 = local read "GUI Aisle 3"() -> (w2671:T1[])
            n1082 = local read "GUI Aisle 4"() -> (w2670:T1[])
          }
        }
        n1083 = Bundle("GUI Aisle 1"=w2657, "GUI Aisle 1A"=w2656, "GUI Aisle 2"=w2655, "GUI Aisle 3"=w2654, "GUI Aisle 4"=w2653, "Dryer To Save"=w2652) -> (w2658:T20)  [unwired: 1 in]
        n1084 = case shown="False" w2651 {
          tunnel: [_ "Exit" ("State(s) in Front (\"\")")] -> w2649
          frame False {
          }
          frame True {
          }
        }
        n1085 = call <vilib>:"Add State(s) to Queue__jki_lib_state_machine.vi"("State(s) in Front (\"\")"=w2649, "State(s) in (\"\")"=w2660) -> ("States Out"=w2659:string)  [unwired: 13 in]
      }
    }
    "UI Events" <- w2140
  }
  n1086 = Not(x=w6) -> (.not. x?=w7:bool)
  n1087 = property on="Test Complete" class="Bool (strict)"("Val(Sgnl)"=w6) -> ()  [unwired: 2 in, 2 out]
  n1088 = local write "Stop Test"(w7) -> ()
